vi "nanocal -- nuclear schottky fit V3.vi"() -> ()   [LabVIEW 2020]
uses:
  filename-pattern.ctl
  show-win- control.ctl
  cursor winow.ctl
  nanocal-goodness-weighting-strategy.ctl
  <vilib>/gmath/NumericalOptimization/stopping criteria.ctl
  3-lorentzian-parameters.ctl
  cursor window action.ctl
  3-lorentzian-heat-response action.ctl
  cursor action.ctl
  2Dwindow.ctl
  publisher action.ctl
  mathematica string map action.ctl
  <vilib>/gmath/NumericalOptimization/objective function data.ctl
  3-lorentzian-parameters -- action.ctl
  filename-action.ctl
  <vilib>/Utility/miscctls.llb/LVMapReplaceAction.ctl
  file -- read-write control.ctl
  array -- freq-voltage transformations action.ctl
  KM_file -- read-write control.ctl
  replace cursor action stack.vi
  Q -- range multiplier -- real -- V2.vi
  Q - not nan and gtr than zero - Real.vi
  Q - not nan -- real.vi
  Q -- check range -- i -- real.vi
  array - smart min max.vi
  3-lorentzian-heat-response -- V4.vi/142dd4c5-f9ed-c64b-bc14-a88e3e2c450a.vi
  3-lorentzian-heat-response -- analytic derivatives V3.vi
  array -- integrate scalar product.vi
  3-lorentzian-heat-response -- analytic derivatives -- grad and curvature -- V4.vi
  array -- freq-voltage transformations.vi/05c44075-957c-bc42-b6fa-2799d0bc0485.vi
  tale of three indices.vi
  filter -- window span logic.vi
  linear interp iiii- complex - z-omega - divide.vi
  linear interpolation iiii- complex.vi
  containing bix.vi
  3-lorentzian-heat-response.vi/142dd4c5-f9ed-c64b-bc14-a88e3e2c450a.vi
  <vilib>/Array/Sort 2D Array - Pop Stack.vi
  <vilib>/Array/Sort 2D Array - Push Stack.vi
  array -- freq-voltage transformations.vi/05c44075-957c-bc42-b6fa-2799d0bc0485.vi/5dd0d2be-718e-c148-b8fa-e083cdba2843.vi
  array -- freq-voltage transformations.vi/05c44075-957c-bc42-b6fa-2799d0bc0485.vi/095795a0-771d-c341-9fed-d90d2e44c51c.vi
  command stack.vi
  tale of three indices -- check state.vi
  Q -- check range -- i -- integer.vi
  linear interp iiii- complex - z-omega.vi
  line -- complex.vi
  Q - not nan -- integer.vi
  <vilib>/Analysis/baseanly.llb/A x B.vi
  <vilib>/Analysis/baseanly.llb/Complex A x B.vi
  array -- 3-finitediff.vi
  <vilib>/Analysis/polynomials.llb/Multiply Polynomials.vi
  <vilib>/Analysis/polynomials.llb/Multiply Polynomials (DBL).vi
  <vilib>/Analysis/polynomials.llb/Polynomial Roots.vi
  <vilib>/Analysis/polynomials.llb/Polynomial Roots (DBL).vi
  <vilib>/gmath/NumericalOptimization/Quasi Newton.vi
  <vilib>/Analysis/Matrix/Numeric/Conversions/Array To Matrix.vi
  <vilib>/Analysis/Matrix/Numeric/Conversions/Array To Matrix - RA2.vi
  <vilib>/Analysis/baseanly.llb/Inverse Matrix.vi
  <vilib>/Analysis/baseanly.llb/Real Inverse Matrix.vi
  <vilib>/Comparison/Less/Less Functor/Less Functor.lvclass
  <vilib>/gmath/NI_Gmath.lvlib
panel:
  in  "Map OUT":map{T1, dbl}(c390)
  in  "strings stuff tab":T2(tab)
  in  "string IN":string="  48 ->   <| \"ζ\"->  0.218787747977  , \"τ1\"-> 0.031456659327  , \"τS\"-> 0.269139973017  , \"τN\"-> 0.256714789857  , \"τC\"-> 0.001257909269  , \"κ0\"-> 0.000000000759  , \"mm1\"-> 0.000225096911  , \"mm2\"-> 0.015739660310  , \"mm3\"-> 0.657655153581  , \"T\"->  0.148000000000  , \"B\"-> 12.000000000000  , \"θ\"-> 0.000000000000  |>   , \r49 ->   <| \"ζ\"->  0.166979764431  , \"τ1\"-> 0.018942043621  , \"τS\"-> 0.110758885907  , \"τN\"-> 0.187535940807  , \"τC\"-> 0.001145519942  , \"κ0\"-> 0.000000001049  , \"mm1\"-> 0.000162653882  , \"mm2\"-> 0.006830646180  , \"mm3\"-> 0.361198290111  , \"T\"->  0.179000000000  , \"B\"-> 12.000000000000  , \"θ\"-> 0.000000000000  |>   , \r50 ->   <| \"ζ\"->  0.129670961314  , \"τ1\"-> 0.021089937696  , \"τS\"-> 0.112692124493  , \"τN\"-> 0.107228011320  , \"τC\"-> 0.001403544000  , \"κ0\"-> 0.000000001212  , \"mm1\"-> 0.000159537518  , \"mm2\"-> 0.010413685343  , \"mm3\"-> 0.260357650071  , \"T\"->  0.197000000000  , \"B\"-> 12.000000000000  , \"θ\"-> 0.000000000000  |>   , \r51 ->   <| \"ζ\"->  0.079034359832  , \"τ1\"-> 0.025346839295  , \"τS\"-> 0.089984085428  , \"τN\"-> 0.031717364329  , \"τC\"-> 0.001567096624  , \"κ0\"-> 0.000000001542  , \"mm1\"-> 0.000113086552  , \"mm2\"-> 0.017802249564  , \"mm3\"-> 0.140318645732  , \"T\"->  0.250000000000  , \"B\"-> 12.000000000000  , \"θ\"-> 0.000000000000  |>   , \r52 ->   <| \"ζ\"->  0.054397810218  , \"τ1\"-> 0.023191672440  , \"τS\"-> 0.068776102177  , \"τN\"-> 0.016667714610  , \"τC\"-> 0.001951070520  , \"κ0\"-> 0.000000001955  , \"mm1\"-> 0.000098147963  , \"mm2\"-> 0.017702409099  , \"mm3\"-> 0.097433959215  , \"T\"->  0.300000000000  , \"B\"-> 12.000000000000  , \"θ\"-> 0.000000000000  |>   , \r53 ->   <| \"ζ\"->  0.039475039748  , \"τ1\"-> 0.021602230815  , \"τS\"-> 0.055852925082  , \"τN\"-> 0.008163813050  , \"τC\"-> 0.002520091738  , \"κ0\"-> 0.000000002417  , \"mm1\"-> 0.000091858515  , \"mm2\"-> 0.018006002388  , \"mm3\"-> 0.072568263064  , \"T\"->  0.360000000000  , \"B\"-> 12.000000000000  , \"θ\"-> 0.000000000000  |>   , \r54 ->   <| \"ζ\"->  0.031945976845  , \"τ1\"-> 0.019000922826  , \"τS\"-> 0.045624146388  , \"τN\"-> 0.005314716063  , \"τC\"-> 0.002488383471  , \"κ0\"-> 0.000000002954  , \"mm1\"-> 0.000073272643  , \"mm2\"-> 0.016306894362  , \"mm3\"-> 0.057675293464  , \"T\"->  0.430000000000  , \"B\"-> 12.000000000000  , \"θ\"-> 0.000000000000  |>   , \r55 ->   <| \"ζ\"->  0.023031239946  , \"τ1\"-> 0.018268814012  , \"τS\"-> 0.037269400776  , \"τN\"-> 0.002696792890  , \"τC\"-> 0.003257395394  , \"κ0\"-> 0.000000003720  , \"mm1\"-> 0.000067670174  , \"mm2\"-> 0.016445281937  , \"mm3\"-> 0.045899921957  , \"T\"->  0.512000000000  , \"B\"-> 12.000000000000  , \"θ\"-> 0.000000000000  |>   , \r56 ->   <| \"ζ\"->  0.019920170845  , \"τ1\"-> 0.016368892412  , \"τS\"-> 0.030579536580  , \"τN\"-> 0.001736017565  , \"τC\"-> 0.004971418152  , \"κ0\"-> 0.000000004410  , \"mm1\"-> 0.000083939556  , \"mm2\"-> 0.015095997595  , \"mm3\"-> 0.039119658918  , \"T\"->  0.610000000000  , \"B\"-> 12.000000000000  , \"θ\"-> 0.000000000000  |>   , \r57 ->   <| \"ζ\"->  0.017558473054  , \"τ1\"-> 0.014545104284  , \"τS\"-> 0.022979681288  , \"τN\"-> 0.000840829385  , \"τC\"-> 0.005228030240  , \"κ0\"-> 0.000000006068  , \"mm1\"-> 0.000073916527  , \"mm2\"-> 0.013750428362  , \"mm3\"-> 0.030187552103  , \"T\"->  0.810000000000  , \"B\"-> 12.000000000000  , \"θ\"-> 0.000000000000  |>   , \r58 ->   <| \"ζ\"->  0.011916480594  , \"τ1\"-> 0.012551282481  , \"τS\"-> 0.018233218660  , \"τN\"-> 0.000345702746  , \"τC\"-> 0.004699451527  , \"κ0\"-> 0.000000008451  , \"mm1\"-> 0.000044190864  , \"mm2\"-> 0.012162820727  , \"mm3\"-> 0.023844039179  , \"T\"->  1.120000000000  , \"B\"-> 12.000000000000  , \"θ\"-> 0.000000000000  |>   , \r59 ->   <| \"ζ\"->  0.012831327568  , \"τ1\"-> 0.013315909415  , \"τS\"-> 0.012590836847  , \"τN\"-> 0.000065003013  , \"τC\"-> 0.005276356243  , \"κ0\"-> 0.000000013610  , \"mm1\"-> 0.000047406274  , \"mm2\"-> 0.013137605540  , \"mm3\"-> 0.018225484932  , \"T\"->  1.800000000000  , \"B\"-> 12.000000000000  , \"θ\"-> 0.000000000000  |>   , \r60 ->   <| \"ζ\"->  0.019774146838  , \"τ1\"-> 0.013257273421  , \"τS\"-> 0.007064131508  , \"τN\"-> 0.000028000819  , \"τC\"-> 0.006942241845  , \"κ0\"-> 0.000000023477  , \"mm1\"-> 0.000068886863  , \"mm2\"-> 0.012935419574  , \"mm3\"-> 0.014427582022  , \"T\"->  3.000000000000  , \"B\"-> 12.000000000000  , \"θ\"-> 0.000000000000  |>   , \r61 ->   <| \"ζ\"->  0.029251354442  , \"τ1\"-> 0.014634751206  , \"τS\"-> 0.003873958746  , \"τN\"-> 0.000007000487  , \"τC\"-> 0.006827504775  , \"κ0\"-> 0.000000056438  , \"mm1\"-> 0.000072018576  , \"mm2\"-> 0.010723236476  , \"mm3\"-> 0.014661483476  , \"T\"->  5.500000000000  , \"B\"-> 12.000000000000  , \"θ\"-> 0.000000000000  |>   , \r70 ->   <| \"ζ\"->  0.160194284670  , \"τ1\"-> 0.072790516188  , \"τS\"-> 0.045092589839  , \"τN\"-> 0.161618119718  , \"τC\"-> 0.001523160685  , \"κ0\"-> 0.000000001042  , \"mm1\"-> 0.000205091024  , \"mm2\"-> 0.012975392154  , \"mm3\"-> 0.300957777503  , \"T\"->  0.179000000000  , \"B\"-> 12.000000000000  , \"θ\"-> 90.000000000000  |>   , \r71 ->   <| \"ζ\"->  0.317192968490  , \"τ1\"-> 0.095324848000  , \"τS\"-> 0.087097785701  , \"τN\"-> 0.936221653169  , \"τC\"-> 0.001480807262  , \"κ0\"-> 0.000000000534  , \"mm1\"-> 0.000352978450  , \"mm2\"-> 0.007690057134  , \"mm3\"-> 1.436671789077  , \"T\"->  0.120000000000  , \"B\"-> 12.000000000000  , \"θ\"-> 90.000000000000  |>   , \r72 ->   <| \"ζ\"->  0.214326066797  , \"τ1\"-> 0.094995759328  , \"τS\"-> 0.077012716798  , \"τN\"-> 0.365142947332  , \"τC\"-> 0.001579379527  , \"κ0\"-> 0.000000000781  , \"mm1\"-> 0.000274869552  , \"mm2\"-> 0.014562991419  , \"mm3\"-> 0.618658426419  , \"T\"->  0.148000000000  , \"B\"-> 12.000000000000  , \"θ\"-> 90.000000000000  |>   , \r73 ->   <| \"ζ\"->  0.136975374218  , \"τ1\"-> 0.070969356603  , \"τS\"-> 0.041937456488  , \"τN\"-> 0.122985136767  , \"τC\"-> 0.001568280930  , \"κ0\"-> 0.000000001212  , \"mm1\"-> 0.000183564552  , \"mm2\"-> 0.014176261244  , \"mm3\"-> 0.245690738920  , \"T\"->  0.197000000000  , \"B\"-> 12.000000000000  , \"θ\"-> 90.000000000000  |>   , \r74 ->   <| \"ζ\"->  0.081038743925  , \"τ1\"-> 0.054864856987  , \"τS\"-> 0.033961002119  , \"τN\"-> 0.048653010594  , \"τC\"-> 0.001781381797  , \"κ0\"-> 0.000000001539  , \"mm1\"-> 0.000127765061  , \"mm2\"-> 0.016246990705  , \"mm3\"-> 0.129580431552  , \"T\"->  0.249000000000  , \"B\"-> 12.000000000000  , \"θ\"-> 90.000000000000  |>   , \r75 ->   <| \"ζ\"->  0.056185573597  , \"τ1\"-> 0.045207611912  , \"τS\"-> 0.029603026010  , \"τN\"-> 0.023507324547  , \"τC\"-> 0.002233080371  , \"κ0\"-> 0.000000001957  , \"mm1\"-> 0.000111229220  , \"mm2\"-> 0.017586614089  , \"mm3\"-> 0.085837235040  , \"T\"->  0.300000000000  , \"B\"-> 12.000000000000  , \"θ\"-> 90.000000000000  |>   , \r76 ->   <| \"ζ\"->  0.041794370964  , \"τ1\"-> 0.038862739492  , \"τS\"-> 0.026705422753  , \"τN\"-> 0.013514328703  , \"τC\"-> 0.002820386983  , \"κ0\"-> 0.000000002373  , \"mm1\"-> 0.000103067276  , \"mm2\"-> 0.018175730335  , \"mm3\"-> 0.065305039533  , \"T\"->  0.360000000000  , \"B\"-> 12.000000000000  , \"θ\"-> 90.000000000000  |>   , \r77 ->   <| \"ζ\"->  0.033296236595  , \"τ1\"-> 0.031336126456  , \"τS\"-> 0.024496257026  , \"τN\"-> 0.007027117109  , \"τC\"-> 0.002825302830  , \"κ0\"-> 0.000000002954  , \"mm1\"-> 0.000082132803  , \"mm2\"-> 0.018113321458  , \"mm3\"-> 0.048538958884  , \"T\"->  0.430000000000  , \"B\"-> 12.000000000000  , \"θ\"-> 90.000000000000  |>   , \r78 ->   <| \"ζ\"->  0.027144402160  , \"τ1\"-> 0.026090960664  , \"τS\"-> 0.022078937790  , \"τN\"-> 0.003827547658  , \"τC\"-> 0.003825438719  , \"κ0\"-> 0.000000003686  , \"mm1\"-> 0.000086780474  , \"mm2\"-> 0.017873160725  , \"mm3\"-> 0.038566159691  , \"T\"->  0.512000000000  , \"B\"-> 12.000000000000  , \"θ\"-> 90.000000000000  |>   , \r79 ->   <| \"ζ\"->  0.020263859818  , \"τ1\"-> 0.022629231163  , \"τS\"-> 0.021062454034  , \"τN\"-> 0.002238399470  , \"τC\"-> 0.004128602745  , \"κ0\"-> 0.000000004397  , \"mm1\"-> 0.000068966735  , \"mm2\"-> 0.017587727761  , \"mm3\"-> 0.032874158145  , \"T\"->  0.610000000000  , \"B\"-> 12.000000000000  , \"θ\"-> 90.000000000000  |>   , \r80 ->   <| \"ζ\"->  0.014774082145  , \"τ1\"-> 0.015773102766  , \"τS\"-> 0.018723894921  , \"τN\"-> 0.000790199963  , \"τC\"-> 0.005097561693  , \"κ0\"-> 0.000000006095  , \"mm1\"-> 0.000058657119  , \"mm2\"-> 0.014545814994  , \"mm3\"-> 0.026068590072  , \"T\"->  0.810000000000  , \"B\"-> 12.000000000000  , \"θ\"-> 90.000000000000  |>   , \r81 ->   <| \"ζ\"->  0.014230278097  , \"τ1\"-> 0.016181489886  , \"τS\"-> 0.016832346578  , \"τN\"-> 0.000327070958  , \"τC\"-> 0.005559720416  , \"κ0\"-> 0.000000008431  , \"mm1\"-> 0.000058995908  , \"mm2\"-> 0.015461166696  , \"mm3\"-> 0.023624648518  , \"T\"->  1.100000000000  , \"B\"-> 12.000000000000  , \"θ\"-> 90.000000000000  |>   , \r82 ->   <| \"ζ\"->  0.014703834330  , \"τ1\"-> 0.019025451961  , \"τS\"-> 0.011790469569  , \"τN\"-> 0.000107003492  , \"τC\"-> 0.007625608278  , \"κ0\"-> 0.000000014259  , \"mm1\"-> 0.000067719319  , \"mm2\"-> 0.017860728495  , \"mm3\"-> 0.020795023959  , \"T\"->  1.800000000000  , \"B\"-> 12.000000000000  , \"θ\"-> 90.000000000000  |>   , \r83 ->   <| \"ζ\"->  0.021950059397  , \"τ1\"-> 0.019029879523  , \"τS\"-> 0.006582834729  , \"τN\"-> 0.000028012011  , \"τC\"-> 0.009051896214  , \"κ0\"-> 0.000000024750  , \"mm1\"-> 0.000083329251  , \"mm2\"-> 0.015568079914  , \"mm3\"-> 0.019186321790  , \"T\"->  3.000000000000  , \"B\"-> 12.000000000000  , \"θ\"-> 90.000000000000  |>   , \r84 ->   <| \"ζ\"->  0.027897403691  , \"τ1\"-> 0.014639690770  , \"τS\"-> 0.004105291179  , \"τN\"-> 0.000006999171  , \"τC\"-> 0.007414449545  , \"κ0\"-> 0.000000059701  , \"mm1\"-> 0.000073450671  , \"mm2\"-> 0.011534391407  , \"mm3\"-> 0.014673310811  , \"T\"->  5.700000000000  , \"B\"-> 12.000000000000  , \"θ\"-> 90.000000000000  |>   , \r"
  in  "math -->   τ's !":bool
  in  "τ's --> math!":bool
  out "string OUT":string="  48 ->   <| \"ζ\"->  0.218787747977  , \"τ1\"-> 0.031456659327  , \"τS\"-> 0.269139973017  , \"τN\"-> 0.256714789857  , \"τC\"-> 0.001257909269  , \"κ0\"-> 0.000000000759  , \"mm1\"-> 0.000225096911  , \"mm2\"-> 0.015739660310  , \"mm3\"-> 0.657655153581  , \"T\"->  0.148000000000  , \"B\"-> 12.000000000000  , \"θ\"-> 0.000000000000  |>   , \r49 ->   <| \"ζ\"->  0.166979764431  , \"τ1\"-> 0.018942043621  , \"τS\"-> 0.110758885907  , \"τN\"-> 0.187535940807  , \"τC\"-> 0.001145519942  , \"κ0\"-> 0.000000001049  , \"mm1\"-> 0.000162653882  , \"mm2\"-> 0.006830646180  , \"mm3\"-> 0.361198290111  , \"T\"->  0.179000000000  , \"B\"-> 12.000000000000  , \"θ\"-> 0.000000000000  |>   , \r50 ->   <| \"ζ\"->  0.129670961314  , \"τ1\"-> 0.021089937696  , \"τS\"-> 0.112692124493  , \"τN\"-> 0.107228011320  , \"τC\"-> 0.001403544000  , \"κ0\"-> 0.000000001212  , \"mm1\"-> 0.000159537518  , \"mm2\"-> 0.010413685343  , \"mm3\"-> 0.260357650071  , \"T\"->  0.197000000000  , \"B\"-> 12.000000000000  , \"θ\"-> 0.000000000000  |>   , \r51 ->   <| \"ζ\"->  0.079034359832  , \"τ1\"-> 0.025346839295  , \"τS\"-> 0.089984085428  , \"τN\"-> 0.031717364329  , \"τC\"-> 0.001567096624  , \"κ0\"-> 0.000000001542  , \"mm1\"-> 0.000113086552  , \"mm2\"-> 0.017802249564  , \"mm3\"-> 0.140318645732  , \"T\"->  0.250000000000  , \"B\"-> 12.000000000000  , \"θ\"-> 0.000000000000  |>   , \r52 ->   <| \"ζ\"->  0.054397810218  , \"τ1\"-> 0.023191672440  , \"τS\"-> 0.068776102177  , \"τN\"-> 0.016667714610  , \"τC\"-> 0.001951070520  , \"κ0\"-> 0.000000001955  , \"mm1\"-> 0.000098147963  , \"mm2\"-> 0.017702409099  , \"mm3\"-> 0.097433959215  , \"T\"->  0.300000000000  , \"B\"-> 12.000000000000  , \"θ\"-> 0.000000000000  |>   , \r53 ->   <| \"ζ\"->  0.039475039748  , \"τ1\"-> 0.021602230815  , \"τS\"-> 0.055852925082  , \"τN\"-> 0.008163813050  , \"τC\"-> 0.002520091738  , \"κ0\"-> 0.000000002417  , \"mm1\"-> 0.000091858515  , \"mm2\"-> 0.018006002388  , \"mm3\"-> 0.072568263064  , \"T\"->  0.360000000000  , \"B\"-> 12.000000000000  , \"θ\"-> 0.000000000000  |>   , \r54 ->   <| \"ζ\"->  0.031945976845  , \"τ1\"-> 0.019000922826  , \"τS\"-> 0.045624146388  , \"τN\"-> 0.005314716063  , \"τC\"-> 0.002488383471  , \"κ0\"-> 0.000000002954  , \"mm1\"-> 0.000073272643  , \"mm2\"-> 0.016306894362  , \"mm3\"-> 0.057675293464  , \"T\"->  0.430000000000  , \"B\"-> 12.000000000000  , \"θ\"-> 0.000000000000  |>   , \r55 ->   <| \"ζ\"->  0.023031239946  , \"τ1\"-> 0.018268814012  , \"τS\"-> 0.037269400776  , \"τN\"-> 0.002696792890  , \"τC\"-> 0.003257395394  , \"κ0\"-> 0.000000003720  , \"mm1\"-> 0.000067670174  , \"mm2\"-> 0.016445281937  , \"mm3\"-> 0.045899921957  , \"T\"->  0.512000000000  , \"B\"-> 12.000000000000  , \"θ\"-> 0.000000000000  |>   , \r56 ->   <| \"ζ\"->  0.019920170845  , \"τ1\"-> 0.016368892412  , \"τS\"-> 0.030579536580  , \"τN\"-> 0.001736017565  , \"τC\"-> 0.004971418152  , \"κ0\"-> 0.000000004410  , \"mm1\"-> 0.000083939556  , \"mm2\"-> 0.015095997595  , \"mm3\"-> 0.039119658918  , \"T\"->  0.610000000000  , \"B\"-> 12.000000000000  , \"θ\"-> 0.000000000000  |>   , \r57 ->   <| \"ζ\"->  0.017558473054  , \"τ1\"-> 0.014545104284  , \"τS\"-> 0.022979681288  , \"τN\"-> 0.000840829385  , \"τC\"-> 0.005228030240  , \"κ0\"-> 0.000000006068  , \"mm1\"-> 0.000073916527  , \"mm2\"-> 0.013750428362  , \"mm3\"-> 0.030187552103  , \"T\"->  0.810000000000  , \"B\"-> 12.000000000000  , \"θ\"-> 0.000000000000  |>   , \r58 ->   <| \"ζ\"->  0.011916480594  , \"τ1\"-> 0.012551282481  , \"τS\"-> 0.018233218660  , \"τN\"-> 0.000345702746  , \"τC\"-> 0.004699451527  , \"κ0\"-> 0.000000008451  , \"mm1\"-> 0.000044190864  , \"mm2\"-> 0.012162820727  , \"mm3\"-> 0.023844039179  , \"T\"->  1.120000000000  , \"B\"-> 12.000000000000  , \"θ\"-> 0.000000000000  |>   , \r59 ->   <| \"ζ\"->  0.012831327568  , \"τ1\"-> 0.013315909415  , \"τS\"-> 0.012590836847  , \"τN\"-> 0.000065003013  , \"τC\"-> 0.005276356243  , \"κ0\"-> 0.000000013610  , \"mm1\"-> 0.000047406274  , \"mm2\"-> 0.013137605540  , \"mm3\"-> 0.018225484932  , \"T\"->  1.800000000000  , \"B\"-> 12.000000000000  , \"θ\"-> 0.000000000000  |>   , \r60 ->   <| \"ζ\"->  0.019774146838  , \"τ1\"-> 0.013257273421  , \"τS\"-> 0.007064131508  , \"τN\"-> 0.000028000819  , \"τC\"-> 0.006942241845  , \"κ0\"-> 0.000000023477  , \"mm1\"-> 0.000068886863  , \"mm2\"-> 0.012935419574  , \"mm3\"-> 0.014427582022  , \"T\"->  3.000000000000  , \"B\"-> 12.000000000000  , \"θ\"-> 0.000000000000  |>   , \r61 ->   <| \"ζ\"->  0.029251354442  , \"τ1\"-> 0.014634751206  , \"τS\"-> 0.003873958746  , \"τN\"-> 0.000007000487  , \"τC\"-> 0.006827504775  , \"κ0\"-> 0.000000056438  , \"mm1\"-> 0.000072018576  , \"mm2\"-> 0.010723236476  , \"mm3\"-> 0.014661483476  , \"T\"->  5.500000000000  , \"B\"-> 12.000000000000  , \"θ\"-> 0.000000000000  |>   , \r70 ->   <| \"ζ\"->  0.160194284670  , \"τ1\"-> 0.072790516188  , \"τS\"-> 0.045092589839  , \"τN\"-> 0.161618119718  , \"τC\"-> 0.001523160685  , \"κ0\"-> 0.000000001042  , \"mm1\"-> 0.000205091024  , \"mm2\"-> 0.012975392154  , \"mm3\"-> 0.300957777503  , \"T\"->  0.179000000000  , \"B\"-> 12.000000000000  , \"θ\"-> 90.000000000000  |>   , \r71 ->   <| \"ζ\"->  0.317192968490  , \"τ1\"-> 0.095324848000  , \"τS\"-> 0.087097785701  , \"τN\"-> 0.936221653169  , \"τC\"-> 0.001480807262  , \"κ0\"-> 0.000000000534  , \"mm1\"-> 0.000352978450  , \"mm2\"-> 0.007690057134  , \"mm3\"-> 1.436671789077  , \"T\"->  0.120000000000  , \"B\"-> 12.000000000000  , \"θ\"-> 90.000000000000  |>   , \r72 ->   <| \"ζ\"->  0.214326066797  , \"τ1\"-> 0.094995759328  , \"τS\"-> 0.077012716798  , \"τN\"-> 0.365142947332  , \"τC\"-> 0.001579379527  , \"κ0\"-> 0.000000000781  , \"mm1\"-> 0.000274869552  , \"mm2\"-> 0.014562991419  , \"mm3\"-> 0.618658426419  , \"T\"->  0.148000000000  , \"B\"-> 12.000000000000  , \"θ\"-> 90.000000000000  |>   , \r73 ->   <| \"ζ\"->  0.136975374218  , \"τ1\"-> 0.070969356603  , \"τS\"-> 0.041937456488  , \"τN\"-> 0.122985136767  , \"τC\"-> 0.001568280930  , \"κ0\"-> 0.000000001212  , \"mm1\"-> 0.000183564552  , \"mm2\"-> 0.014176261244  , \"mm3\"-> 0.245690738920  , \"T\"->  0.197000000000  , \"B\"-> 12.000000000000  , \"θ\"-> 90.000000000000  |>   , \r74 ->   <| \"ζ\"->  0.081038743925  , \"τ1\"-> 0.054864856987  , \"τS\"-> 0.033961002119  , \"τN\"-> 0.048653010594  , \"τC\"-> 0.001781381797  , \"κ0\"-> 0.000000001539  , \"mm1\"-> 0.000127765061  , \"mm2\"-> 0.016246990705  , \"mm3\"-> 0.129580431552  , \"T\"->  0.249000000000  , \"B\"-> 12.000000000000  , \"θ\"-> 90.000000000000  |>   , \r75 ->   <| \"ζ\"->  0.056185573597  , \"τ1\"-> 0.045207611912  , \"τS\"-> 0.029603026010  , \"τN\"-> 0.023507324547  , \"τC\"-> 0.002233080371  , \"κ0\"-> 0.000000001957  , \"mm1\"-> 0.000111229220  , \"mm2\"-> 0.017586614089  , \"mm3\"-> 0.085837235040  , \"T\"->  0.300000000000  , \"B\"-> 12.000000000000  , \"θ\"-> 90.000000000000  |>   , \r76 ->   <| \"ζ\"->  0.041794370964  , \"τ1\"-> 0.038862739492  , \"τS\"-> 0.026705422753  , \"τN\"-> 0.013514328703  , \"τC\"-> 0.002820386983  , \"κ0\"-> 0.000000002373  , \"mm1\"-> 0.000103067276  , \"mm2\"-> 0.018175730335  , \"mm3\"-> 0.065305039533  , \"T\"->  0.360000000000  , \"B\"-> 12.000000000000  , \"θ\"-> 90.000000000000  |>   , \r77 ->   <| \"ζ\"->  0.033296236595  , \"τ1\"-> 0.031336126456  , \"τS\"-> 0.024496257026  , \"τN\"-> 0.007027117109  , \"τC\"-> 0.002825302830  , \"κ0\"-> 0.000000002954  , \"mm1\"-> 0.000082132803  , \"mm2\"-> 0.018113321458  , \"mm3\"-> 0.048538958884  , \"T\"->  0.430000000000  , \"B\"-> 12.000000000000  , \"θ\"-> 90.000000000000  |>   , \r78 ->   <| \"ζ\"->  0.027144402160  , \"τ1\"-> 0.026090960664  , \"τS\"-> 0.022078937790  , \"τN\"-> 0.003827547658  , \"τC\"-> 0.003825438719  , \"κ0\"-> 0.000000003686  , \"mm1\"-> 0.000086780474  , \"mm2\"-> 0.017873160725  , \"mm3\"-> 0.038566159691  , \"T\"->  0.512000000000  , \"B\"-> 12.000000000000  , \"θ\"-> 90.000000000000  |>   , \r79 ->   <| \"ζ\"->  0.020263859818  , \"τ1\"-> 0.022629231163  , \"τS\"-> 0.021062454034  , \"τN\"-> 0.002238399470  , \"τC\"-> 0.004128602745  , \"κ0\"-> 0.000000004397  , \"mm1\"-> 0.000068966735  , \"mm2\"-> 0.017587727761  , \"mm3\"-> 0.032874158145  , \"T\"->  0.610000000000  , \"B\"-> 12.000000000000  , \"θ\"-> 90.000000000000  |>   , \r80 ->   <| \"ζ\"->  0.014774082145  , \"τ1\"-> 0.015773102766  , \"τS\"-> 0.018723894921  , \"τN\"-> 0.000790199963  , \"τC\"-> 0.005097561693  , \"κ0\"-> 0.000000006095  , \"mm1\"-> 0.000058657119  , \"mm2\"-> 0.014545814994  , \"mm3\"-> 0.026068590072  , \"T\"->  0.810000000000  , \"B\"-> 12.000000000000  , \"θ\"-> 90.000000000000  |>   , \r81 ->   <| \"ζ\"->  0.014230278097  , \"τ1\"-> 0.016181489886  , \"τS\"-> 0.016832346578  , \"τN\"-> 0.000327070958  , \"τC\"-> 0.005559720416  , \"κ0\"-> 0.000000008431  , \"mm1\"-> 0.000058995908  , \"mm2\"-> 0.015461166696  , \"mm3\"-> 0.023624648518  , \"T\"->  1.100000000000  , \"B\"-> 12.000000000000  , \"θ\"-> 90.000000000000  |>   , \r82 ->   <| \"ζ\"->  0.014703834330  , \"τ1\"-> 0.019025451961  , \"τS\"-> 0.011790469569  , \"τN\"-> 0.000107003492  , \"τC\"-> 0.007625608278  , \"κ0\"-> 0.000000014259  , \"mm1\"-> 0.000067719319  , \"mm2\"-> 0.017860728495  , \"mm3\"-> 0.020795023959  , \"T\"->  1.800000000000  , \"B\"-> 12.000000000000  , \"θ\"-> 90.000000000000  |>   , \r83 ->   <| \"ζ\"->  0.021950059397  , \"τ1\"-> 0.019029879523  , \"τS\"-> 0.006582834729  , \"τN\"-> 0.000028012011  , \"τC\"-> 0.009051896214  , \"κ0\"-> 0.000000024750  , \"mm1\"-> 0.000083329251  , \"mm2\"-> 0.015568079914  , \"mm3\"-> 0.019186321790  , \"T\"->  3.000000000000  , \"B\"-> 12.000000000000  , \"θ\"-> 90.000000000000  |>   , \r84 ->   <| \"ζ\"->  0.027897403691  , \"τ1\"-> 0.014639690770  , \"τS\"-> 0.004105291179  , \"τN\"-> 0.000006999171  , \"τC\"-> 0.007414449545  , \"κ0\"-> 0.000000059701  , \"mm1\"-> 0.000073450671  , \"mm2\"-> 0.011534391407  , \"mm3\"-> 0.014673310811  , \"T\"->  5.700000000000  , \"B\"-> 12.000000000000  , \"θ\"-> 90.000000000000  |>   , \r"
  in  "math --> string!":bool
  in  "string --> math!":bool
  in  "file pattern":string="CeCoIn5_*_labview_.dat"
  in  "folder":path=path "/opt/new/Dropbox/shared_AkashAndreas/paper-CeCoIn5/labviewreadydata"
  in  "filenames":u16(ring)=11 caption="files" items=["CeCoIn5_2nd_071_12T_0.120K_90deg_fdep_labview_.dat", "CeCoIn5_2nd_048_12T_0.148K_0deg_freqDep_labview_.dat", "CeCoIn5_2nd_072_12T_0.148K_90deg_fdep_labview_.dat", "CeCoIn5_2nd_049_12T_0.179K_0deg_freqDep_labview_.dat", "CeCoIn5_2nd_070_12T_0.179K_90deg_fdep_labview_.dat", "CeCoIn5_2nd_050_12T_0.197K_0deg_freqDep_labview_.dat", "CeCoIn5_2nd_073_12T_0.197K_90deg_fdep_labview_.dat", "CeCoIn5_2nd_074_12T_0.249K_90deg_fdep_labview_.dat", "CeCoIn5_2nd_051_12T_0.25K_0deg_freqDep_labview_.dat", "CeCoIn5_2nd_052_12T_0.3K_0deg_freqDep_labview_.dat", "CeCoIn5_2nd_075_12T_0.300K_90deg_fdep_labview_.dat", "CeCoIn5_2nd_053_12T_0.360K_0deg_freqDep_labview_.dat", "CeCoIn5_2nd_076_12T_0.360K_90deg_fdep_labview_.dat", "CeCoIn5_2nd_054_12T_0.430K_0deg_freqDep_labview_.dat", "CeCoIn5_2nd_077_12T_0.430K_90deg_fdep_labview_.dat", "CeCoIn5_2nd_055_12T_0.512K_0deg_freqDep_labview_.dat", "CeCoIn5_2nd_078_12T_0.512K_90deg_fdep_labview_.dat", "CeCoIn5_2nd_056_12T_0.61K_0deg_freqDep_labview_.dat", "CeCoIn5_2nd_079_12T_0.610K_90deg_fdep_labview_.dat", "CeCoIn5_2nd_057_12T_0.81K_0deg_freqDep_labview_.dat", "CeCoIn5_2nd_080_12T_0.810K_90deg_fdep_labview_.dat", "CeCoIn5_2nd_081_12T_1.1K_90deg_fdep_labview_.dat", "CeCoIn5_2nd_058_12T_1.12K_0deg_freqDep_labview_.dat", "CeCoIn5_2nd_059_12T_1.8K_0deg_freqDep_labview_.dat", "CeCoIn5_2nd_082_12T_1.8K_90deg_fdep_labview_.dat", "CeCoIn5_2nd_060_12T_3.0K_0deg_freqDep_labview_.dat", "CeCoIn5_2nd_083_12T_3.0K_90deg_fdep_labview_.dat", "CeCoIn5_2nd_061_12T_5.5K_0deg_freqDep_labview_.dat", "CeCoIn5_2nd_084_12T_5.7K_90deg_fdep_labview_.dat"]
  out "notes":string="------------\n\n/opt/new/Dropbox/desktop_data/Indium-nanocal-cell12-June2021/labview-ready-files\nIndium_June2021_*_ark.dat\n\n---------------------\n/opt/new/Dropbox/shared_AkashAndreas/paper-CeCoIn5/labviewreadydata\nCeCoIn5_*_labview_.dat\n--------------------------------\n\n\n\n  48 ->   <| \"ζ\"-> 0.225182112153  , \"τ1\"-> 0.030427185371  , \"τS\"-> 0.215756406989  , \"τN\"-> 0.297516075068  , \"τC\"-> 0.001159880124  , \"κ0\"-> 0.000000000757  , \"T\"-> 0.148000000000  , \"mm1\"-> 0.000000000000  , \"mm2\"-> 0.000000000000  , \"mm3\"-> 0.000000000000  , \"θ\"-> 0.000000000000  |>   , \r49 ->   <| \"ζ\"-> 0.172076901868  , \"τ1\"-> 0.029034369734  , \"τS\"-> 0.155813864567  , \"τN\"-> 0.144653734876  , \"τC\"-> 0.001114471886  , \"κ0\"-> 0.000000001041  , \"T\"-> 0.179000000000  , \"mm1\"-> 0.000000000000  , \"mm2\"-> 0.000000000000  , \"mm3\"-> 0.000000000000  , \"θ\"-> 0.000000000000  |>   , \r50 ->   <| \"ζ\"-> 0.148077728243  , \"τ1\"-> 0.028544607399  , \"τS\"-> 0.124620640187  , \"τN\"-> 0.093757074751  , \"τC\"-> 0.001082877171  , \"κ0\"-> 0.000000001180  , \"T\"-> 0.197000000000  , \"mm1\"-> 0.000000000000  , \"mm2\"-> 0.000000000000  , \"mm3\"-> 0.000000000000  , \"θ\"-> 0.000000000000  |>   , \r51 ->   <| \"ζ\"-> 0.081193222097  , \"τ1\"-> 0.024715806431  , \"τS\"-> 0.089455978355  , \"τN\"-> 0.032053841538  , \"τC\"-> 0.001544599185  , \"κ0\"-> 0.000000001536  , \"T\"-> 0.250000000000  , \"mm1\"-> 0.000000000000  , \"mm2\"-> 0.000000000000  , \"mm3\"-> 0.000000000000  , \"θ\"-> 0.000000000000  |>   , \r52 ->   <| \"ζ\"-> 0.048082496373  , \"τ1\"-> 0.022642786515  , \"τS\"-> 0.068869549235  , \"τN\"-> 0.016486235683  , \"τC\"-> 0.002476229885  , \"κ0\"-> 0.000000001973  , \"T\"-> 0.300000000000  , \"mm1\"-> 0.000000000000  , \"mm2\"-> 0.000000000000  , \"mm3\"-> 0.000000000000  , \"θ\"-> 0.000000000000  |>   , \r53 ->   <| \"ζ\"-> 0.038407326202  , \"τ1\"-> 0.020371560008  , \"τS\"-> 0.055508745241  , \"τN\"-> 0.008451508810  , \"τC\"-> 0.002530832197  , \"κ0\"-> 0.000000002423  , \"T\"-> 0.360000000000  , \"mm1\"-> 0.000000000000  , \"mm2\"-> 0.000000000000  , \"mm3\"-> 0.000000000000  , \"θ\"-> 0.000000000000  |>   , \r54 ->   <| \"ζ\"-> 0.025817013343  , \"τ1\"-> 0.018385471103  , \"τS\"-> 0.045747558757  , \"τN\"-> 0.005165003032  , \"τC\"-> 0.002680275541  , \"κ0\"-> 0.000000002982  , \"T\"-> 0.430000000000  , \"mm1\"-> 0.000000000000  , \"mm2\"-> 0.000000000000  , \"mm3\"-> 0.000000000000  , \"θ\"-> 0.000000000000  |>   , \r55 ->   <| \"ζ\"-> 0.019908376980  , \"τ1\"-> 0.016902177597  , \"τS\"-> 0.037431350421  , \"τN\"-> 0.003115611581  , \"τC\"-> 0.002813000351  , \"κ0\"-> 0.000000003723  , \"T\"-> 0.512000000000  , \"mm1\"-> 0.000000000000  , \"mm2\"-> 0.000000000000  , \"mm3\"-> 0.000000000000  , \"θ\"-> 0.000000000000  |>   , \r56 ->   <| \"ζ\"-> 0.018376000000  , \"τ1\"-> 0.014989979497  , \"τS\"-> 0.031364970092  , \"τN\"-> 0.001876083588  , \"τC\"-> 0.004034409107  , \"κ0\"-> 0.000000004410  , \"T\"-> 0.610000000000  , \"mm1\"-> 0.000000000000  , \"mm2\"-> 0.000000000000  , \"mm3\"-> 0.000000000000  , \"θ\"-> 0.000000000000  |>   , \r57 ->   <| \"ζ\"-> 0.015651665128  , \"τ1\"-> 0.013298894889  , \"τS\"-> 0.022882494925  , \"τN\"-> 0.000826522678  , \"τC\"-> 0.005306542804  , \"κ0\"-> 0.000000006075  , \"T\"-> 0.810000000000  , \"mm1\"-> 0.000000000000  , \"mm2\"-> 0.000000000000  , \"mm3\"-> 0.000000000000  , \"θ\"-> 0.000000000000  |>   , \r58 ->   <| \"ζ\"-> 0.011916480594  , \"τ1\"-> 0.012551282481  , \"τS\"-> 0.018233218660  , \"τN\"-> 0.000345702746  , \"τC\"-> 0.004699451527  , \"κ0\"-> 0.000000008451  , \"T\"-> 1.120000000000  , \"mm1\"-> 0.000000000000  , \"mm2\"-> 0.000000000000  , \"mm3\"-> 0.000000000000  , \"θ\"-> 0.000000000000  |>   , \r59 ->   <| \"ζ\"-> 0.012831327568  , \"τ1\"-> 0.013315909415  , \"τS\"-> 0.012590836847  , \"τN\"-> 0.000065003013  , \"τC\"-> 0.005276356243  , \"κ0\"-> 0.000000013610  , \"T\"-> 1.800000000000  , \"mm1\"-> 0.000000000000  , \"mm2\"-> 0.000000000000  , \"mm3\"-> 0.000000000000  , \"θ\"-> 0.000000000000  |>   , \r60 ->   <| \"ζ\"-> 0.019774146838  , \"τ1\"-> 0.013257273421  , \"τS\"-> 0.007064131508  , \"τN\"-> 0.000028000819  , \"τC\"-> 0.006942241845  , \"κ0\"-> 0.000000023477  , \"T\"-> 3.000000000000  , \"mm1\"-> 0.000000000000  , \"mm2\"-> 0.000000000000  , \"mm3\"-> 0.000000000000  , \"θ\"-> 0.000000000000  |>   , \r61 ->   <| \"ζ\"-> 0.029251354442  , \"τ1\"-> 0.014634751206  , \"τS\"-> 0.003873958746  , \"τN\"-> 0.000007000487  , \"τC\"-> 0.006827504775  , \"κ0\"-> 0.000000056438  , \"T\"-> 5.500000000000  , \"mm1\"-> 0.000000000000  , \"mm2\"-> 0.000000000000  , \"mm3\"-> 0.000000000000  , \"θ\"-> 0.000000000000  |>   , \r70 ->   <| \"ζ\"-> 0.160286026344  , \"τ1\"-> 0.073452047785  , \"τS\"-> 0.044872374187  , \"τN\"-> 0.162076895387  , \"τC\"-> 0.001481759328  , \"κ0\"-> 0.000000001039  , \"T\"-> 0.179000000000  , \"mm1\"-> 0.000000000000  , \"mm2\"-> 0.000000000000  , \"mm3\"-> 0.000000000000  , \"θ\"-> 90.000000000000  |>   , \r71 ->   <| \"ζ\"-> 0.317192968490  , \"τ1\"-> 0.095324848000  , \"τS\"-> 0.087097785701  , \"τN\"-> 0.936221653169  , \"τC\"-> 0.001480807262  , \"κ0\"-> 0.000000000534  , \"T\"-> 0.120000000000  , \"mm1\"-> 0.000000000000  , \"mm2\"-> 0.000000000000  , \"mm3\"-> 0.000000000000  , \"θ\"-> 90.000000000000  |>   , \r72 ->   <| \"ζ\"-> 0.222764630124  , \"τ1\"-> 0.096058032825  , \"τS\"-> 0.066495942806  , \"τN\"-> 0.366151877245  , \"τC\"-> 0.001319275999  , \"κ0\"-> 0.000000000769  , \"T\"-> 0.148000000000  , \"mm1\"-> 0.000000000000  , \"mm2\"-> 0.000000000000  , \"mm3\"-> 0.000000000000  , \"θ\"-> 90.000000000000  |>   , \r73 ->   <| \"ζ\"-> 0.136082903087  , \"τ1\"-> 0.070214285183  , \"τS\"-> 0.041562366618  , \"τN\"-> 0.122478563978  , \"τC\"-> 0.001561716081  , \"κ0\"-> 0.000000001214  , \"T\"-> 0.197000000000  , \"mm1\"-> 0.000000000000  , \"mm2\"-> 0.000000000000  , \"mm3\"-> 0.000000000000  , \"θ\"-> 90.000000000000  |>   , \r74 ->   <| \"ζ\"-> 0.079924133870  , \"τ1\"-> 0.053892600038  , \"τS\"-> 0.033721986821  , \"τN\"-> 0.048194390820  , \"τC\"-> 0.001786420268  , \"κ0\"-> 0.000000001543  , \"T\"-> 0.249000000000  , \"mm1\"-> 0.000000000000  , \"mm2\"-> 0.000000000000  , \"mm3\"-> 0.000000000000  , \"θ\"-> 90.000000000000  |>   , \r75 ->   <| \"ζ\"-> 0.055680730504  , \"τ1\"-> 0.044845519236  , \"τS\"-> 0.029550773155  , \"τN\"-> 0.023428217313  , \"τC\"-> 0.002197475136  , \"κ0\"-> 0.000000001960  , \"T\"-> 0.300000000000  , \"mm1\"-> 0.000000000000  , \"mm2\"-> 0.000000000000  , \"mm3\"-> 0.000000000000  , \"θ\"-> 90.000000000000  |>   , \r76 ->   <| \"ζ\"-> 0.040648812263  , \"τ1\"-> 0.038083560479  , \"τS\"-> 0.026574795079  , \"τN\"-> 0.013361826633  , \"τC\"-> 0.002899405432  , \"κ0\"-> 0.000000002383  , \"T\"-> 0.360000000000  , \"mm1\"-> 0.000000000000  , \"mm2\"-> 0.000000000000  , \"mm3\"-> 0.000000000000  , \"θ\"-> 90.000000000000  |>   , \r77 ->   <| \"ζ\"-> 0.031873906103  , \"τ1\"-> 0.030223838950  , \"τS\"-> 0.024286132427  , \"τN\"-> 0.006926780152  , \"τC\"-> 0.002978043437  , \"κ0\"-> 0.000000002967  , \"T\"-> 0.430000000000  , \"mm1\"-> 0.000000000000  , \"mm2\"-> 0.000000000000  , \"mm3\"-> 0.000000000000  , \"θ\"-> 90.000000000000  |>   , \r78 ->   <| \"ζ\"-> 0.025948172116  , \"τ1\"-> 0.025051552712  , \"τS\"-> 0.022571188655  , \"τN\"-> 0.003812228812  , \"τC\"-> 0.003259730052  , \"κ0\"-> 0.000000003686  , \"T\"-> 0.512000000000  , \"mm1\"-> 0.000000000000  , \"mm2\"-> 0.000000000000  , \"mm3\"-> 0.000000000000  , \"θ\"-> 90.000000000000  |>   , \r79 ->   <| \"ζ\"-> 0.020946044060  , \"τ1\"-> 0.024756174566  , \"τS\"-> 0.021099556284  , \"τN\"-> 0.002276701384  , \"τC\"-> 0.004159440288  , \"κ0\"-> 0.000000004389  , \"T\"-> 0.610000000000  , \"mm1\"-> 0.000000000000  , \"mm2\"-> 0.000000000000  , \"mm3\"-> 0.000000000000  , \"θ\"-> 90.000000000000  |>   , \r80 ->   <| \"ζ\"-> 0.014774082145  , \"τ1\"-> 0.015773102766  , \"τS\"-> 0.018723894921  , \"τN\"-> 0.000790199963  , \"τC\"-> 0.005097561693  , \"κ0\"-> 0.000000006095  , \"T\"-> 0.810000000000  , \"mm1\"-> 0.000000000000  , \"mm2\"-> 0.000000000000  , \"mm3\"-> 0.000000000000  , \"θ\"-> 90.000000000000  |>   , \r81 ->   <| \"ζ\"-> 0.013971175207  , \"τ1\"-> 0.015831825440  , \"τS\"-> 0.017293056061  , \"τN\"-> 0.000406001835  , \"τC\"-> 0.005061653181  , \"κ0\"-> 0.000000008423  , \"T\"-> 1.100000000000  , \"mm1\"-> 0.000000000000  , \"mm2\"-> 0.000000000000  , \"mm3\"-> 0.000000000000  , \"θ\"-> 90.000000000000  |>   , \r82 ->   <| \"ζ\"-> 0.014703834330  , \"τ1\"-> 0.019025451961  , \"τS\"-> 0.011790469569  , \"τN\"-> 0.000107003492  , \"τC\"-> 0.007625608278  , \"κ0\"-> 0.000000014259  , \"T\"-> 1.800000000000  , \"mm1\"-> 0.000000000000  , \"mm2\"-> 0.000000000000  , \"mm3\"-> 0.000000000000  , \"θ\"-> 90.000000000000  |>   , \r83 ->   <| \"ζ\"-> 0.021950059397  , \"τ1\"-> 0.019029879523  , \"τS\"-> 0.006582834729  , \"τN\"-> 0.000028012011  , \"τC\"-> 0.009051896214  , \"κ0\"-> 0.000000024750  , \"T\"-> 3.000000000000  , \"mm1\"-> 0.000000000000  , \"mm2\"-> 0.000000000000  , \"mm3\"-> 0.000000000000  , \"θ\"-> 90.000000000000  |>   , \r84 ->   <| \"ζ\"-> 0.027897403691  , \"τ1\"-> 0.014639690770  , \"τS\"-> 0.004105291179  , \"τN\"-> 0.000006999171  , \"τC\"-> 0.007414449545  , \"κ0\"-> 0.000000059701  , \"T\"-> 5.700000000000  , \"mm1\"-> 0.000073450671  , \"mm2\"-> 0.014673310812  , \"mm3\"-> 0.011534391407  , \"θ\"-> 90.000000000000  |>   , \r"
  out "filenames":map{i32, string}(c390)={48="CeCoIn5_2nd_048_12T_0.148K_0deg_freqDep_labview_.dat", 49="CeCoIn5_2nd_049_12T_0.179K_0deg_freqDep_labview_.dat", 50="CeCoIn5_2nd_050_12T_0.197K_0deg_freqDep_labview_.dat", 51="CeCoIn5_2nd_051_12T_0.25K_0deg_freqDep_labview_.dat", 52="CeCoIn5_2nd_052_12T_0.3K_0deg_freqDep_labview_.dat", 53="CeCoIn5_2nd_053_12T_0.360K_0deg_freqDep_labview_.dat", 54="CeCoIn5_2nd_054_12T_0.430K_0deg_freqDep_labview_.dat", 55="CeCoIn5_2nd_055_12T_0.512K_0deg_freqDep_labview_.dat", 56="CeCoIn5_2nd_056_12T_0.61K_0deg_freqDep_labview_.dat", 57="CeCoIn5_2nd_057_12T_0.81K_0deg_freqDep_labview_.dat", 58="CeCoIn5_2nd_058_12T_1.12K_0deg_freqDep_labview_.dat", 59="CeCoIn5_2nd_059_12T_1.8K_0deg_freqDep_labview_.dat", 60="CeCoIn5_2nd_060_12T_3.0K_0deg_freqDep_labview_.dat", 61="CeCoIn5_2nd_061_12T_5.5K_0deg_freqDep_labview_.dat", 70="CeCoIn5_2nd_070_12T_0.179K_90deg_fdep_labview_.dat", 71="CeCoIn5_2nd_071_12T_0.120K_90deg_fdep_labview_.dat", 72="CeCoIn5_2nd_072_12T_0.148K_90deg_fdep_labview_.dat", 73="CeCoIn5_2nd_073_12T_0.197K_90deg_fdep_labview_.dat", 74="CeCoIn5_2nd_074_12T_0.249K_90deg_fdep_labview_.dat", 75="CeCoIn5_2nd_075_12T_0.300K_90deg_fdep_labview_.dat", 76="CeCoIn5_2nd_076_12T_0.360K_90deg_fdep_labview_.dat", 77="CeCoIn5_2nd_077_12T_0.430K_90deg_fdep_labview_.dat", 78="CeCoIn5_2nd_078_12T_0.512K_90deg_fdep_labview_.dat", 79="CeCoIn5_2nd_079_12T_0.610K_90deg_fdep_labview_.dat", 80="CeCoIn5_2nd_080_12T_0.810K_90deg_fdep_labview_.dat", 81="CeCoIn5_2nd_081_12T_1.1K_90deg_fdep_labview_.dat", 82="CeCoIn5_2nd_082_12T_1.8K_90deg_fdep_labview_.dat", 83="CeCoIn5_2nd_083_12T_3.0K_90deg_fdep_labview_.dat", 84="CeCoIn5_2nd_084_12T_5.7K_90deg_fdep_labview_.dat"}
  out "Set of B's":set{dbl}(c389)={12.0}
  out "Set of θ's":set{dbl}(c389)={0.0, 90.0}
  out "Set of T's":set{dbl}(c389)={0.12, 0.148, 0.179, 0.197, 0.249, 0.25, 0.3, 0.36, 0.43, 0.512, 0.61, 0.81, 1.1, 1.12, 1.8, 3.0, 5.5, 5.7}
  out "B lookup":map{i32, dbl}(c390)={0=12.0}
  out "filesnames lookup":map{i32, i32}(c390)={0=71, 1=48, 2=72, 3=49, 4=70, 5=50, 6=73, 7=74, 8=51, 9=52, 10=75, 11=53, 12=76, 13=54, 14=77, 15=55, 16=78, 17=56, 18=79, 19=57, 20=80, 21=81, 22=58, 23=59, 24=82, 25=60, 26=83, 27=61, 28=84}
  out "θ lookup":map{i32, dbl}(c390)={0=0.0, 1=90.0}
  out "T lookup":map{i32, dbl}(c390)={0=0.12, 1=0.148, 2=0.179, 3=0.197, 4=0.249, 5=0.25, 6=0.3, 7=0.36, 8=0.43, 9=0.512, 10=0.61, 11=0.81, 12=1.1, 13=1.12, 14=1.8, 15=3.0, 16=5.5, 17=5.7}
  out "backup mathematica string OUT backup":string="  48 ->   <| \"ζ\"-> 0.225182112153  , \"τ1\"-> 0.030427185371  , \"τS\"-> 0.215756406989  , \"τN\"-> 0.297516075068  , \"τC\"-> 0.001159880124  , \"κ0\"-> 0.000000000757  , \"T\"-> 0.148000000000  , \"mm1\"-> 0.000000000000  , \"mm2\"-> 0.000000000000  , \"mm3\"-> 0.000000000000  , \"θ\"-> 0.000000000000  |>   , \r49 ->   <| \"ζ\"-> 0.172076901868  , \"τ1\"-> 0.029034369734  , \"τS\"-> 0.155813864567  , \"τN\"-> 0.144653734876  , \"τC\"-> 0.001114471886  , \"κ0\"-> 0.000000001041  , \"T\"-> 0.179000000000  , \"mm1\"-> 0.000000000000  , \"mm2\"-> 0.000000000000  , \"mm3\"-> 0.000000000000  , \"θ\"-> 0.000000000000  |>   , \r50 ->   <| \"ζ\"-> 0.148077728243  , \"τ1\"-> 0.028544607399  , \"τS\"-> 0.124620640187  , \"τN\"-> 0.093757074751  , \"τC\"-> 0.001082877171  , \"κ0\"-> 0.000000001180  , \"T\"-> 0.197000000000  , \"mm1\"-> 0.000000000000  , \"mm2\"-> 0.000000000000  , \"mm3\"-> 0.000000000000  , \"θ\"-> 0.000000000000  |>   , \r51 ->   <| \"ζ\"-> 0.081193222097  , \"τ1\"-> 0.024715806431  , \"τS\"-> 0.089455978355  , \"τN\"-> 0.032053841538  , \"τC\"-> 0.001544599185  , \"κ0\"-> 0.000000001536  , \"T\"-> 0.250000000000  , \"mm1\"-> 0.000000000000  , \"mm2\"-> 0.000000000000  , \"mm3\"-> 0.000000000000  , \"θ\"-> 0.000000000000  |>   , \r52 ->   <| \"ζ\"-> 0.048082496373  , \"τ1\"-> 0.022642786515  , \"τS\"-> 0.068869549235  , \"τN\"-> 0.016486235683  , \"τC\"-> 0.002476229885  , \"κ0\"-> 0.000000001973  , \"T\"-> 0.300000000000  , \"mm1\"-> 0.000000000000  , \"mm2\"-> 0.000000000000  , \"mm3\"-> 0.000000000000  , \"θ\"-> 0.000000000000  |>   , \r53 ->   <| \"ζ\"-> 0.038407326202  , \"τ1\"-> 0.020371560008  , \"τS\"-> 0.055508745241  , \"τN\"-> 0.008451508810  , \"τC\"-> 0.002530832197  , \"κ0\"-> 0.000000002423  , \"T\"-> 0.360000000000  , \"mm1\"-> 0.000000000000  , \"mm2\"-> 0.000000000000  , \"mm3\"-> 0.000000000000  , \"θ\"-> 0.000000000000  |>   , \r54 ->   <| \"ζ\"-> 0.025817013343  , \"τ1\"-> 0.018385471103  , \"τS\"-> 0.045747558757  , \"τN\"-> 0.005165003032  , \"τC\"-> 0.002680275541  , \"κ0\"-> 0.000000002982  , \"T\"-> 0.430000000000  , \"mm1\"-> 0.000000000000  , \"mm2\"-> 0.000000000000  , \"mm3\"-> 0.000000000000  , \"θ\"-> 0.000000000000  |>   , \r55 ->   <| \"ζ\"-> 0.019908376980  , \"τ1\"-> 0.016902177597  , \"τS\"-> 0.037431350421  , \"τN\"-> 0.003115611581  , \"τC\"-> 0.002813000351  , \"κ0\"-> 0.000000003723  , \"T\"-> 0.512000000000  , \"mm1\"-> 0.000000000000  , \"mm2\"-> 0.000000000000  , \"mm3\"-> 0.000000000000  , \"θ\"-> 0.000000000000  |>   , \r56 ->   <| \"ζ\"-> 0.018376000000  , \"τ1\"-> 0.014989979497  , \"τS\"-> 0.031364970092  , \"τN\"-> 0.001876083588  , \"τC\"-> 0.004034409107  , \"κ0\"-> 0.000000004410  , \"T\"-> 0.610000000000  , \"mm1\"-> 0.000000000000  , \"mm2\"-> 0.000000000000  , \"mm3\"-> 0.000000000000  , \"θ\"-> 0.000000000000  |>   , \r57 ->   <| \"ζ\"-> 0.015651665128  , \"τ1\"-> 0.013298894889  , \"τS\"-> 0.022882494925  , \"τN\"-> 0.000826522678  , \"τC\"-> 0.005306542804  , \"κ0\"-> 0.000000006075  , \"T\"-> 0.810000000000  , \"mm1\"-> 0.000000000000  , \"mm2\"-> 0.000000000000  , \"mm3\"-> 0.000000000000  , \"θ\"-> 0.000000000000  |>   , \r58 ->   <| \"ζ\"-> 0.011916480594  , \"τ1\"-> 0.012551282481  , \"τS\"-> 0.018233218660  , \"τN\"-> 0.000345702746  , \"τC\"-> 0.004699451527  , \"κ0\"-> 0.000000008451  , \"T\"-> 1.120000000000  , \"mm1\"-> 0.000000000000  , \"mm2\"-> 0.000000000000  , \"mm3\"-> 0.000000000000  , \"θ\"-> 0.000000000000  |>   , \r59 ->   <| \"ζ\"-> 0.012831327568  , \"τ1\"-> 0.013315909415  , \"τS\"-> 0.012590836847  , \"τN\"-> 0.000065003013  , \"τC\"-> 0.005276356243  , \"κ0\"-> 0.000000013610  , \"T\"-> 1.800000000000  , \"mm1\"-> 0.000000000000  , \"mm2\"-> 0.000000000000  , \"mm3\"-> 0.000000000000  , \"θ\"-> 0.000000000000  |>   , \r60 ->   <| \"ζ\"-> 0.019774146838  , \"τ1\"-> 0.013257273421  , \"τS\"-> 0.007064131508  , \"τN\"-> 0.000028000819  , \"τC\"-> 0.006942241845  , \"κ0\"-> 0.000000023477  , \"T\"-> 3.000000000000  , \"mm1\"-> 0.000000000000  , \"mm2\"-> 0.000000000000  , \"mm3\"-> 0.000000000000  , \"θ\"-> 0.000000000000  |>   , \r61 ->   <| \"ζ\"-> 0.029251354442  , \"τ1\"-> 0.014634751206  , \"τS\"-> 0.003873958746  , \"τN\"-> 0.000007000487  , \"τC\"-> 0.006827504775  , \"κ0\"-> 0.000000056438  , \"T\"-> 5.500000000000  , \"mm1\"-> 0.000000000000  , \"mm2\"-> 0.000000000000  , \"mm3\"-> 0.000000000000  , \"θ\"-> 0.000000000000  |>   , \r70 ->   <| \"ζ\"-> 0.160286026344  , \"τ1\"-> 0.073452047785  , \"τS\"-> 0.044872374187  , \"τN\"-> 0.162076895387  , \"τC\"-> 0.001481759328  , \"κ0\"-> 0.000000001039  , \"T\"-> 0.179000000000  , \"mm1\"-> 0.000000000000  , \"mm2\"-> 0.000000000000  , \"mm3\"-> 0.000000000000  , \"θ\"-> 90.000000000000  |>   , \r71 ->   <| \"ζ\"-> 0.317192968490  , \"τ1\"-> 0.095324848000  , \"τS\"-> 0.087097785701  , \"τN\"-> 0.936221653169  , \"τC\"-> 0.001480807262  , \"κ0\"-> 0.000000000534  , \"T\"-> 0.120000000000  , \"mm1\"-> 0.000000000000  , \"mm2\"-> 0.000000000000  , \"mm3\"-> 0.000000000000  , \"θ\"-> 90.000000000000  |>   , \r72 ->   <| \"ζ\"-> 0.222764630124  , \"τ1\"-> 0.096058032825  , \"τS\"-> 0.066495942806  , \"τN\"-> 0.366151877245  , \"τC\"-> 0.001319275999  , \"κ0\"-> 0.000000000769  , \"T\"-> 0.148000000000  , \"mm1\"-> 0.000000000000  , \"mm2\"-> 0.000000000000  , \"mm3\"-> 0.000000000000  , \"θ\"-> 90.000000000000  |>   , \r73 ->   <| \"ζ\"-> 0.136082903087  , \"τ1\"-> 0.070214285183  , \"τS\"-> 0.041562366618  , \"τN\"-> 0.122478563978  , \"τC\"-> 0.001561716081  , \"κ0\"-> 0.000000001214  , \"T\"-> 0.197000000000  , \"mm1\"-> 0.000000000000  , \"mm2\"-> 0.000000000000  , \"mm3\"-> 0.000000000000  , \"θ\"-> 90.000000000000  |>   , \r74 ->   <| \"ζ\"-> 0.079924133870  , \"τ1\"-> 0.053892600038  , \"τS\"-> 0.033721986821  , \"τN\"-> 0.048194390820  , \"τC\"-> 0.001786420268  , \"κ0\"-> 0.000000001543  , \"T\"-> 0.249000000000  , \"mm1\"-> 0.000000000000  , \"mm2\"-> 0.000000000000  , \"mm3\"-> 0.000000000000  , \"θ\"-> 90.000000000000  |>   , \r75 ->   <| \"ζ\"-> 0.055680730504  , \"τ1\"-> 0.044845519236  , \"τS\"-> 0.029550773155  , \"τN\"-> 0.023428217313  , \"τC\"-> 0.002197475136  , \"κ0\"-> 0.000000001960  , \"T\"-> 0.300000000000  , \"mm1\"-> 0.000000000000  , \"mm2\"-> 0.000000000000  , \"mm3\"-> 0.000000000000  , \"θ\"-> 90.000000000000  |>   , \r76 ->   <| \"ζ\"-> 0.040648812263  , \"τ1\"-> 0.038083560479  , \"τS\"-> 0.026574795079  , \"τN\"-> 0.013361826633  , \"τC\"-> 0.002899405432  , \"κ0\"-> 0.000000002383  , \"T\"-> 0.360000000000  , \"mm1\"-> 0.000000000000  , \"mm2\"-> 0.000000000000  , \"mm3\"-> 0.000000000000  , \"θ\"-> 90.000000000000  |>   , \r77 ->   <| \"ζ\"-> 0.031873906103  , \"τ1\"-> 0.030223838950  , \"τS\"-> 0.024286132427  , \"τN\"-> 0.006926780152  , \"τC\"-> 0.002978043437  , \"κ0\"-> 0.000000002967  , \"T\"-> 0.430000000000  , \"mm1\"-> 0.000000000000  , \"mm2\"-> 0.000000000000  , \"mm3\"-> 0.000000000000  , \"θ\"-> 90.000000000000  |>   , \r78 ->   <| \"ζ\"-> 0.025948172116  , \"τ1\"-> 0.025051552712  , \"τS\"-> 0.022571188655  , \"τN\"-> 0.003812228812  , \"τC\"-> 0.003259730052  , \"κ0\"-> 0.000000003686  , \"T\"-> 0.512000000000  , \"mm1\"-> 0.000000000000  , \"mm2\"-> 0.000000000000  , \"mm3\"-> 0.000000000000  , \"θ\"-> 90.000000000000  |>   , \r79 ->   <| \"ζ\"-> 0.020946044060  , \"τ1\"-> 0.024756174566  , \"τS\"-> 0.021099556284  , \"τN\"-> 0.002276701384  , \"τC\"-> 0.004159440288  , \"κ0\"-> 0.000000004389  , \"T\"-> 0.610000000000  , \"mm1\"-> 0.000000000000  , \"mm2\"-> 0.000000000000  , \"mm3\"-> 0.000000000000  , \"θ\"-> 90.000000000000  |>   , \r80 ->   <| \"ζ\"-> 0.014774082145  , \"τ1\"-> 0.015773102766  , \"τS\"-> 0.018723894921  , \"τN\"-> 0.000790199963  , \"τC\"-> 0.005097561693  , \"κ0\"-> 0.000000006095  , \"T\"-> 0.810000000000  , \"mm1\"-> 0.000000000000  , \"mm2\"-> 0.000000000000  , \"mm3\"-> 0.000000000000  , \"θ\"-> 90.000000000000  |>   , \r81 ->   <| \"ζ\"-> 0.013971175207  , \"τ1\"-> 0.015831825440  , \"τS\"-> 0.017293056061  , \"τN\"-> 0.000406001835  , \"τC\"-> 0.005061653181  , \"κ0\"-> 0.000000008423  , \"T\"-> 1.100000000000  , \"mm1\"-> 0.000000000000  , \"mm2\"-> 0.000000000000  , \"mm3\"-> 0.000000000000  , \"θ\"-> 90.000000000000  |>   , \r82 ->   <| \"ζ\"-> 0.014703834330  , \"τ1\"-> 0.019025451961  , \"τS\"-> 0.011790469569  , \"τN\"-> 0.000107003492  , \"τC\"-> 0.007625608278  , \"κ0\"-> 0.000000014259  , \"T\"-> 1.800000000000  , \"mm1\"-> 0.000000000000  , \"mm2\"-> 0.000000000000  , \"mm3\"-> 0.000000000000  , \"θ\"-> 90.000000000000  |>   , \r83 ->   <| \"ζ\"-> 0.021950059397  , \"τ1\"-> 0.019029879523  , \"τS\"-> 0.006582834729  , \"τN\"-> 0.000028012011  , \"τC\"-> 0.009051896214  , \"κ0\"-> 0.000000024750  , \"T\"-> 3.000000000000  , \"mm1\"-> 0.000000000000  , \"mm2\"-> 0.000000000000  , \"mm3\"-> 0.000000000000  , \"θ\"-> 90.000000000000  |>   , \r84 ->   <| \"ζ\"-> 0.027897403691  , \"τ1\"-> 0.014639690770  , \"τS\"-> 0.004105291179  , \"τN\"-> 0.000006999171  , \"τC\"-> 0.007414449545  , \"κ0\"-> 0.000000059701  , \"T\"-> 5.700000000000  , \"mm1\"-> 0.000073450671  , \"mm2\"-> 0.014673310812  , \"mm3\"-> 0.011534391407  , \"θ\"-> 90.000000000000  |>   , \r"
  in  "input":enum32{"Page 1", "Page 2"}(tab)
  in  "String":string=" <| \"ζ\"->  0.033416389090  , \"τ1\"-> 0.010165657588  , \"τS\"-> 0.048946310195  , \"τN\"-> 0.014465537704  , \"τC\"-> 0.002635749648  , \"κ0\"-> 0.000000002431  , \"mm1\"-> 0.000081122356  , \"mm2\"-> 0.007652084156  , \"mm3\"-> 0.070599043606  , \"T\"->  0.360000000000  , \"B\"-> 12.000000000000  , \"θ\"-> 0.000000000000  |> "
  in  "parse! :p":bool
  in  "Read from file":path=path "/opt/new/Dropbox/shared_AkashAndreas/paper-CeCoIn5/labviewreadydata/CeCoIn5_2nd_053_12T_0.360K_0deg_freqDep_labview_.dat"
  in  "load! :l":bool
  in  "string notes":string="\"T\"-> 0.225000,    \"ζ\"-> 0.006057  , \"τ1\"-> 0.011106  , \"τS\"-> 0.134857  , \"τN\"-> 0.000042  , \"τC\"-> 0.012982  , \"κ0\"-> 0.000000101776  , \"mm1\"-> 0.000071  , \"mm2\"-> 0.148631  , \"mm3\"-> 0.011103 "
  in  "backup string :b":string="\"T\"-> 0.225000,    \"ζ\"-> 0.006057  , \"τ1\"-> 0.011106  , \"τS\"-> 0.134857  , \"τN\"-> 0.000042  , \"τC\"-> 0.012982  , \"κ0\"-> 0.000000101776  , \"mm1\"-> 0.000071  , \"mm2\"-> 0.148631  , \"mm3\"-> 0.011103 "
  in  "plots":enum32{"Page 1", "Page 2"}(tab)
  out "Plot:  colors":cluster{"Freq out (Hz)":dbl[], dbl[]}[](graph)=[{"Freq out (Hz)"=[0.148, 0.179, 0.197, 0.25, 0.3, 0.36, 0.43, 0.512, 0.61, 0.81, 1.12, 1.8, 3.0, 5.5], [0.218787747977, 0.17097389920422382, 0.14761812098892468, 0.11274074360033087, 0.04559581897801322, 0.039475039748, 0.031945976845, 0.023031239946, 0.019920170845, 0.017558473054, 0.011916480594, 0.012831327568, 0.019774146838, 0.029251354442]}, {"Freq out (Hz)"=[0.148, 0.179, 0.197, 0.25, 0.3, 0.36, 0.43, 0.512, 0.61, 0.81, 1.12, 1.8, 3.0, 5.5], [0.031456659327, 0.020780406407531756, 0.017439087629000503, 0.013992698862444412, 0.011644710932388511, 0.021602230815, 0.019000922826, 0.018268814012, 0.016368892412, 0.014545104284, 0.012551282481, 0.013315909415, 0.013257273421, 0.014634751206]}, {"Freq out (Hz)"=[0.148, 0.179, 0.197, 0.25, 0.3, 0.36, 0.43, 0.512, 0.61, 0.81, 1.12, 1.8, 3.0, 5.5], [0.269139973017, 0.07892374572886786, 0.07345575091244771, 0.06366178328551222, 0.05923744701839523, 0.055852925082, 0.045624146388, 0.037269400776, 0.03057953658, 0.022979681288, 0.01823321866, 0.012590836847, 0.007064131508, 0.003873958746]}, {"Freq out (Hz)"=[0.148, 0.179, 0.197, 0.25, 0.3, 0.36, 0.43, 0.512, 0.61, 0.81, 1.12, 1.8, 3.0, 5.5], [0.256714789857, 0.21798091781830217, 0.13956179065392582, 0.05207630273431135, 0.024840698735647763, 0.00816381305, 0.005314716063, 0.00269679289, 0.001736017565, 0.000840829385, 0.000345702746, 6.5003013e-05, 2.8000819e-05, 7.000487e-06]}, {"Freq out (Hz)"=[0.148, 0.179, 0.197, 0.25, 0.3, 0.36, 0.43, 0.512, 0.61, 0.81, 1.12, 1.8, 3.0, 5.5], [0.001257909269, 0.0010028907738879789, 0.0009010361830654456, 0.0005326114848183616, 0.0024545078524793656, 0.002520091738, 0.002488383471, 0.003257395394, 0.004971418152, 0.00522803024, 0.004699451527, 0.005276356243, 0.006942241845, 0.006827504775]}]
  in  "parameter selectors":enum32{"Page 1"}(tab)
  in  "select B (T)":u16(ring) items=["12.000000"]
  in  "select θ (deg)":u16(ring) items=["0.000000", "90.000000"]
  in  "ignore T !":bool=TRUE
  in  "select T (T)":u16(ring) items=["0.120000", "0.148000", "0.179000", "0.197000", "0.249000", "0.250000", "0.300000", "0.360000", "0.430000", "0.512000", "0.610000", "0.810000", "1.100000", "1.120000", "1.800000", "3.000000", "5.500000", "5.700000"]
  in  "ignore B !":bool
  in  "ignore θ !":bool
  in  "X selector":T1=enum."T (K)"
  in  "parameters":enum32{"Page 1"}(tab)
  in  "ζ":dbl(slide)=0.03341638908995967 min=0.0 max=0.3 step=1e-06 scale=1e-05..1000.0 scale format="%#_3p"
  in  "T1":dbl(slide)=0.010165657588352316 min=0.0 max=0.3 step=1e-06 scale=0.0001..1000.0 scale format="%#_3p"
  in  "τS":dbl(slide)=0.04894631019507874 min=0.0 max=0.3 step=1e-06 scale=0.0001..10.0 scale format="%#_3p"
  in  "τN":dbl(slide)=0.014465537704024084 min=0.0 max=0.3 step=1e-06 scale=1e-06..1000.0 scale format="%#_3p"
  in  "τC":dbl(slide)=0.002635749648085244 min=0.0 max=0.3 step=1e-06 scale=0.0001..10.0 scale format="%#_3p"
  in  "κ0":dbl(slide)=2.4306364470344755e-09 min=0.0 max=0.3 step=1e-12 scale=1e-10..1e-06 scale format="%#_3p"
  in  "newton control":enum32{"Page 1", "Page 2"}(tab)
  in  "pause!":bool
  in  "newton control":enum32{"Page 1"}(tab)
  in  "# steps":dbl=250.0 format="%#_10f"
  in  "gradient factor":dbl(slide)=7.40925439579986e-05 scale=1e-06..1.0 scale format="%#_3p"
  out "logarithmic derivatives":dbl[](array[numeric])=[-0.4786399825424796, 0.5445905389195271, -0.5599486619851562, 2.3056625030751086, 0.04611264466244743, -0.03487920539952545]
  in  "weighting":T3=enum."|dz/dω|"
  out "goodness":dbl=8.801800703278548e-05 format="%#_10f"
  in  "go!":bool
  in  "what":cluster{"scaling":dbl, "what":T1}[](array[cluster])=[{"scaling"=1.0, "what"=enum."ζ"}, {"scaling"=1.0, "what"=enum."τ1"}, {"scaling"=1.0, "what"=enum."τS"}, {"scaling"=1.0, "what"=enum."τN"}, {"scaling"=10.0, "what"=enum."τC"}, {"scaling"=1.0, "what"=enum."κ0"}]
  out "θ (deg)":dbl format="%#_10f"
  out "T (K)":dbl=0.36 format="%#_10f"
  out "file index":i32=53
  out "B (T)":dbl=12.0
  in  "newton pause":bool=TRUE
  in  "sweeper panel":T4(tab)
  out "Plot: sweep window":cluster{"Freq out (Hz)":dbl[], dbl[]}[](graph)
  in  "scale gauge: Plot: complex plane":dbl(slide)=617512679.872548 min=0.0 max=0.3 step=1e-06 scale=1e-05..100000000000.0 scale format="%#_3p"
  in  "ω0 (rad/sec)":dbl(slide)=140.85980015121274 scale=0.001..50000.0 scale format="%#_3f"
  in  "offset control tab":enum32{"Page 1"}(tab)
  in  "off\nRe\nIm":cluster{"Numeric":dbl, "Numeric":dbl}(slide)={"Numeric"=-1851851.8518518507, "Numeric"=0.0} scale=-50000000.0..100000000.0 scale format="%#_1p"
  in  "cspan":dbl=0.003 format="%#_13g"
  in  "cursor window":T5={"left"=20184.313682072192, "right "=24669.14654231211, "center"=22426.730112192152, "window"=4484.832860239923, "cursors"=[0, 1, 2], "relative"=0, "absolute"=0, "fixed vertical offset"=0.0, "vertical offset"=0.0, "skew"=0.0, "default window frac"=0.1, "kind"=enum."symmetric", "skew.left"=0.5, "skew.right"=0.5, "Plot ref"=refnum, "wing order"=enum."forw"}
  in  "win":T6={"cen (Hz)"=23772.179970264126, "win (Hz)"=4484.832860239923, "left (Hz)"=21529.763540144166, "right (Hz)"=26014.596400384085}
  in  ":sweep is ON":bool
  in  "stopping criteria":T7={"function tolerance"=1e-06, "parameter tolerance"=1e-06, "max iterations"=100, "max function calls"=1000, "gradient tolerance"=1e-06, "max time (sec)"=-1.0}
  in  "uco! :u":bool
  in  "tr":enum16{"as is", "add - ω", "full rydh"}(ring)=enum."add - ω"
  out "cursor x selector":map{T1, dbl}(c390)={enum."T (K)"=0.36, enum."B (T)"=12.0, enum."θ (deg)"=0.0}
  out "Plot: phase":cluster{"Freq out (Hz)":dbl[], dbl[]}[](graph)
  in  "save data":enum32{"save/read"}(tab)
  in  "Save to file :s":bool
  in  "Freq sweep name template":T8={"prefix"="RuCl3-rod", "group"="f"}
  in  "Save folder":path=path "/opt/data"
  in  "freq sweep file name":string="f004_RuCl3-rod_060221.dat"
  in  "cursor index map":map{T1, i32}(c390)={enum."ζ"=0, enum."τ1"=1, enum."τS"=2, enum."τN"=3, enum."τC"=4, enum."κ0"=5, enum."m1"=6, enum."m2"=7, enum."m3"=8}
  out "temps&degs":map{i32, map{T1, dbl}}(c390)={48={enum."T (K)"=0.148, enum."B (T)"=12.0, enum."θ (deg)"=0.0}, 49={enum."T (K)"=0.179, enum."B (T)"=12.0, enum."θ (deg)"=0.0}, 50={enum."T (K)"=0.197, enum."B (T)"=12.0, enum."θ (deg)"=0.0}, 51={enum."T (K)"=0.25, enum."B (T)"=12.0, enum."θ (deg)"=0.0}, 52={enum."T (K)"=0.3, enum."B (T)"=12.0, enum."θ (deg)"=0.0}, 53={enum."T (K)"=0.36, enum."B (T)"=12.0, enum."θ (deg)"=0.0}, 54={enum."T (K)"=0.43, enum."B (T)"=12.0, enum."θ (deg)"=0.0}, 55={enum."T (K)"=0.512, enum."B (T)"=12.0, enum."θ (deg)"=0.0}, 56={enum."T (K)"=0.61, enum."B (T)"=12.0, enum."θ (deg)"=0.0}, 57={enum."T (K)"=0.81, enum."B (T)"=12.0, enum."θ (deg)"=0.0}, 58={enum."T (K)"=1.12, enum."B (T)"=12.0, enum."θ (deg)"=0.0}, 59={enum."T (K)"=1.8, enum."B (T)"=12.0, enum."θ (deg)"=0.0}, 60={enum."T (K)"=3.0, enum."B (T)"=12.0, enum."θ (deg)"=0.0}, 61={enum."T (K)"=5.5, enum."B (T)"=12.0, enum."θ (deg)"=0.0}, 70={enum."T (K)"=0.179, enum."B (T)"=12.0, enum."θ (deg)"=90.0}, 71={enum."T (K)"=0.12, enum."B (T)"=12.0, enum."θ (deg)"=90.0}, 72={enum."T (K)"=0.148, enum."B (T)"=12.0, enum."θ (deg)"=90.0}, 73={enum."T (K)"=0.197, enum."B (T)"=12.0, enum."θ (deg)"=90.0}, 74={enum."T (K)"=0.249, enum."B (T)"=12.0, enum."θ (deg)"=90.0}, 75={enum."T (K)"=0.3, enum."B (T)"=12.0, enum."θ (deg)"=90.0}, 76={enum."T (K)"=0.36, enum."B (T)"=12.0, enum."θ (deg)"=90.0}, 77={enum."T (K)"=0.43, enum."B (T)"=12.0, enum."θ (deg)"=90.0}, 78={enum."T (K)"=0.512, enum."B (T)"=12.0, enum."θ (deg)"=90.0}, 79={enum."T (K)"=0.61, enum."B (T)"=12.0, enum."θ (deg)"=90.0}, 80={enum."T (K)"=0.81, enum."B (T)"=12.0, enum."θ (deg)"=90.0}, 81={enum."T (K)"=1.1, enum."B (T)"=12.0, enum."θ (deg)"=90.0}, 82={enum."T (K)"=1.8, enum."B (T)"=12.0, enum."θ (deg)"=90.0}, 83={enum."T (K)"=3.0, enum."B (T)"=12.0, enum."θ (deg)"=90.0}, 84={enum."T (K)"=5.7, enum."B (T)"=12.0, enum."θ (deg)"=90.0}}
  out "mathematica thing":map{i32, map{T1, dbl}}(c390)={48={enum."ζ"=0.218787747977, enum."τ1"=0.031456659327, enum."τS"=0.269139973017, enum."τN"=0.256714789857, enum."τC"=0.001257909269, enum."κ0"=7.59e-10, enum."m1"=0.0, enum."m2"=0.0, enum."m3"=0.0, enum."T (K)"=0.148, enum."B (T)"=12.0, enum."θ (deg)"=0.0}, 49={enum."ζ"=0.17097389920422382, enum."τ1"=0.020780406407531756, enum."τS"=0.07892374572886786, enum."τN"=0.21798091781830217, enum."τC"=0.0010028907738879789, enum."κ0"=1.037573495113704e-09, enum."m1"=0.00014505896771698846, enum."m2"=0.005326274955191035, enum."m3"=0.3639795748242596, enum."T (K)"=0.179, enum."B (T)"=12.0, enum."θ (deg)"=0.0}, 50={enum."ζ"=0.14761812098892468, enum."τ1"=0.017439087629000503, enum."τS"=0.07345575091244771, enum."τN"=0.13956179065392582, enum."τC"=0.0009010361830654456, enum."κ0"=1.1823236559074934e-09, enum."m1"=0.00011481579473876581, enum."m2"=0.0057762461188156184, enum."m3"=0.25691185268859335, enum."T (K)"=0.197, enum."B (T)"=12.0, enum."θ (deg)"=0.0}, 51={enum."ζ"=0.11274074360033087, enum."τ1"=0.013992698862444412, enum."τS"=0.06366178328551222, enum."τN"=0.05207630273431135, enum."τC"=0.0005326114848183616, enum."κ0"=1.4852787827729598e-09, enum."m1"=5.359958459029188e-05, enum."m2"=0.0073424414045021435, enum."m3"=0.13591575325874794, enum."T (K)"=0.25, enum."B (T)"=12.0, enum."θ (deg)"=0.0}, 52={enum."ζ"=0.04559581897801322, enum."τ1"=0.011644710932388511, enum."τS"=0.05923744701839523, enum."τN"=0.024840698735647763, enum."τC"=0.0024545078524793656, enum."κ0"=1.978437402181448e-09, enum."m1"=0.0001031059636937415, enum."m2"=0.007970635185906098, enum."m3"=0.09393723530311938, enum."T (K)"=0.3, enum."B (T)"=12.0, enum."θ (deg)"=0.0}, 53={enum."ζ"=0.039475039748, enum."τ1"=0.021602230815, enum."τS"=0.055852925082, enum."τN"=0.00816381305, enum."τC"=0.002520091738, enum."κ0"=2.417e-09, enum."m1"=0.0, enum."m2"=0.0, enum."m3"=0.0, enum."T (K)"=0.36, enum."B (T)"=12.0, enum."θ (deg)"=0.0}, 54={enum."ζ"=0.031945976845, enum."τ1"=0.019000922826, enum."τS"=0.045624146388, enum."τN"=0.005314716063, enum."τC"=0.002488383471, enum."κ0"=2.954e-09, enum."m1"=0.0, enum."m2"=0.0, enum."m3"=0.0, enum."T (K)"=0.43, enum."B (T)"=12.0, enum."θ (deg)"=0.0}, 55={enum."ζ"=0.023031239946, enum."τ1"=0.018268814012, enum."τS"=0.037269400776, enum."τN"=0.00269679289, enum."τC"=0.003257395394, enum."κ0"=3.72e-09, enum."m1"=0.0, enum."m2"=0.0, enum."m3"=0.0, enum."T (K)"=0.512, enum."B (T)"=12.0, enum."θ (deg)"=0.0}, 56={enum."ζ"=0.019920170845, enum."τ1"=0.016368892412, enum."τS"=0.03057953658, enum."τN"=0.001736017565, enum."τC"=0.004971418152, enum."κ0"=4.41e-09, enum."m1"=0.0, enum."m2"=0.0, enum."m3"=0.0, enum."T (K)"=0.61, enum."B (T)"=12.0, enum."θ (deg)"=0.0}, 57={enum."ζ"=0.017558473054, enum."τ1"=0.014545104284, enum."τS"=0.022979681288, enum."τN"=0.000840829385, enum."τC"=0.00522803024, enum."κ0"=6.068e-09, enum."m1"=0.0, enum."m2"=0.0, enum."m3"=0.0, enum."T (K)"=0.81, enum."B (T)"=12.0, enum."θ (deg)"=0.0}, 58={enum."ζ"=0.011916480594, enum."τ1"=0.012551282481, enum."τS"=0.01823321866, enum."τN"=0.000345702746, enum."τC"=0.004699451527, enum."κ0"=8.451e-09, enum."m1"=0.0, enum."m2"=0.0, enum."m3"=0.0, enum."T (K)"=1.12, enum."B (T)"=12.0, enum."θ (deg)"=0.0}, 59={enum."ζ"=0.012831327568, enum."τ1"=0.013315909415, enum."τS"=0.012590836847, enum."τN"=6.5003013e-05, enum."τC"=0.005276356243, enum."κ0"=1.361e-08, enum."m1"=0.0, enum."m2"=0.0, enum."m3"=0.0, enum."T (K)"=1.8, enum."B (T)"=12.0, enum."θ (deg)"=0.0}, 60={enum."ζ"=0.019774146838, enum."τ1"=0.013257273421, enum."τS"=0.007064131508, enum."τN"=2.8000819e-05, enum."τC"=0.006942241845, enum."κ0"=2.3477e-08, enum."m1"=0.0, enum."m2"=0.0, enum."m3"=0.0, enum."T (K)"=3.0, enum."B (T)"=12.0, enum."θ (deg)"=0.0}, 61={enum."ζ"=0.029251354442, enum."τ1"=0.014634751206, enum."τS"=0.003873958746, enum."τN"=7.000487e-06, enum."τC"=0.006827504775, enum."κ0"=5.6438e-08, enum."m1"=0.0, enum."m2"=0.0, enum."m3"=0.0, enum."T (K)"=5.5, enum."B (T)"=12.0, enum."θ (deg)"=0.0}, 70={enum."ζ"=0.16687004024769275, enum."τ1"=0.07230206533653885, enum."τS"=0.041247201771786146, enum."τN"=0.16130228501353755, enum."τC"=0.0012104695826081564, enum."κ0"=1.0265454590974847e-09, enum."m1"=0.00016940679594146428, enum."m2"=0.011942507015549044, enum."m3"=0.29774954890499666, enum."T (K)"=0.179, enum."B (T)"=12.0, enum."θ (deg)"=90.0}, 71={enum."ζ"=0.31719296849, enum."τ1"=0.095324848, enum."τS"=0.087097785701, enum."τN"=0.936221653169, enum."τC"=0.001480807262, enum."κ0"=5.34e-10, enum."m1"=0.0, enum."m2"=0.0, enum."m3"=0.0, enum."T (K)"=0.12, enum."B (T)"=12.0, enum."θ (deg)"=90.0}, 72={enum."ζ"=0.21779292555204557, enum."τ1"=0.09577148981745257, enum."τS"=0.07303905538394233, enum."τN"=0.36551960376559023, enum."τC"=0.0014682873216596848, enum."κ0"=7.760669180430888e-10, enum."m1"=0.00025902196149852626, enum."m2"=0.013995321620223699, enum."m3"=0.6170590661092816, enum."T (K)"=0.148, enum."B (T)"=12.0, enum."θ (deg)"=90.0}, 73={enum."ζ"=0.136975374218, enum."τ1"=0.070969356603, enum."τS"=0.041937456488, enum."τN"=0.122985136767, enum."τC"=0.00156828093, enum."κ0"=1.212e-09, enum."m1"=0.0, enum."m2"=0.0, enum."m3"=0.0, enum."T (K)"=0.197, enum."B (T)"=12.0, enum."θ (deg)"=90.0}, 74={enum."ζ"=0.081038743925, enum."τ1"=0.054864856987, enum."τS"=0.033961002119, enum."τN"=0.048653010594, enum."τC"=0.001781381797, enum."κ0"=1.539e-09, enum."m1"=0.0, enum."m2"=0.0, enum."m3"=0.0, enum."T (K)"=0.249, enum."B (T)"=12.0, enum."θ (deg)"=90.0}, 75={enum."ζ"=0.056185573597, enum."τ1"=0.045207611912, enum."τS"=0.02960302601, enum."τN"=0.023507324547, enum."τC"=0.002233080371, enum."κ0"=1.957e-09, enum."m1"=0.0, enum."m2"=0.0, enum."m3"=0.0, enum."T (K)"=0.3, enum."B (T)"=12.0, enum."θ (deg)"=90.0}, 76={enum."ζ"=0.041794370964, enum."τ1"=0.038862739492, enum."τS"=0.026705422753, enum."τN"=0.013514328703, enum."τC"=0.002820386983, enum."κ0"=2.373e-09, enum."m1"=0.0, enum."m2"=0.0, enum."m3"=0.0, enum."T (K)"=0.36, enum."B (T)"=12.0, enum."θ (deg)"=90.0}, 77={enum."ζ"=0.033296236595, enum."τ1"=0.031336126456, enum."τS"=0.024496257026, enum."τN"=0.007027117109, enum."τC"=0.00282530283, enum."κ0"=2.954e-09, enum."m1"=0.0, enum."m2"=0.0, enum."m3"=0.0, enum."T (K)"=0.43, enum."B (T)"=12.0, enum."θ (deg)"=90.0}, 78={enum."ζ"=0.02714440216, enum."τ1"=0.026090960664, enum."τS"=0.02207893779, enum."τN"=0.003827547658, enum."τC"=0.003825438719, enum."κ0"=3.686e-09, enum."m1"=0.0, enum."m2"=0.0, enum."m3"=0.0, enum."T (K)"=0.512, enum."B (T)"=12.0, enum."θ (deg)"=90.0}, 79={enum."ζ"=0.020263859818, enum."τ1"=0.022629231163, enum."τS"=0.021062454034, enum."τN"=0.00223839947, enum."τC"=0.004128602745, enum."κ0"=4.397e-09, enum."m1"=0.0, enum."m2"=0.0, enum."m3"=0.0, enum."T (K)"=0.61, enum."B (T)"=12.0, enum."θ (deg)"=90.0}, 80={enum."ζ"=0.014774082145, enum."τ1"=0.015773102766, enum."τS"=0.018723894921, enum."τN"=0.000790199963, enum."τC"=0.005097561693, enum."κ0"=6.095e-09, enum."m1"=0.0, enum."m2"=0.0, enum."m3"=0.0, enum."T (K)"=0.81, enum."B (T)"=12.0, enum."θ (deg)"=90.0}, 81={enum."ζ"=0.014230278097, enum."τ1"=0.016181489886, enum."τS"=0.016832346578, enum."τN"=0.000327070958, enum."τC"=0.005559720416, enum."κ0"=8.431e-09, enum."m1"=0.0, enum."m2"=0.0, enum."m3"=0.0, enum."T (K)"=1.1, enum."B (T)"=12.0, enum."θ (deg)"=90.0}, 82={enum."ζ"=0.01470383433, enum."τ1"=0.019025451961, enum."τS"=0.011790469569, enum."τN"=0.000107003492, enum."τC"=0.007625608278, enum."κ0"=1.4259e-08, enum."m1"=0.0, enum."m2"=0.0, enum."m3"=0.0, enum."T (K)"=1.8, enum."B (T)"=12.0, enum."θ (deg)"=90.0}, 83={enum."ζ"=0.021950059397, enum."τ1"=0.019029879523, enum."τS"=0.006582834729, enum."τN"=2.8012011e-05, enum."τC"=0.009051896214, enum."κ0"=2.475e-08, enum."m1"=0.0, enum."m2"=0.0, enum."m3"=0.0, enum."T (K)"=3.0, enum."B (T)"=12.0, enum."θ (deg)"=90.0}, 84={enum."ζ"=0.027897403691, enum."τ1"=0.01463969077, enum."τS"=0.004105291179, enum."τN"=6.999171e-06, enum."τC"=0.007414449545, enum."κ0"=5.9701e-08, enum."m1"=0.0, enum."m2"=0.0, enum."m3"=0.0, enum."T (K)"=5.7, enum."B (T)"=12.0, enum."θ (deg)"=90.0}}
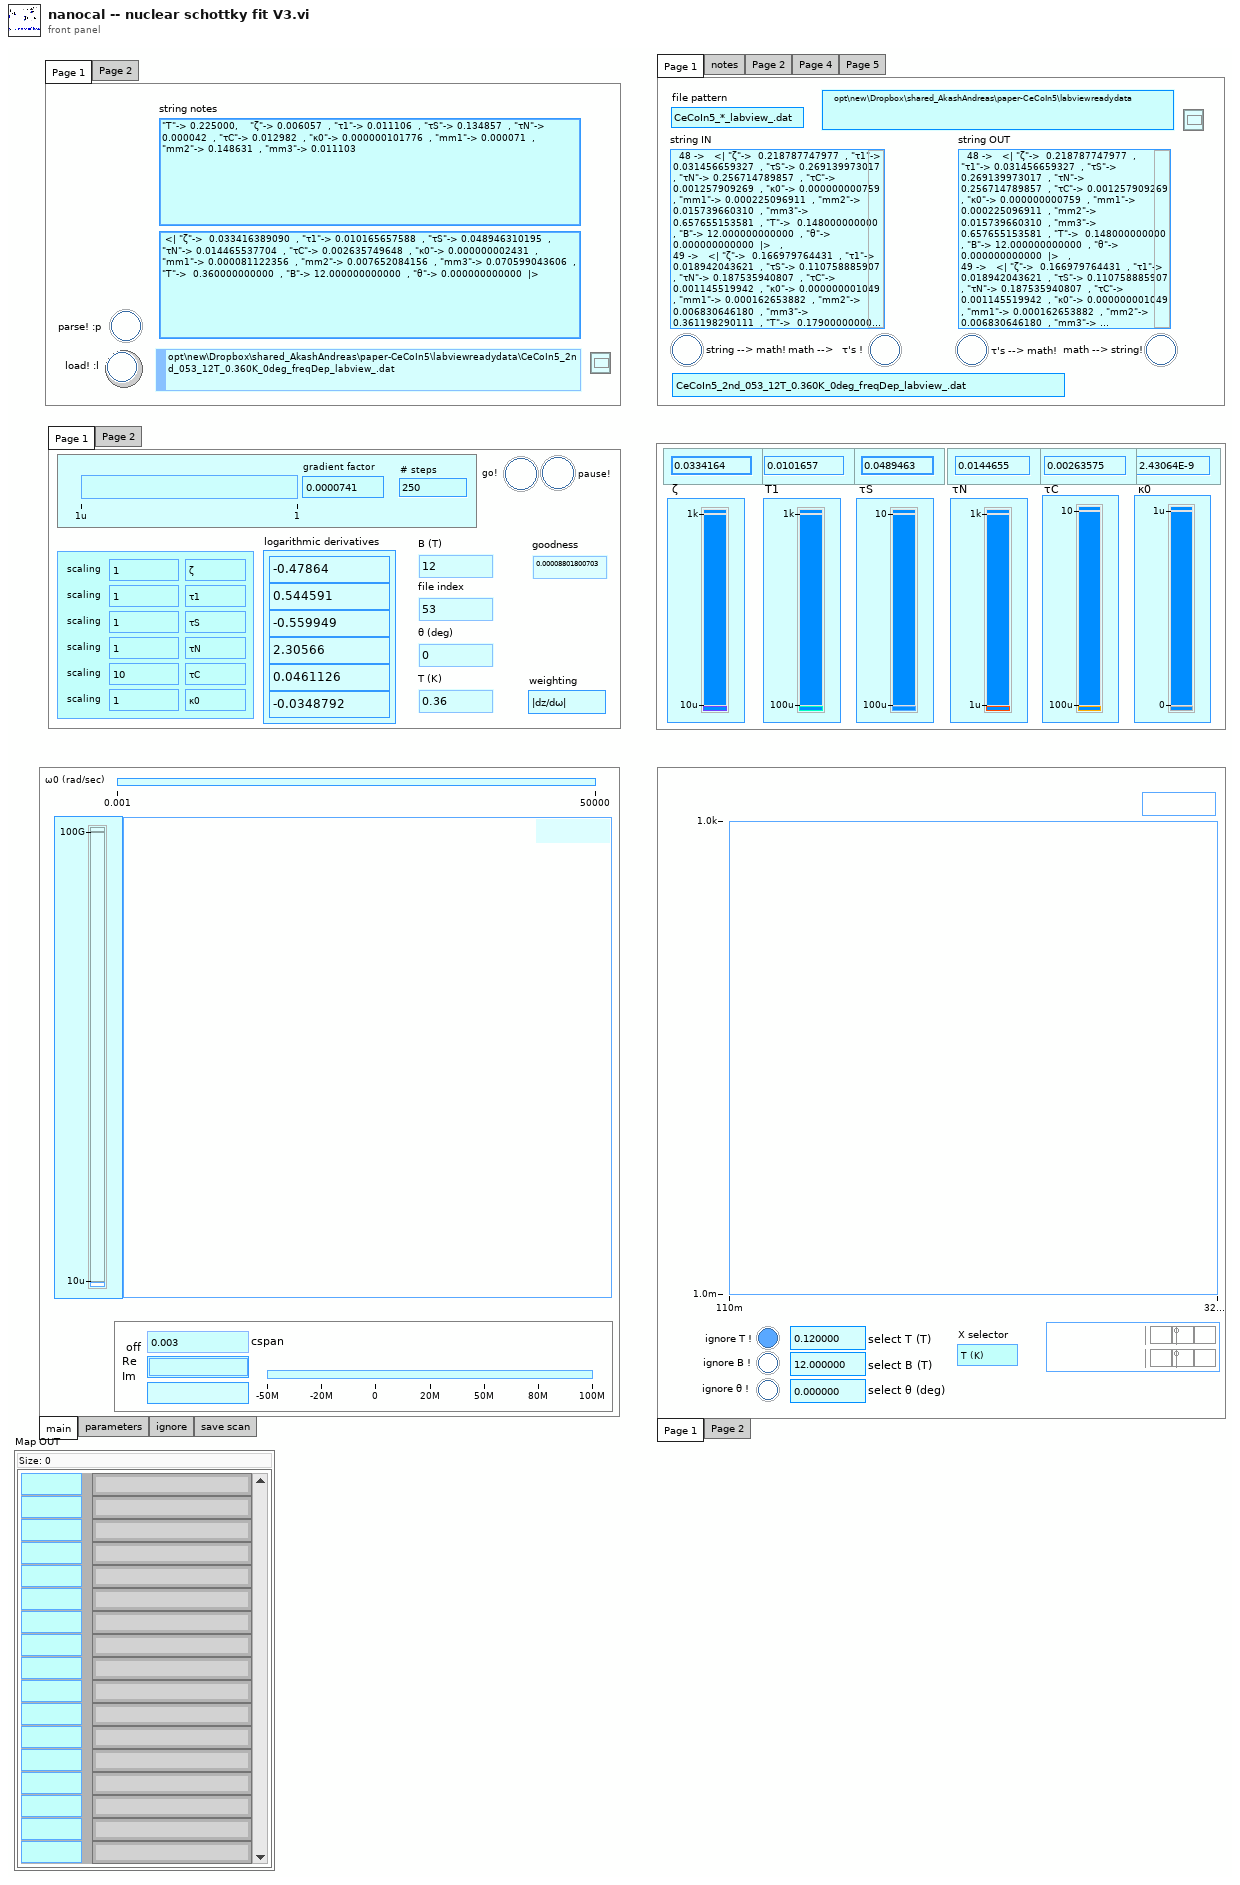
[diagram p1: front panel]
types:
  T1 = typedef "3-lorentzian-parameters.ctl" = enum16{"ζ", "τ1", "τS", "τN", "τC", "κ0", "m1", "m2", "m3", "T (K)", "B (T)", "θ (deg)"}
  T2 = enum32{"Page 1", "notes", "Page 2", "Page 4", "Page 5"}
  T3 = typedef "nanocal-goodness-weighting-strategy.ctl" = enum16{"as is", "|dz/dω|", "ω", "phase"}
  T4 = enum32{"main", "parameters", "ignore", "save scan"}
  T5 = typedef "cursor winow.ctl" = cluster{"left":dbl, "right ":dbl, "center":dbl, "window":dbl, "cursors":i32[], "relative":i32, "absolute":i32, "fixed vertical offset":dbl, "vertical offset":dbl, "skew":dbl, "default window frac":dbl, "kind":enum16{"symmetric", "skewed", "fancy"}, "skew.left":dbl, "skew.right":dbl, "Plot ref":refnum<vi>, "wing order":enum16{"forw", "back"}}
  T6 = typedef "show-win- control.ctl" = cluster{"cen (Hz)":dbl, "win (Hz)":dbl, "left (Hz)":dbl, "right (Hz)":dbl}
  T7 = typedef "NI_Gmath.lvlib/stopping criteria.ctl" = cluster{"function tolerance":dbl, "parameter tolerance":dbl, "max iterations":i32, "max function calls":i32, "gradient tolerance":dbl, "max time (sec)":dbl}
  T8 = typedef "filename-pattern.ctl" = cluster{"prefix":string, "group":string}
  T9 = typedef "3-lorentzian-heat-response action.ctl" = enum16{"calc R", "create string", "calc m1m2m3", "dζ", "dT1", "dτS", "dτN", "dτC", "d-all", "dκ0", "T(K)", "m1", "m2", "m3", "parse string", "θ (deg)", "B (T)"}
  T10 = typedef "cursor action.ctl" = enum16{"range", "read", "write", "check", "zoom out", "smart zoom out", "zoom to aspect ratio 1", "zoom to win", "zoom out 20%", "zoom in 20%", "-empty", "smart zoom out&aspect", "move range left 20%", "move range right 20%", "move range up 20%", "move range down 20%", "zoom to X win", "zoom to Y win", "zoom out X", "zoom out Y", "zoom in X", "zoom in Y", "check plot scale"}
  T11 = typedef "cursor window action.ctl" = enum16{"balance", "h. offset change", "cursor moves", "change center", "change window", "init", "check", "reset", "set y to middle", "idle", "-write all Y", "-write left.X", "-write center.X", "-write right.X", "-write all X", "-change center", "-change window", "-change skew", "-read cursor 2", "-read cursor 1", "-read cursor 0", "-read all cursors", "-reset", "-read plot scale", "-set y to middle", "-Q: center.Y is visible", "-Q: window is visible", "-parse center.Y", "-right left from center", "-left move", "-right move", "-set center.Y", "-empty", "-set cursors to default", "-check", "-write center.Y", "-copy cursor 1", "-copy cursor 0", "-copy cursor 2", "move right", "move left", "shrink", "broaden", "skew up", "skew down", "-write plot scale", "zoom X", "change cen&win", "zoom to all data", "color--red", "color--green", "color--yellow", "read", "zoom out", "zoom in", "slide right", "slide left", "set range aspect ratio to 1"}
  T12 = typedef "mathematica string map action.ctl" = enum16{"create string", "calc m1m2m3", "parse string"}
  T13 = typedef "publisher action.ctl" = enum16{"set", "get", "init", "check"}
  T14 = typedef "3-lorentzian-parameters -- action.ctl" = enum16{"to array", "to parameters"}
  T15 = typedef "NI_Gmath.lvlib/objective function data.ctl" = variant
  T16 = typedef "filename-action.ctl" = enum16{"rewrite", "parse", "force pattern", "uniquenum", "get T", "get B", "get ind", "get deg", "get name", "get folder", "get extension", "get basename"}
  T17 = typedef "LVMapReplaceAction.ctl" = enum32{"Modify Entry only if found", "Add or Modify Entry", "Delete Entry"}
  T18 = typedef "file -- read-write control.ctl" = enum16{"read", "write all", "append one line"}
  T19 = typedef "array -- freq-voltage transformations action.ctl" = enum16{"as is", "add -ω", "sort ω", "2 x ω", "R-phase(deg) to Re-Im", "select ω>0"}
  T20 = typedef "KM_file -- read-write control.ctl" = enum16{"read", "write all", "append one line"}
  T21 = typedef "2Dwindow.ctl" = cluster{"window y":dbl, "center x":dbl, "center y":dbl, "window x":dbl}
  T22 = typedef "eventvkey.ctl" = enum16{"ASCII", "Enter", "Return", "Shift", "Ctrl", "Alt", "Cmd", "Opt", "Caps", "NumLock", "Clear", "Break", "Up", "Down", "Left", "Right", "Insert", "Delete", "Home", "End", "PageUp", "PageDown", "Escape", "Help", "Pause", "ScrollLock", "F1", "F2", "F3", "F4", "F5", "F6", "F7", "F8", "F9", "F10", "F11", "F12", "F13", "F14", "F15", "F16", "F17", "F18", "F19", "F20", "F21", "F22", "F23", "F24", "Play", "VolumeUp", "VolumeDown", "Mute", "Two Byte Char"}
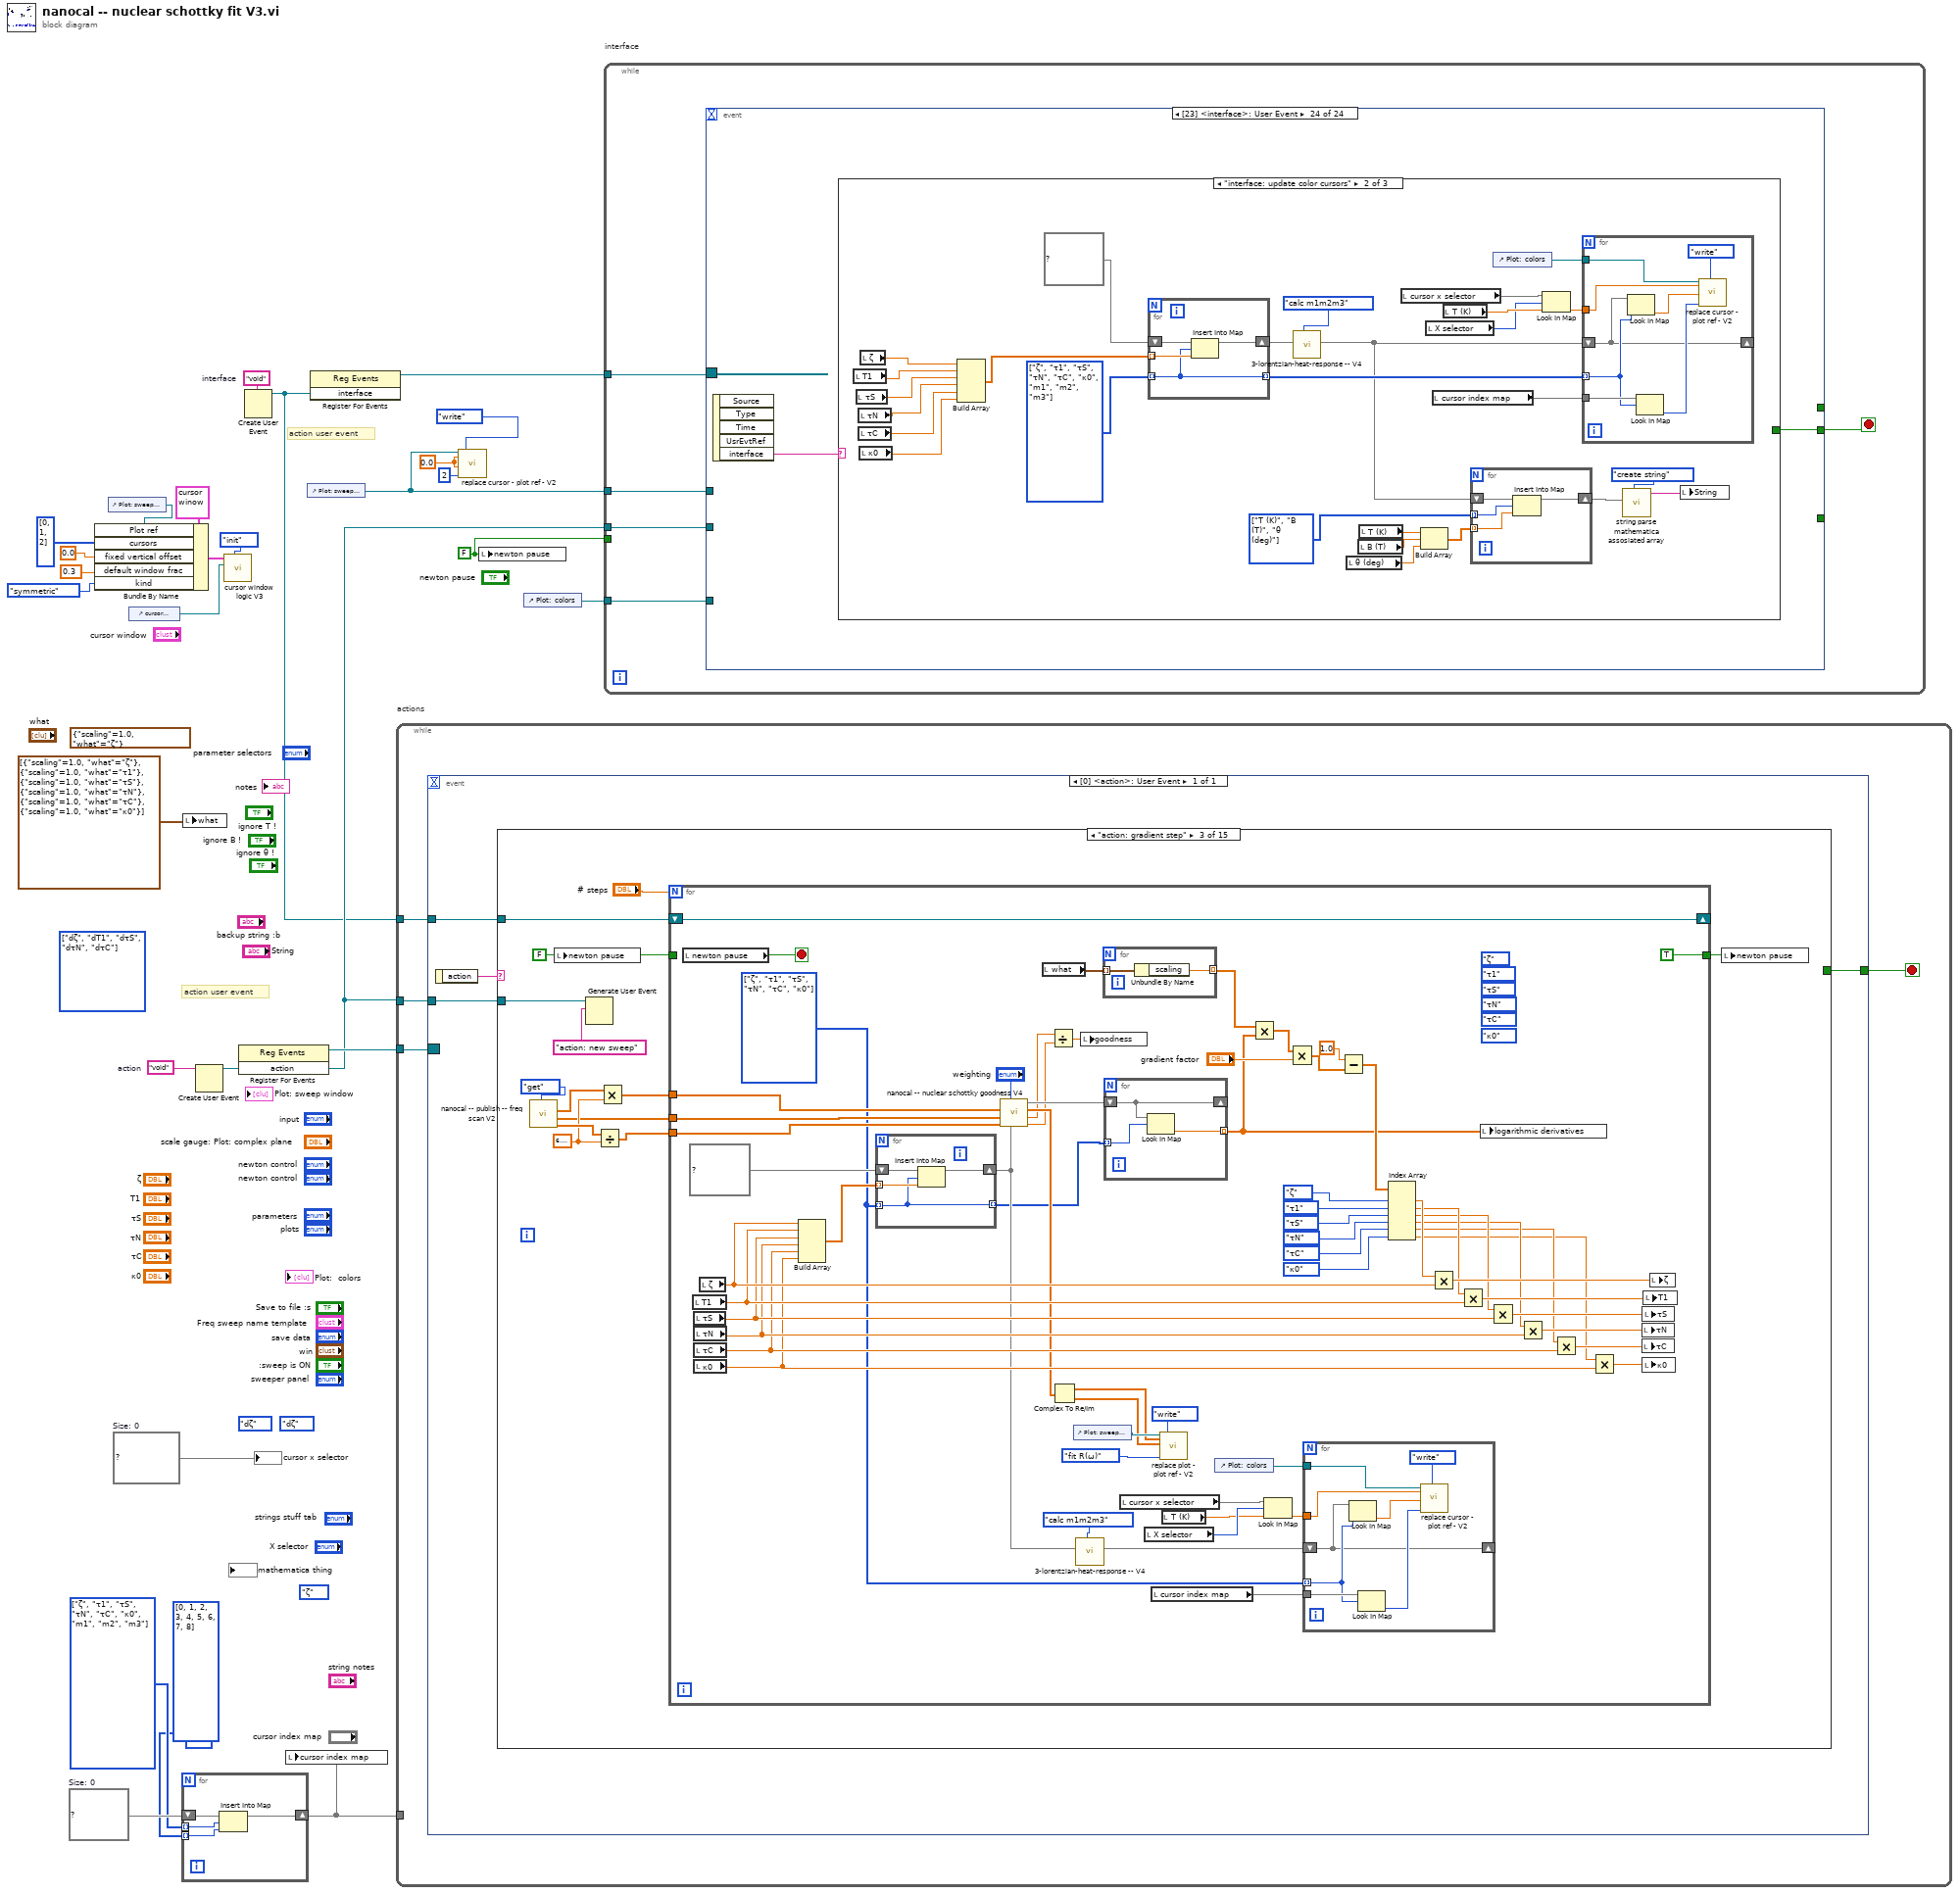
[diagram p0: block diagram]
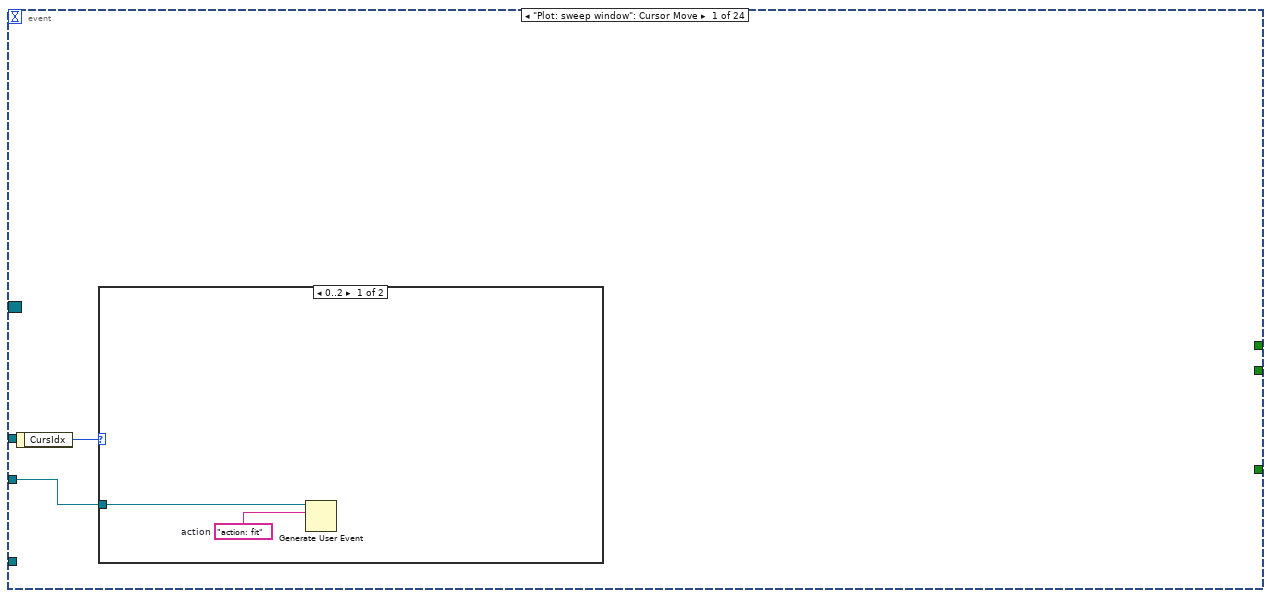
[diagram p2: hidden frame]
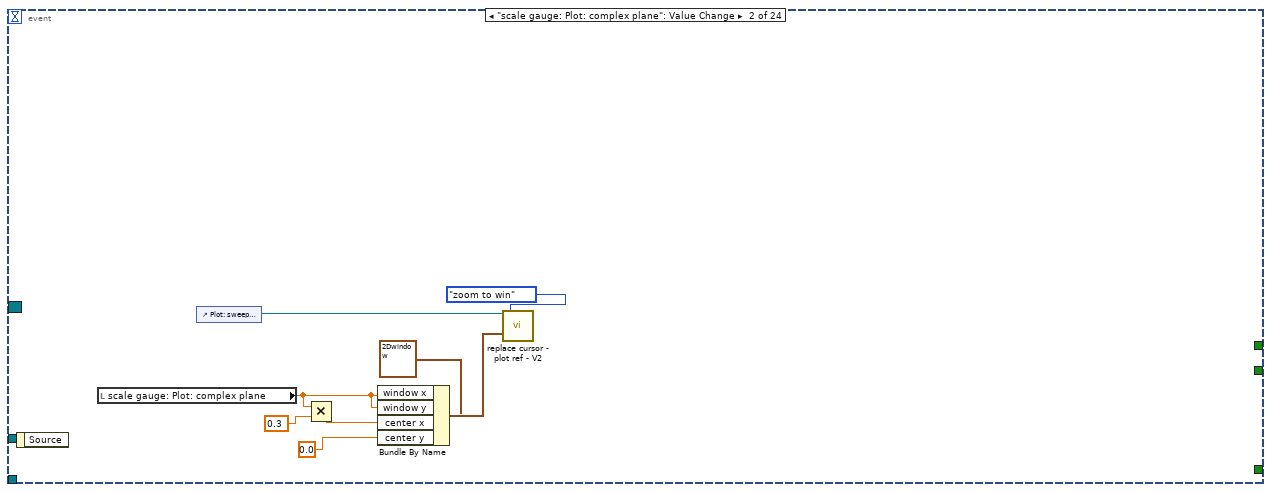
[diagram p4: hidden frame]
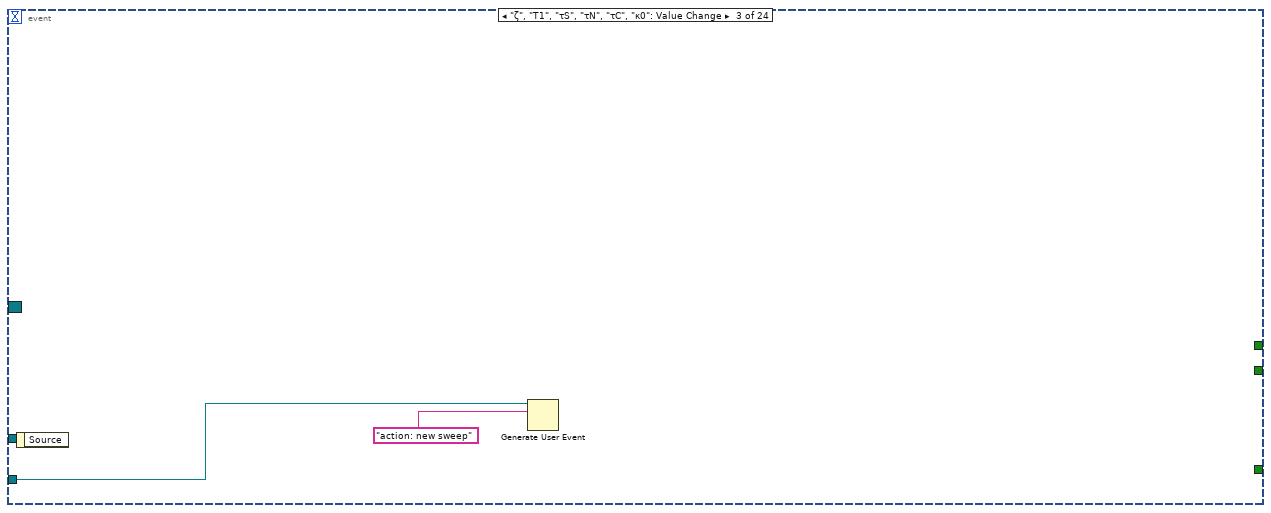
[diagram p5: hidden frame]
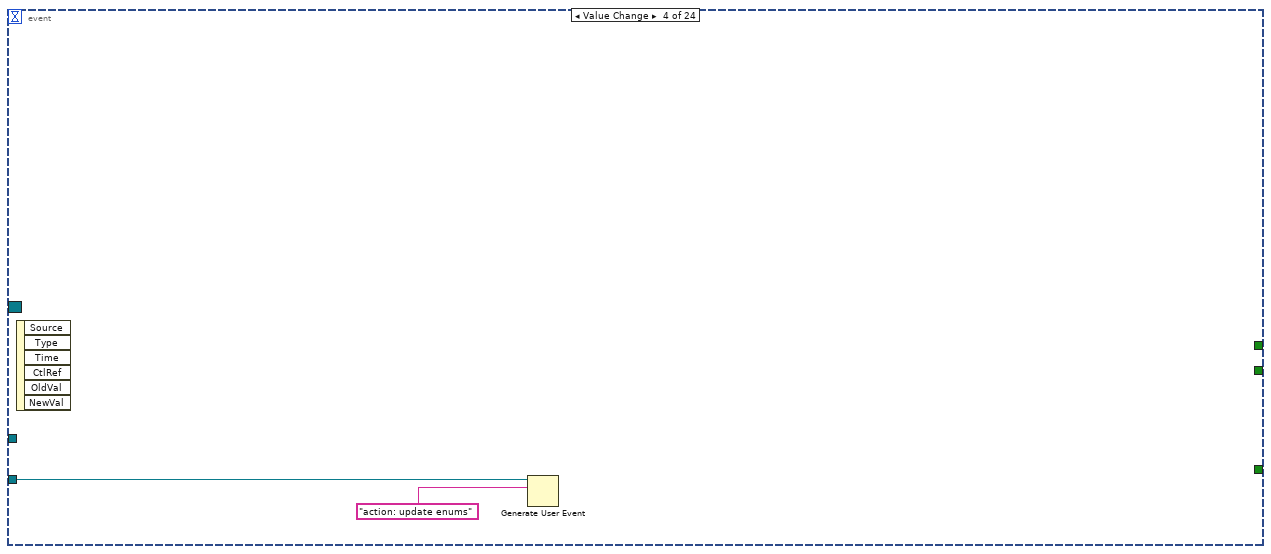
[diagram p6: hidden frame]
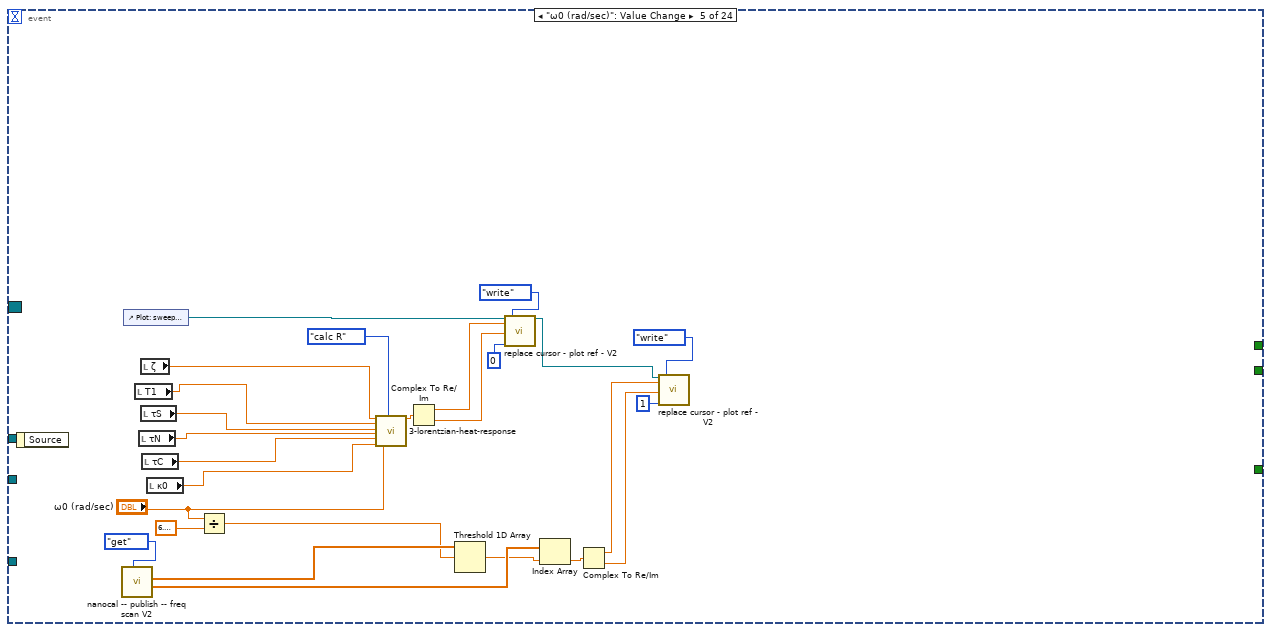
[diagram p7: hidden frame]
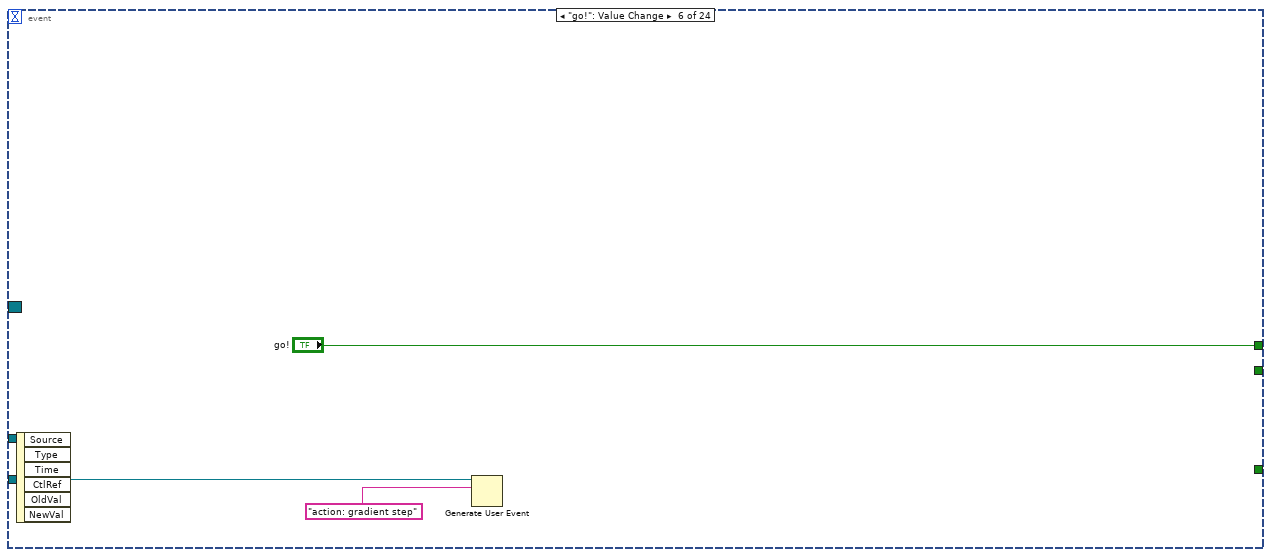
[diagram p8: hidden frame]
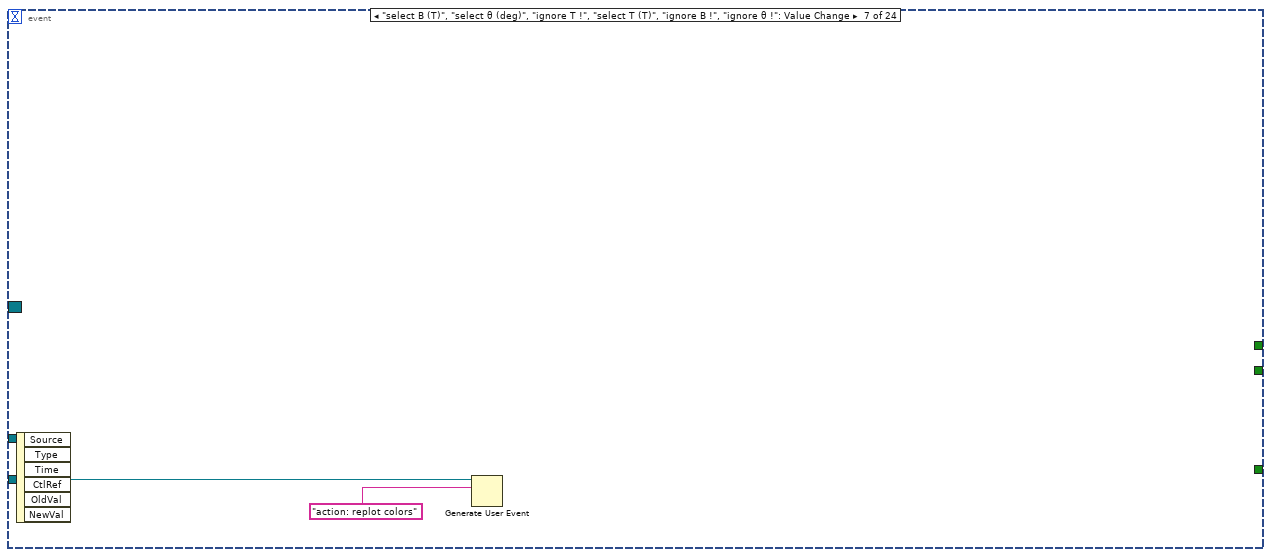
[diagram p9: hidden frame]
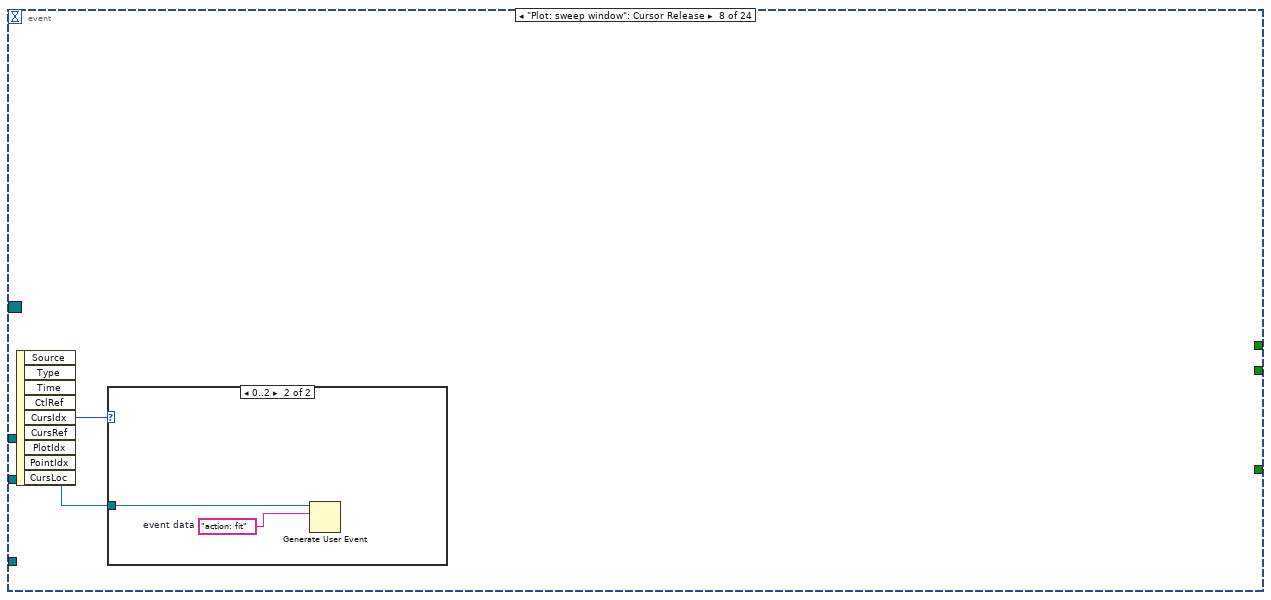
[diagram p10: hidden frame]
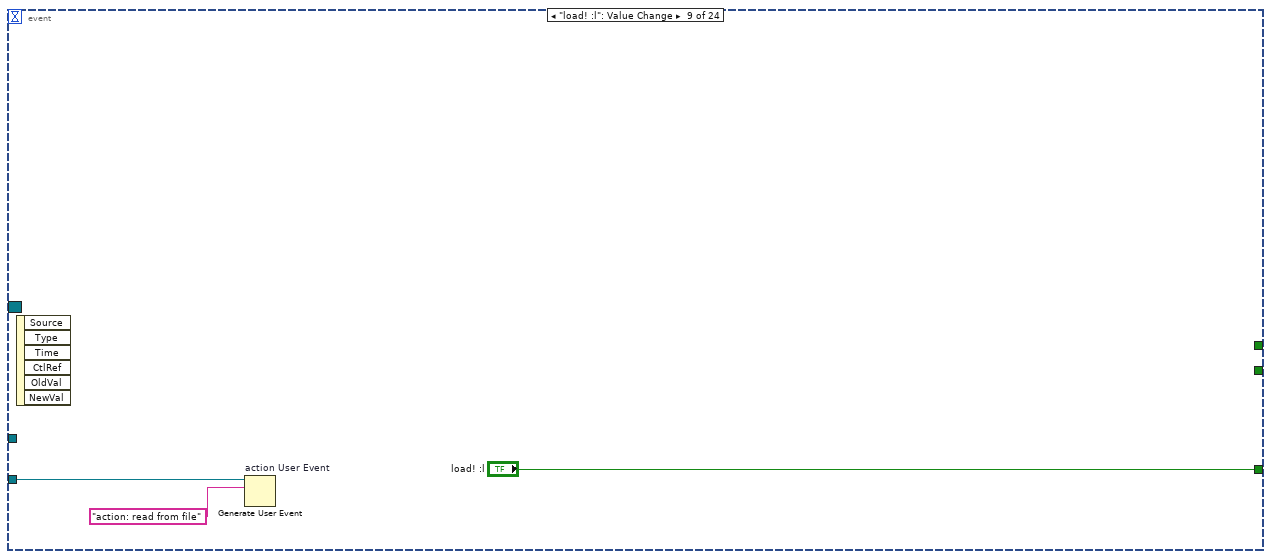
[diagram p12: hidden frame]
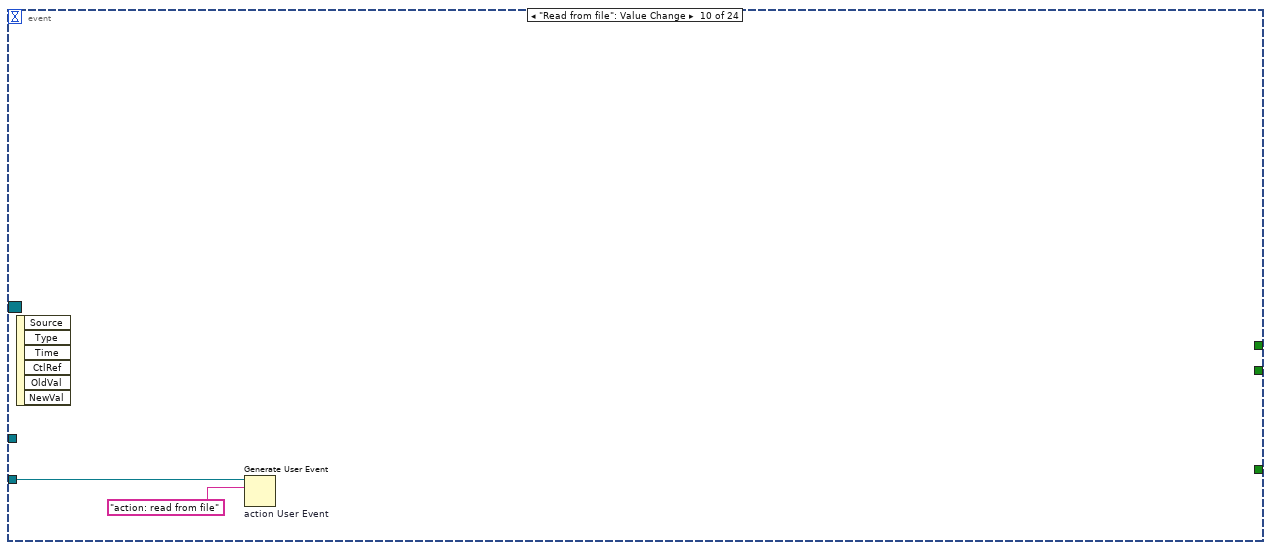
[diagram p13: hidden frame]
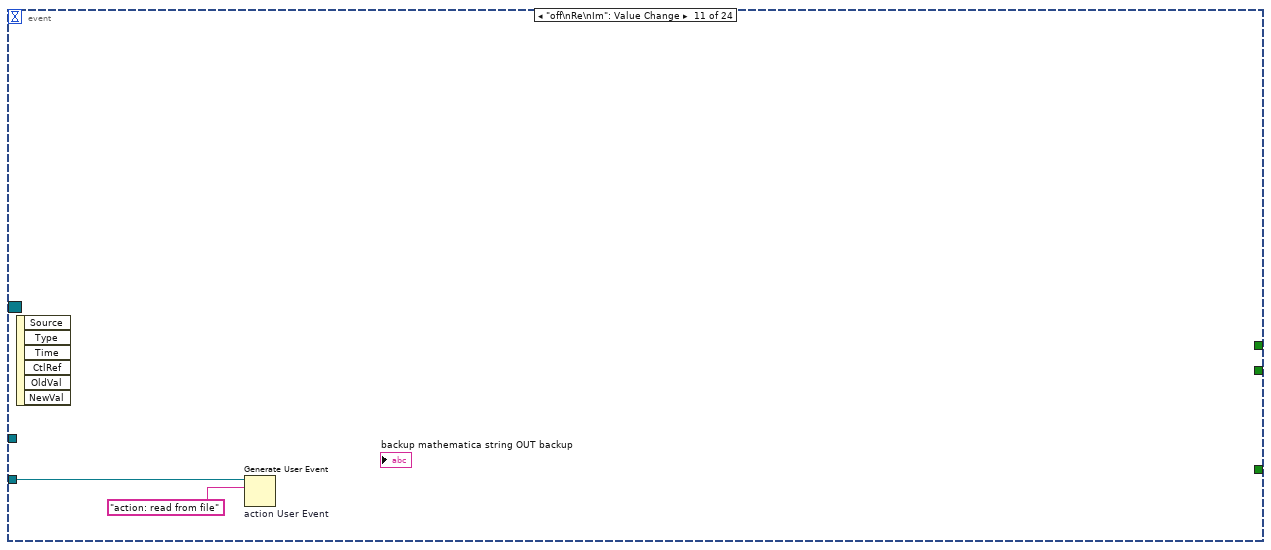
[diagram p14: hidden frame]
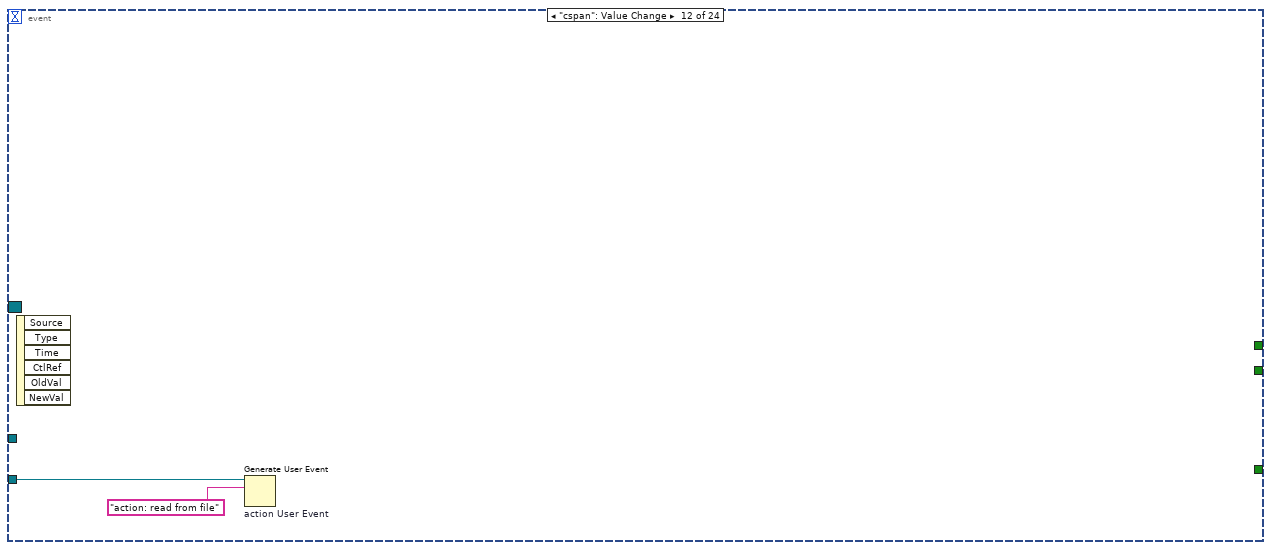
[diagram p15: hidden frame]
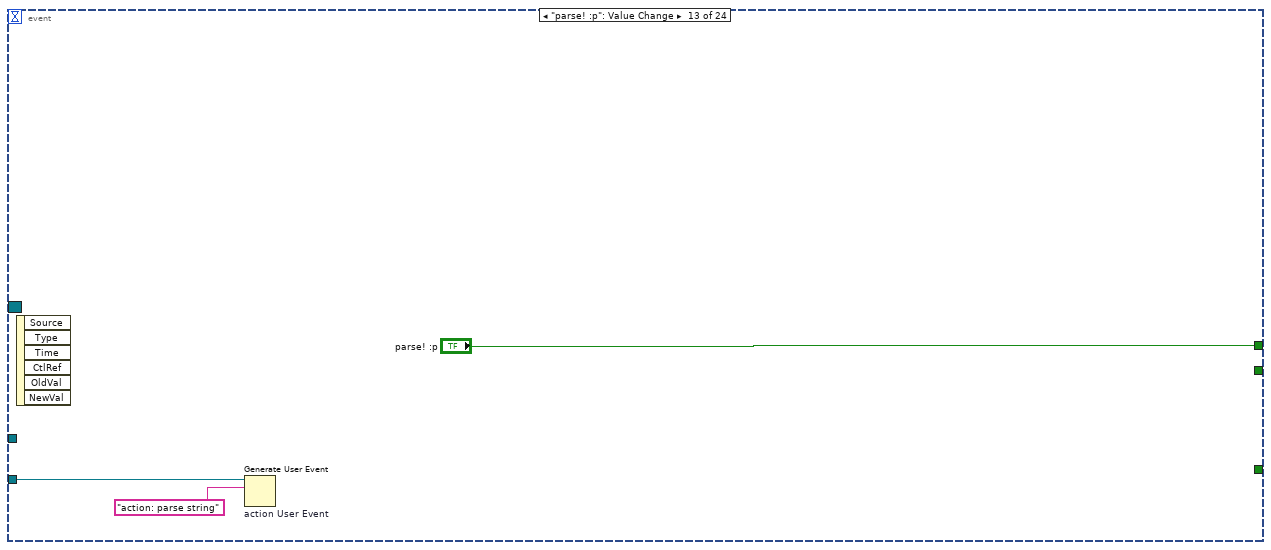
[diagram p16: hidden frame]
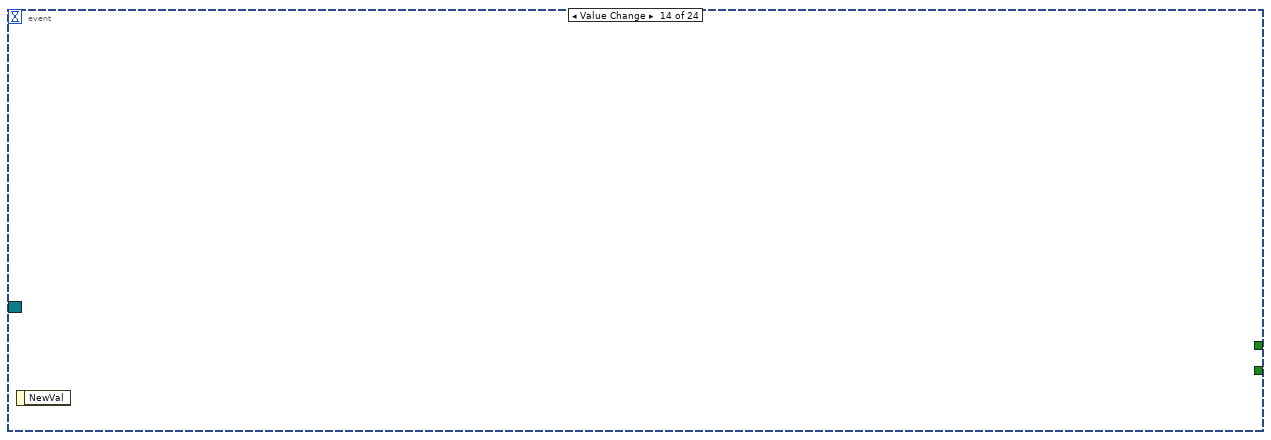
[diagram p17: hidden frame]
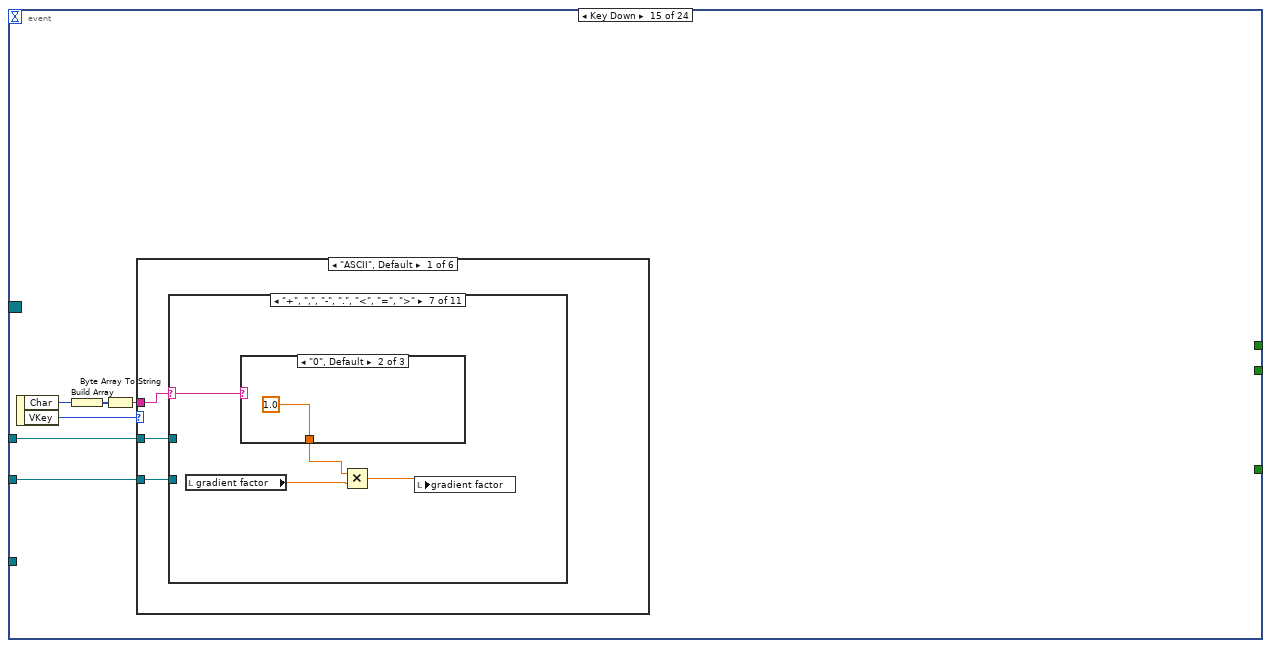
[diagram p18: hidden frame]
diagram:
  (unwired) cluster{"scaling":dbl, "what":T1} {"scaling"=1.0, "what"=enum."ζ"}
  (unwired) 3-lorentzian-parameters."ζ" ("X selector")
  w6 = map{T1, i32} {}  # Size: 0
  w5 = T1[] [enum."ζ", enum."τ1", enum."τS", enum."τN", enum."τC", enum."κ0", enum."m1", enum."m2", enum."m3"] items=["ζ", "τ1", "τS", "τN", "τC", "κ0", "m1", "m2", "m3", "T (K)", "B (T)", "θ (deg)"]
  w7 = FALSE ("newton pause")
  w9 = map{T1, dbl} {}  # Size: 0
  (unwired) 3-lorentzian-heat-response_action."dζ" ("derivative")
  (unwired) 3-lorentzian-heat-response_action."dζ" ("derivative")
  w10 = 0.0 ("new X")
  (unwired) T9[] [enum."dζ", enum."dT1", enum."dτS", enum."dτN", enum."dτC"] items=["calc R", "create string", "calc m1m2m3", "dζ", "dT1", "dτS", "dτN", "dτC", "d-all", "dκ0", "T(K)", "m1", "m2", "m3", "parse string", "θ (deg)", "B (T)"] ("Array")
  w24 = "void"  # interface
  w26 = "void"  # action
  # "action user event"
  # "action user event"
  n1 = control-ref of="Plot: sweep window"() -> (w16:refnum<vi>)
  n2 = Bundle By Name(cluster=T5 {"left"=0.0, "right "=0.0, "center"=0.0, "window"=0.0, "cursors"=[], "relative"=0, "absolute"=0, "fixed vertical offset"=0.0, "vertical offset"=0.0, "skew"=0.0, "default window frac"=0.0, "kind"=enum."symmetric", "skew.left"=0.0, "skew.right"=0.0, "Plot ref"=refnum, "wing order"=enum."forw"} ("cursor bracket: All, data window"), "Plot ref"=w16, "cursors"=i32[] [0, 1, 2], "fixed vertical offset"=0.0, "default window frac"=0.3 ("fixed vertical offset"), "kind"=enum16{"symmetric", "skewed", "fancy"}."symmetric") -> (w19:T5)
  n3 = control-ref of="cursor window"() -> (w15:refnum<vi>)
  n4 = for {
    shift-right: [w30] -> w3
    shift-left: w6 -> [w31]
    tunnel: w5 -> [w29] mode=indexing
    tunnel: i32[] [0, 1, 2, 3, 4, 5, 6, 7, 8] -> [w28] mode=indexing
    n5 = Insert Into Map(map in=w31, key=w29, value=w28) -> (map out=w30:map{T1, i32})  [unwired: 2 out]
  }
  n6 = local write "what"(cluster{"scaling":dbl, "what":T1}[] [{"scaling"=1.0, "what"=enum."ζ"}, {"scaling"=1.0, "what"=enum."τ1"}, {"scaling"=1.0, "what"=enum."τS"}, {"scaling"=1.0, "what"=enum."τN"}, {"scaling"=1.0, "what"=enum."τC"}, {"scaling"=1.0, "what"=enum."κ0"}]) -> ()
  n7 = Create User Event(user event datatype=w26) -> (user event=w14:refnum<user-event>)  [unwired: 1 in, 1 out]
  n8 = call "cursor window logic V3.vi"("cursor window action"=cursor_window_action."init", "cursor window in"=w15, "cursor window init"=w19) -> ()  [unwired: 7 in, 2 out]
  n9 = register-events(w14) -> (reference out=w27:refnum<event-registration>)  [unwired: 2 in, 1 out]
  n10 = Create User Event(user event datatype=w24) -> (user event=w1:refnum<user-event>)  [unwired: 1 in, 1 out]
  n11 = local write "cursor index map"(w3) -> ()
  n12 = control-ref of="Plot: sweep window"() -> (w11:refnum<vi>)
  n13 = register-events(w1) -> (reference out=w25:refnum<event-registration>)  [unwired: 2 in, 1 out]
  n14 = while "actions" {
    tunnel: w27 -> [w35]
    tunnel: w14 -> [w34]
    tunnel: w3 -> [_]
    tunnel: w1 -> [w32]
    stop <- w33 stop-if-true
    n15 = event shown="[0] <action>: User Event" {
      selector: w35 -> [_]
      dyn-events: _ -> [_]
      timeout: _ -> [_]
      tunnel: w34 -> [w38]
      tunnel: [w37] -> w33
      tunnel: w32 -> [w36]
      event User Event {
        n16 = event-data() -> ("action"=w39:string)  [unwired: 1 in]
        n17 = case shown="\"action: gradient step\"" w39 {
          tunnel: w38 -> [_ _ w158 w264 w280 w286 w369 _ _ w495 w534 _ w588 _ _]
          tunnel: [_ _ _ _ _ _ _ _ _ _ _ TRUE _ _ _] -> w37
          tunnel: w36 -> [_ _ w157 _ _ _ _ _ _ _ _ _ _ _ _]
          frame "action: new sweep" {
            w45 = T1[] [enum."T (K)", enum."B (T)", enum."θ (deg)"] items=["ζ", "τ1", "τS", "τN", "τC", "κ0", "m1", "m2", "m3", "T (K)", "B (T)", "θ (deg)"]
            w53 = T1[] [enum."ζ", enum."τ1", enum."τS", enum."τN", enum."τC", enum."κ0"] items=["ζ", "τ1", "τS", "τN", "τC", "κ0", "m1", "m2", "m3", "T (K)", "B (T)", "θ (deg)"]
            w88 = 6.283185307179586
            n18 = call "nanocal -- publish -- freq scan V2.vi"("publisher action"=publisher_action."get") -> ("dz/dω out (V)"=w89:cdb[], "z out (V)"=w83:cdb[], "ω out (Hz)"=w91:dbl[])  [unwired: 8 in]
            n19 = Divide(x=w89, y=w88) -> (x/y=w85:cdb[])
            n20 = Multiply(x=w91, y=w88) -> (x*y=w82:dbl[])
            n21 = local read "T1"() -> (w70:dbl)
            n22 = local read "τS"() -> (w69:dbl)
            n23 = local read "τN"() -> (w68:dbl)
            n24 = local read "τC"() -> (w67:dbl)
            n25 = local read "κ0"() -> (w66:dbl)
            n26 = local read "ζ"() -> (w71:dbl)
            n27 = Build Array(w71, w70, w69, w68, w67, w66) -> (w52:dbl[])
            n28 = for {
              shift-right: [w99] -> w51
              shift-left: map{T1, dbl} {} ("Map IN") -> [w100]
              tunnel: w53 -> [w97] mode=indexing
              tunnel: w52 -> [w98] mode=indexing
              tunnel: [w97] -> w40 mode=indexing
              n29 = Insert Into Map(map in=w100, key=w97, value=w98) -> (map out=w99:map{T1, dbl})  [unwired: 2 out]
            }
            n30 = local read "weighting"() -> (w84:T3)
            n31 = call "nanocal -- nuclear schottky goodness V3.vi"("weighting strategy"=w84, "dz/dω IN (V)"=w85, "Voltage IN (V)"=w83, "ω (rad/sec)"=w82, "parameters"=w52) -> ("R norm"=w81:dbl, "G"=w77:dbl, "derivatives"=w79:dbl[], "parameters OUT"=w80:dbl[], "R(ω) out"=w76:cdb[])  [unwired: 2 in]
            n32 = Multiply(x=w80, y=w79) -> (x*y=w78:dbl[])
            n33 = disable-structure shown="Disabled" {
              disable-tunnel: w83 -> [w108 _]
              disable-tunnel: w82 -> [w105 _]
              disable-tunnel: w76 -> [w101 _]
              frame Disabled {
                n34 = Complex To Polar(r * e^(i*theta)=w108) -> (theta=w107:dbl[])  [unwired: 1 out]
                n35 = Complex To Polar(r * e^(i*theta)=w101) -> (theta=w106:dbl[])  [unwired: 1 out]
                n36 = Bundle(w105, w107) -> (w104:cluster{dbl[], dbl[]})  [unwired: 1 in]
                n37 = Bundle(w105, w106) -> (w103:cluster{dbl[], dbl[]})  [unwired: 1 in]
                n38 = Build Array(w104, w103) -> (→"Plot: phase":cluster{dbl[], dbl[]}[])
                n39 = control-ref of="Plot: phase"() -> ()  [unwired: 1 out]
              }
              frame Enabled {
              }
            }
            n40 = Divide(x=w77, y=w81) -> (x/y=→"goodness":dbl)
            n41 = call "3-lorentzian-heat-response -- V4.vi"("action"=3-lorentzian-heat-response_action."calc m1m2m3", "Map IN"=w51) -> ("Map OUT"=w46:map{T1, dbl})  [unwired: 7 in, 2 out]
            n42 = Divide(x=w78, y=w77) -> (x/y=→"logarithmic derivatives":dbl[])
            n43 = local read "θ (deg)"() -> (w47:dbl)
            n44 = local read "B (T)"() -> (w48:dbl)
            n45 = local read "T (K)"() -> (w49:dbl)
            n46 = Build Array(w49, w48, w47) -> (w44:dbl[])
            n47 = local read "cursor x selector"() -> (w75:map{T1, dbl})
            n48 = control-ref of="Plot: sweep window"() -> (w65:refnum<vi>)
            n49 = local read "X selector"() -> (w74:T1)
            n50 = local read "cursor index map"() -> (w55:map{T1, i32})
            n51 = for {
              shift-right: [w95] -> w43
              shift-left: w46 -> [w96]
              tunnel: w45 -> [w94] mode=indexing
              tunnel: w44 -> [w93] mode=indexing
              n52 = Insert Into Map(map in=w96, key=w94, value=w93) -> (map out=w95:map{T1, dbl})  [unwired: 2 out]
            }
            n53 = local read "T (K)"() -> (w73:dbl)
            n54 = control-ref of="Plot:  colors"() -> (w90:refnum<vi>)
            n55 = Complex To Re/Im(x + iy=w83) -> (x=w64:dbl[], y=w63:dbl[])
            n56 = Look In Map(map=w75, key=w74, default value=w73) -> (value=w72:dbl)  [unwired: 1 out]
            n57 = call "replace plot - plot ref - V2.vi"("Plot ref in"=w65, "Array X IN"=w64, "Array Y IN"=w63, "plot index"=enum16{"data R(ω)", "fit R(ω)"}."data R(ω)" ("Plost: sweep window"), "cursor action"=cursor_action."write") -> ("Plot ref out"=w62:refnum<vi>)  [unwired: 11 in, 3 out]
            n58 = for {
              tunnel: w72 -> [w116]
              tunnel: w90 -> [w115]
              tunnel: w40 -> [w111] mode=indexing
              tunnel: w55 -> [w113]
              shift-right: [w110] -> _
              shift-left: w46 -> [w110]
              n59 = Look In Map(map=w110, key=w111) -> (value=w109:dbl)  [unwired: 1 in, 1 out]
              n60 = Look In Map(map=w113, key=w111) -> (value=w112:i32)  [unwired: 1 in, 1 out]
              n61 = call "replace cursor - plot ref - V2.vi"("Plot ref in"=w115, "new X"=w116, "new  Y"=w109, "cursor index"=w112, "cursor action"=cursor_action."write") -> ()  [unwired: 11 in, 4 out]
            }
            n62 = call "string parse mathematica assosiated array.vi"("derivative"=mathematica_string_map_action."create string", "Map IN"=w43) -> ("String OUT"=w41:string)  [unwired: 8 in, 1 out]
            n63 = Complex To Re/Im(x + iy=w76) -> (x=w60:dbl[], y=w59:dbl[])
            n64 = local write "String"(w41) -> ()
            n65 = call "replace plot - plot ref - V2.vi"("Plot ref in"=w62, "Array X IN"=w60, "Array Y IN"=w59, "plot index"=enum16{"data R(ω)", "fit R(ω)"}."fit R(ω)" ("Plost: sweep window"), "cursor action"=cursor_action."write") -> ()  [unwired: 11 in, 4 out]
          }
          frame "action: replot circles" {
            w146 = 6.283185307179586
            n66 = local read "T1"() -> (w133:dbl)
            n67 = local read "τS"() -> (w132:dbl)
            n68 = local read "κ0"() -> (w129:dbl)
            n69 = local read "τN"() -> (w131:dbl)
            n70 = local read "τC"() -> (w130:dbl)
            n71 = local read "ζ"() -> (w134:dbl)
            n72 = call "nanocal -- publish -- freq scan V2.vi"("publisher action"=publisher_action."get") -> ("dz/dω out (V)"=w147:cdb[], "z out (V)"=w143:cdb[], "ω out (Hz)"=w148:dbl[])  [unwired: 8 in]
            n73 = Divide(x=w147, y=w146) -> (x/y=w145:cdb[])
            n74 = Multiply(x=w148, y=w146) -> (x*y=w142:dbl[])
            n75 = Build Array(w134, w133, w132, w131, w130, w129) -> (w141:dbl[])
            n76 = local read "weighting"() -> (w144:T3)
            n77 = call "nanocal -- nuclear schottky goodness V3.vi"("weighting strategy"=w144, "dz/dω IN (V)"=w145, "Voltage IN (V)"=w143, "ω (rad/sec)"=w142, "parameters"=w141) -> ("R norm"=w140:dbl, "G"=w136:dbl, "derivatives"=w138:dbl[], "parameters OUT"=w139:dbl[], "R(ω) out"=w135:cdb[])  [unwired: 2 in]
            n78 = Multiply(x=w139, y=w138) -> (x*y=w137:dbl[])
            n79 = control-ref of="Plot: sweep window"() -> (w124:refnum<vi>)
            n80 = Divide(x=w136, y=w140) -> (x/y=w127:dbl)
            n81 = Divide(x=w137, y=w136) -> (x/y=w128:dbl[])
            n82 = Complex To Re/Im(x + iy=w143) -> (x=w122:dbl[], y=w121:dbl[])
            n83 = local write "logarithmic derivatives"(w128) -> ()
            n84 = local write "goodness"(w127) -> ()
            n85 = call "replace plot - plot ref - V2.vi"("Plot ref in"=w124, "Array X IN"=w122, "Array Y IN"=w121, "plot index"=enum16{"data R(ω)", "fit R(ω)"}."data R(ω)" ("Plost: sweep window"), "cursor action"=cursor_action."write") -> ("Plot ref out"=w123:refnum<vi>)  [unwired: 11 in, 3 out]
            n86 = Complex To Re/Im(x + iy=w135) -> (x=w120:dbl[], y=w119:dbl[])
            n87 = call "replace plot - plot ref - V2.vi"("Plot ref in"=w123, "Array X IN"=w120, "Array Y IN"=w119, "plot index"=enum16{"data R(ω)", "fit R(ω)"}."fit R(ω)" ("Plost: sweep window"), "cursor action"=cursor_action."write") -> ()  [unwired: 11 in, 4 out]
          }
          frame "action: gradient step" {
            w154 = 6.283185307179586
            w159 = FALSE ("newton pause")
            n88 = call "nanocal -- publish -- freq scan V2.vi"("publisher action"=publisher_action."get") -> ("dz/dω out (V)"=w156:cdb[], "z out (V)"=w151:cdb[], "ω out (Hz)"=w155:dbl[])  [unwired: 8 in]
            n89 = local write "newton pause"(w159) -> ()
            n90 = Generate User Event(user event=w158, event data cluster="action: new sweep" ("event data")) -> ()  [unwired: 2 in, 2 out]
            n91 = Divide(x=w156, y=w154) -> (x/y=w152:cdb[])
            n92 = Multiply(x=w155, y=w154) -> (x*y=w150:dbl[])
            n93 = for {
              N: "# steps" -> [_]
              tunnel: [TRUE ("newton pause")] -> w160
              tunnel: w159 -> [_]
              shift-right: [w191] -> _
              shift-left: w157 -> [w191]
              tunnel: w152 -> [w174]
              tunnel: w151 -> [w173]
              tunnel: w150 -> [w172]
              stop <- w199 stop-if-true
              (unwired) 3-lorentzian-parameters."κ0" ("Plost: sweep window")
              (unwired) 3-lorentzian-parameters."τC" ("Plost: sweep window")
              (unwired) 3-lorentzian-parameters."τN" ("Plost: sweep window")
              (unwired) 3-lorentzian-parameters."τS" ("Plost: sweep window")
              (unwired) 3-lorentzian-parameters."τ1" ("Plost: sweep window")
              (unwired) 3-lorentzian-parameters."ζ" ("Plost: sweep window")
              w168 = T1[] [enum."ζ", enum."τ1", enum."τS", enum."τN", enum."τC", enum."κ0"] items=["ζ", "τ1", "τS", "τN", "τC", "κ0", "m1", "m2", "m3", "T (K)", "B (T)", "θ (deg)"]
              n94 = local read "newton pause"() -> (w199:bool)
              n95 = local read "T1"() -> (w204:dbl)
              n96 = local read "τS"() -> (w203:dbl)
              n97 = local read "τN"() -> (w202:dbl)
              n98 = local read "τC"() -> (w201:dbl)
              n99 = local read "κ0"() -> (w200:dbl)
              n100 = local read "ζ"() -> (w205:dbl)
              n101 = Build Array(w205, w204, w203, w202, w201, w200) -> (w176:dbl[])
              n102 = for {
                shift-right: [w230] -> w175
                shift-left: map{T1, dbl} {} ("Map IN") -> [w231]
                tunnel: w168 -> [w228] mode=indexing
                tunnel: w176 -> [w229] mode=indexing
                tunnel: [w228] -> w167 mode=indexing
                n103 = Insert Into Map(map in=w231, key=w228, value=w229) -> (map out=w230:map{T1, dbl})  [unwired: 2 out]
              }
              n104 = call "nanocal -- nuclear schottky goodness V4.vi"("parameters IN"=w175, "weighting strategy"="weighting", "dz/dω IN (V)"=w174, "Voltage IN (V)"=w173, "ω (rad/sec)"=w172) -> ("R norm"=w165:dbl, "G"=w166:dbl, "R(ω) out"=w171:cdb[], "derivatives OUT"=w170:map{T1, dbl})  [unwired: 3 in]
              n105 = local read "what"() -> (w217:cluster{"scaling":dbl, "what":T1}[])
              n106 = Divide(x=w166, y=w165) -> (x/y=w164:dbl)
              n107 = Complex To Re/Im(x + iy=w171) -> (x=w188:dbl[], y=w187:dbl[])
              n108 = control-ref of="Plot: sweep window"() -> (w190:refnum<vi>)
              n109 = call "3-lorentzian-heat-response -- V4.vi"("action"=3-lorentzian-heat-response_action."calc m1m2m3", "Map IN"=w175) -> ("Map OUT"=w179:map{T1, dbl})  [unwired: 7 in, 2 out]
              n110 = local write "goodness"(w164) -> ()
              n111 = for {
                tunnel: w217 -> [w241] mode=indexing
                tunnel: [w240] -> w216 mode=indexing
                n112 = Unbundle By Name(w241) -> ("scaling"=w240:dbl)
              }
              n113 = for {
                tunnel: w167 -> [w226] mode=indexing
                shift-right: [w227] -> _
                shift-left: w170 -> [w227]
                tunnel: [w225] -> w169 mode=indexing
                n114 = Look In Map(map=w227, key=w226) -> (value=w225:dbl)  [unwired: 1 in, 1 out]
              }
              n115 = local read "cursor x selector"() -> (w184:map{T1, dbl})
              n116 = local read "X selector"() -> (w183:T1)
              n117 = local read "cursor index map"() -> (w180:map{T1, i32})
              n118 = call "replace plot - plot ref - V2.vi"("Plot ref in"=w190, "Array X IN"=w188, "Array Y IN"=w187, "plot index"=enum16{"data R(ω)", "fit R(ω)"}."fit R(ω)" ("Plost: sweep window"), "cursor action"=cursor_action."write") -> ()  [unwired: 11 in, 4 out]
              n119 = local read "T (K)"() -> (w182:dbl)
              n120 = control-ref of="Plot:  colors"() -> (w185:refnum<vi>)
              n121 = Multiply(x=w216, y=w169) -> (x*y=w215:dbl[])
              n122 = Look In Map(map=w184, key=w183, default value=w182) -> (value=w181:dbl)  [unwired: 1 out]
              n123 = Multiply(x=w215, y="gradient factor") -> (x*y=w220:dbl[])
              n124 = for {
                tunnel: w181 -> [w239]
                tunnel: w185 -> [w238]
                tunnel: w168 -> [w234] mode=indexing
                tunnel: w180 -> [w236]
                shift-right: [w233] -> _
                shift-left: w179 -> [w233]
                n125 = Look In Map(map=w233, key=w234) -> (value=w232:dbl)  [unwired: 1 in, 1 out]
                n126 = Look In Map(map=w236, key=w234) -> (value=w235:i32)  [unwired: 1 in, 1 out]
                n127 = call "replace cursor - plot ref - V2.vi"("Plot ref in"=w238, "new X"=w239, "new  Y"=w232, "cursor index"=w235, "cursor action"=cursor_action."write") -> ()  [unwired: 11 in, 4 out]
              }
              n128 = Subtract(x=1.0 ("index"), y=w220) -> (x-y=w213:dbl[])
              n129 = Index Array(array=w213, index #1=3-lorentzian-parameters."ζ" ("Plost: sweep window"), index #2=3-lorentzian-parameters."τ1" ("Plost: sweep window"), index #3=3-lorentzian-parameters."τS" ("Plost: sweep window"), index #4=3-lorentzian-parameters."τN" ("Plost: sweep window"), index #5=3-lorentzian-parameters."τC" ("Plost: sweep window"), index #6=3-lorentzian-parameters."κ0" ("Plost: sweep window")) -> (element #1=w214:dbl, element #2=w212:dbl, element #3=w211:dbl, element #4=w210:dbl, element #5=w209:dbl, element #6=w207:dbl)
              n130 = Multiply(x=w214, y=w205) -> (x*y=w224:dbl)
              n131 = Multiply(x=w212, y=w204) -> (x*y=w223:dbl)
              n132 = local write "logarithmic derivatives"(w169) -> ()
              n133 = Multiply(x=w211, y=w203) -> (x*y=w222:dbl)
              n134 = Multiply(x=w210, y=w202) -> (x*y=w221:dbl)
              n135 = Multiply(x=w209, y=w201) -> (x*y=w218:dbl)
              n136 = Multiply(x=w207, y=w200) -> (x*y=w208:dbl)
              n137 = local write "τN"(w221) -> ()
              n138 = local write "τC"(w218) -> ()
              n139 = local write "τS"(w222) -> ()
              n140 = local write "κ0"(w208) -> ()
              n141 = local write "T1"(w223) -> ()
              n142 = local write "ζ"(w224) -> ()
            }
            n143 = local write "newton pause"(w160) -> ()
          }
          frame "action: uco" {
            (unwired) 3-lorentzian-parameters."κ0" ("Plost: sweep window")
            n144 = Generate User Event(user event=w264, event data cluster="action: new sweep" ("event data")) -> ()  [unwired: 2 in, 2 out]
            n145 = local read "T1"() -> (w256:dbl)
            n146 = local read "τN"() -> (w254:dbl)
            n147 = local read "τC"() -> (w253:dbl)
            n148 = local read "κ0"() -> (w252:dbl)
            n149 = local read "τS"() -> (w255:dbl)
            n150 = local read "ζ"() -> (w257:dbl)
            n151 = call "3-lorentzian-parameters - manage.vi"("ζ"=w257, "T1"=w256, "τS"=w255, "τN"=w254, "τC"=w253, "κ0"=w252, "parameters"=3-lorentzian-parameters_--_action."to array") -> ("parameter array OUT"=w250:dbl[])  [unwired: 6 in, 6 out]
            n152 = Natural Logarithm(1:w250) -> (0:w262:dbl[])
            n153 = vi-ref "nanocal -- nuclear schottky goodness -- for UCO -- V3.vi"() -> (w263:refnum<vi>)
            n154 = call-poly <vilib>:"Unconstrained Optimization.vi"("function data"=T15 variant, "objective function"=w263, "start"=w262) -> ("f(minimum)"=w260:dbl, "minimum"=w261:dbl[])  [unwired: 5 in, 2 out]
            n155 = Exponential(1:w260) -> (0:w259:dbl)
            n156 = Exponential(1:w261) -> (0:w249:dbl[])
            n157 = call "3-lorentzian-parameters - manage.vi"("parameter array"=w249, "parameters"=3-lorentzian-parameters_--_action."to parameters") -> ("ζ OUT"=w248:dbl, "T1 OUT"=w247:dbl, "τS  OUT"=w246:dbl, "τN  OUT"=w245:dbl, "τC  OUT"=w244:dbl, "κ0  OUT"=w243:dbl)  [unwired: 11 in, 1 out]
            n158 = local write "goodness"(w259) -> ()
            n159 = local write "T1"(w247) -> ()
            n160 = local write "τN"(w245) -> ()
            n161 = local write "τC"(w244) -> ()
            n162 = local write "κ0"(w243) -> ()
            n163 = local write "τS"(w246) -> ()
            n164 = local write "ζ"(w248) -> ()
          }
          frame "action: parse string" {
            n165 = local read "String"() -> (w282:string)
            n166 = call "string parse mathematica assosiated array.vi"("derivative"=mathematica_string_map_action."parse string", "String in"=w282) -> ("Map OUT"=w276:map{T1, dbl})  [unwired: 8 in, 1 out]
            n167 = Generate User Event "action User Event"(user event=w280, event data cluster="action: replot colors" ("event data")) -> ()  [unwired: 2 in, 2 out]
            n168 = Look In Map(map=w276, key=3-lorentzian-parameters."ζ" ("Plost: sweep window")) -> (value=w271:dbl)  [unwired: 1 in, 1 out]
            n169 = Look In Map(map=w276, key=3-lorentzian-parameters."τ1" ("Plost: sweep window")) -> (value=w270:dbl)  [unwired: 1 in, 1 out]
            n170 = Look In Map(map=w276, key=3-lorentzian-parameters."τS" ("Plost: sweep window")) -> (value=w269:dbl)  [unwired: 1 in, 1 out]
            n171 = Look In Map(map=w276, key=3-lorentzian-parameters."τN" ("Plost: sweep window")) -> (value=w268:dbl)  [unwired: 1 in, 1 out]
            n172 = Look In Map(map=w276, key=3-lorentzian-parameters."τC" ("Plost: sweep window")) -> (value=w267:dbl)  [unwired: 1 in, 1 out]
            n173 = Look In Map(map=w276, key=3-lorentzian-parameters."κ0" ("Plost: sweep window")) -> (value=w266:dbl)  [unwired: 1 in, 1 out]
            n174 = local write "ζ"(w271) -> ()
            n175 = local write "T1"(w270) -> ()
            n176 = local write "τS"(w269) -> ()
            n177 = local write "τN"(w268) -> ()
            n178 = local write "τC"(w267) -> ()
            n179 = local write "κ0"(w266) -> ()
          }
          frame "action: read mathematica string" {
            w291 = map{T1, dbl} {}  # Size: 0
            w288 = set{dbl} {}  # Size: 0
            w294 = map{i32, map{T1, dbl}} {}  # Size: 0
            w295 = map{i32, string} {}  # Size: 0
            n180 = call "string parse mathematica list assosiated array.vi"("derivative"=3-lorentzian-heat-response_action."parse string", "string IN"="string IN") -> ("Map OUT"=w296:map{i32, map{T1, dbl}})  [unwired: 8 in, 1 out]
            n181 = List Folder(path="folder", pattern="file pattern") -> (filenames=w297:string[])  [unwired: 2 in, 3 out]
            n182 = Generate User Event(user event=w286, event data cluster="action: update enums" ("event data")) -> ()  [unwired: 2 in, 2 out]
            n183 = for {
              tunnel: w297 -> [w325] mode=indexing
              shift-right: [w328] -> w283
              shift-left: w296 -> [w330]
              shift-right: [w326] -> w292
              shift-left: w295 -> [w327]
              shift-right: [w304] -> w284
              shift-left: w294 -> [w305]
              shift-right: [w311] -> w289
              shift-left: w288 -> [w312]
              shift-right: [w314] -> w290
              shift-left: w288 -> [w315]
              tunnel: w291 -> [w319]
              shift-right: [w308] -> w285
              shift-left: w288 -> [w309]
              n184 = call "filename-manage.vi"("filename-action"=filename-action."get T", "file name IN"=w325) -> ("number OUT"=w310:dbl, "filename OUT"=w323:string)  [unwired: 7 in, 1 out]
              n185 = call "filename-manage.vi"("filename-action"=filename-action."get B", "file name IN"=w323) -> ("number OUT"=w316:dbl, "filename OUT"=w322:string)  [unwired: 7 in, 1 out]
              n186 = Insert Into Map(map in=w319, key=3-lorentzian-parameters."T (K)", value=w310) -> (map out=w318:map{T1, dbl})  [unwired: 2 out]
              n187 = Insert Into Map(map in=w318, key=3-lorentzian-parameters."B (T)", value=w316) -> (map out=w317:map{T1, dbl})  [unwired: 2 out]
              n188 = call "filename-manage.vi"("filename-action"=filename-action."get deg", "file name IN"=w322) -> ("number OUT"=w313:dbl, "filename OUT"=w334:string)  [unwired: 7 in, 1 out]
              n189 = Insert Into Map(map in=w317, key=3-lorentzian-parameters."θ (deg)", value=w313) -> (map out=w307:map{T1, dbl})  [unwired: 2 out]
              n190 = call "filename-manage.vi"("filename-action"=filename-action."get ind", "file name IN"=w334) -> ("number OUT"=w329:dbl)  [unwired: 7 in, 2 out]
              n191 = To Long Integer(number=w329) -> (32bit integer=w306:i32)
              n192 = in-place {
                in-place-border: w316 -> [w368]
                in-place-border: w313 -> [w367]
                in-place-border: w310 -> [w361]
                in-place-border: [w360] -> w321
                n193 = in-place-map #1(w330, w306) -> (w363:map{T1, dbl}, w360:bool)  [unwired: 1 in]
                n194 = Insert Into Map(map in=w363, key=3-lorentzian-parameters."T (K)", value=w361) -> (map out=w362:map{T1, dbl})  [unwired: 2 out]
                n195 = Insert Into Map(map in=w362, key=3-lorentzian-parameters."B (T)", value=w368) -> (map out=w364:map{T1, dbl})  [unwired: 2 out]
                n196 = Insert Into Map(map in=w364, key=3-lorentzian-parameters."θ (deg)", value=w367) -> (map out=w366:map{T1, dbl})  [unwired: 2 out]
                n197 = in-place-map #1(w366, LVMapReplaceAction."Modify Entry only if found" ("action")) -> (w328:map{i32, map{T1, dbl}})  [unwired: 2 out]
              }
              n198 = Not(x=w321) -> (.not. x?=w320:bool)
              n199 = case shown="True" w320 {
                tunnel: w327 -> [w339 w356]
                tunnel: [w339 w355] -> w326
                tunnel: w325 -> [_ w354]
                tunnel: w306 -> [_ w353]
                tunnel: w316 -> [_ w352]
                tunnel: w315 -> [w337 w351]
                tunnel: [w337 w350] -> w314
                tunnel: w313 -> [_ w349]
                tunnel: w312 -> [w338 w348]
                tunnel: [w338 w347] -> w311
                tunnel: w310 -> [_ w346]
                tunnel: [w335 w345] -> w308
                tunnel: w309 -> [w335 w344]
                tunnel: w307 -> [_ w343]
                tunnel: w306 -> [_ w342]
                tunnel: w305 -> [w336 w341]
                tunnel: [w336 w340] -> w304
                frame False {
                }
                frame True {
                  n200 = Insert Into Set(10:w346, 11:w344) -> (3:w345:set{dbl})  [unwired: 1 out]
                  n201 = Insert Into Set(10:w352, 11:w351) -> (3:w350:set{dbl})  [unwired: 1 out]
                  n202 = Insert Into Set(10:w349, 11:w348) -> (3:w347:set{dbl})  [unwired: 1 out]
                  n203 = Insert Into Map(map in=w341, key=w342, value=w343) -> (map out=w340:map{i32, map{T1, dbl}})  [unwired: 2 out]
                  n204 = Insert Into Map(map in=w356, key=w353, value=w354) -> (map out=w355:map{i32, string})  [unwired: 2 out]
                }
              }
            }
            "filenames" <- w292
            "Set of B's" <- w290
            "Set of θ's" <- w289
            "Set of T's" <- w285
            "temps&degs" <- w284
            n205 = local write "mathematica thing"(w283) -> ()
          }
          frame "action: update enums" {
            w374 = map{i32, dbl} {}  # Size: 0
            (unwired) set{dbl} {0.0, 5.0, 10.0, 15.0, 20.0, 25.0, 30.0, 35.0} ("Set of B's")
            w382 = map{i32, i32} {}  # Size: 0
            w381 = map{i32, dbl} {}  # Size: 0
            w380 = map{i32, dbl} {}  # Size: 0
            n206 = local read "temps&degs"() -> (w378:map{i32, map{T1, dbl}})
            n207 = local read "X selector"() -> (w377:T1)
            n208 = local read "filenames"() -> (w379:map{i32, string})
            n209 = Generate User Event(user event=w369, event data cluster="action: replot colors" ("event data")) -> ()  [unwired: 2 in, 2 out]
            n210 = for {
              tunnel: [w422] -> w389 mode=indexing
              tunnel: [w419] -> w387 mode=indexing
              tunnel: [w416] -> w391 mode=indexing
              tunnel: w377 -> [w420]
              tunnel: w379 -> [w418] mode=indexing
              tunnel: w378 -> [w417]
              n211 = Unbundle(w418) -> ("32bit integer"=w416:i32, "file pattern"=w422:string)
              n212 = Look In Map(map=w417, key=w416) -> (value=w421:map{T1, dbl})  [unwired: 1 in, 1 out]
              n213 = Look In Map(map=w421, key=w420) -> (value=w419:dbl)  [unwired: 1 in, 1 out]
            }
            n214 = call "array - sorted inexes.vi"("x"=w387) -> ("index array"=w388:i32[])  [unwired: 9 in, 1 out]
            n215 = local read "Set of T's"() -> (w373:set{dbl})
            n216 = local read "Set of B's"() -> (w375:set{dbl})
            n217 = local read "Set of θ's"() -> (w376:set{dbl})
            n218 = for {
              tunnel: w388 -> [w402] mode=indexing
              tunnel: w389 -> [w405]
              tunnel: [w404] -> w390 mode=indexing
              tunnel: w391 -> [w403]
              shift-right: [w398] -> w392
              shift-left: w382 -> [w401]
              i -> [w400]
              n219 = Index Array(array=w405, index=w402) -> (element=w404:string)
              n220 = Index Array(array=w403, index=w402) -> (element=w399:i32)
              n221 = Insert Into Map(map in=w401, key=w400, value=w399) -> (map out=w398:map{i32, i32})  [unwired: 2 out]
            }
            "filesnames lookup" <- w392
            n222 = for {
              shift-right: [w396] -> w372
              shift-left: w374 -> [w397]
              tunnel: [w394] -> w371 mode=indexing
              tunnel: w373 -> [w393] mode=indexing
              i -> [w395]
              n223 = Insert Into Map(map in=w397, key=w395, value=w393) -> (map out=w396:map{i32, dbl})  [unwired: 2 out]
              n224 = Number To Fractional String(number=w393) -> (F-format string=w394:string)  [unwired: 3 in]
            }
            "T lookup" <- w372
            n225 = for {
              shift-right: [w409] -> w386
              shift-left: w381 -> [w410]
              tunnel: [w407] -> w385 mode=indexing
              tunnel: w375 -> [w406] mode=indexing
              i -> [w408]
              n226 = Insert Into Map(map in=w410, key=w408, value=w406) -> (map out=w409:map{i32, dbl})  [unwired: 2 out]
              n227 = Number To Fractional String(number=w406) -> (F-format string=w407:string)  [unwired: 3 in]
            }
            "B lookup" <- w386
            n228 = for {
              shift-right: [w414] -> w384
              shift-left: w380 -> [w415]
              tunnel: [w412] -> w383 mode=indexing
              tunnel: w376 -> [w411] mode=indexing
              i -> [w413]
              n229 = Insert Into Map(map in=w415, key=w413, value=w411) -> (map out=w414:map{i32, dbl})  [unwired: 2 out]
              n230 = Number To Fractional String(number=w411) -> (F-format string=w412:string)  [unwired: 3 in]
            }
            "θ lookup" <- w384
            n231 = property on="select T (T)" class="Ring (strict)"("Strings []"=w371) -> ()  [unwired: 2 in, 2 out]
            n232 = property on="select B (T)" class="Ring (strict)"("Strings []"=w385) -> ()  [unwired: 2 in, 2 out]
            n233 = property on="select θ (deg)" class="Ring (strict)"("Strings []"=w383) -> ()  [unwired: 2 in, 2 out]
            n234 = property on="filenames" class="Ring (strict)"("Strings []"=w390) -> ()  [unwired: 2 in, 2 out]
          }
          frame "action: write mathematica string" {
            n235 = local read "mathematica thing"() -> (w424:map{i32, map{T1, dbl}})
            n236 = call "string parse mathematica list assosiated array.vi"("derivative"=3-lorentzian-heat-response_action."create string", "Map IN"=w424) -> ("string out"=→"string OUT":string)  [unwired: 8 in, 1 out]
          }
          frame "action: replot colors" {
            w429 = T1[] [enum."ζ", enum."τ1", enum."τS", enum."τN", enum."τC"] items=["ζ", "τ1", "τS", "τN", "τC", "κ0", "m1", "m2", "m3", "T (K)", "B (T)", "θ (deg)"]
            n237 = local read "mathematica thing"() -> (w443:map{i32, map{T1, dbl}})
            n238 = local read "select θ (deg)"() -> (w441:u16)
            n239 = local read "ignore T !"() -> (w433:bool)
            n240 = local read "select B (T)"() -> (w438:u16)
            n241 = local read "select T (T)"() -> (w435:u16)
            n242 = local read "ignore B !"() -> (w432:bool)
            n243 = local read "θ lookup"() -> (w442:map{i32, dbl})
            n244 = local read "ignore θ !"() -> (w431:bool)
            n245 = local read "X selector"() -> (w430:T1)
            n246 = local read "T lookup"() -> (w436:map{i32, dbl})
            n247 = local read "B lookup"() -> (w439:map{i32, dbl})
            n248 = Look In Map(map=w436, key=w435) -> (value=w434:dbl)  [unwired: 1 in, 1 out]
            n249 = Look In Map(map=w442, key=w441) -> (value=w440:dbl)  [unwired: 1 in, 1 out]
            n250 = Look In Map(map=w439, key=w438) -> (value=w437:dbl)  [unwired: 1 in, 1 out]
            n251 = for {
              tunnel: w443 -> [w464]
              tunnel: w440 -> [w460]
              tunnel: 3-lorentzian-parameters."θ (deg)" ("Plost: sweep window") -> [w459]
              tunnel: w430 -> [w458]
              tunnel: 3-lorentzian-parameters."B (T)" ("Plost: sweep window") -> [w457]
              tunnel: w437 -> [w456]
              tunnel: 3-lorentzian-parameters."T (K)" ("Plost: sweep window") -> [w455]
              tunnel: w434 -> [w454]
              tunnel: w433 -> [w453]
              tunnel: w432 -> [w452]
              tunnel: w431 -> [w451]
              tunnel: w429 -> [w445] mode=indexing
              n252 = for {
                tunnel: w464 -> [w494] mode=indexing
                tunnel: w445 -> [w493]
                tunnel: [w492] -> w463 mode=indexing if=w470
                tunnel: [w491] -> w462 mode=indexing if=w470
                tunnel: w460 -> [w489]
                tunnel: w459 -> [w488]
                tunnel: w458 -> [w487]
                tunnel: w457 -> [w485]
                tunnel: w456 -> [w484]
                tunnel: w455 -> [w482]
                tunnel: w454 -> [w474]
                tunnel: w453 -> [w473]
                tunnel: w452 -> [w481]
                tunnel: w451 -> [w479]
                n253 = Unbundle(w494) -> ("Map"=w483:map{T1, dbl})  [unwired: 1 out]
                n254 = Look In Map(map=w483, key=w485) -> (value=w486:dbl)  [unwired: 1 in, 1 out]
                n255 = Look In Map(map=w483, key=w487) -> (value=w492:dbl)  [unwired: 1 in, 1 out]
                n256 = Look In Map(map=w483, key=w488) -> (value=w490:dbl)  [unwired: 1 in, 1 out]
                n257 = Look In Map(map=w483, key=w493) -> (value=w491:dbl)  [unwired: 1 in, 1 out]
                n258 = Look In Map(map=w483, key=w482) -> (value=w475:dbl)  [unwired: 1 in, 1 out]
                n259 = Equal?(x=w486, y=w484) -> (x = y?=w480:bool)
                n260 = Equal?(x=w475, y=w474) -> (x = y?=w472:bool)
                n261 = Equal?(x=w490, y=w489) -> (x = y?=w478:bool)
                n262 = Or(x=w473, y=w472) -> (x .or. y?=w471:bool)
                n263 = Or(x=w481, y=w480) -> (x .or. y?=w477:bool)
                n264 = Or(x=w479, y=w478) -> (x .or. y?=w476:bool)
                n265 = Compound Arithmetic op=AND(w471, w477, w476) -> (w470:bool)
              }
              n266 = local read "cursor index map"() -> (w446:map{T1, i32})
              n267 = call "array - sorted inexes.vi"("x"=w463) -> ("index array"=w461:i32[])  [unwired: 9 in, 1 out]
              n268 = for {
                tunnel: w463 -> [w469]
                tunnel: w462 -> [w468]
                tunnel: w461 -> [w465] mode=indexing
                tunnel: [w467] -> w449 mode=indexing
                tunnel: [w466] -> w448 mode=indexing
                n269 = Index Array(array=w469, index=w465) -> (element=w467:dbl)
                n270 = Index Array(array=w468, index=w465) -> (element=w466:dbl)
              }
              n271 = Look In Map(map=w446, key=w445) -> (value=w444:i32)  [unwired: 1 in, 1 out]
              n272 = control-ref of="Plot:  colors"() -> (w447:refnum<vi>)
              n273 = call "replace plot - plot ref - V2.vi"("Plot ref in"=w447, "Array X IN"=w449, "Array Y IN"=w448, "plot index"=w444, "cursor action"=cursor_action."write") -> ()  [unwired: 11 in, 4 out]
            }
          }
          frame "action: copy from math" {
            (unwired) 3-lorentzian-heat-response_action."dζ" ("derivative")
            n274 = local read "mathematica thing"() -> (w500:map{i32, map{T1, dbl}})
            n275 = local read "file index"() -> (w499:i32)
            n276 = Look In Map(map=w500, key=w499) -> (key not found?=w497:bool, value=w498:map{T1, dbl})  [unwired: 1 in]
            n277 = Generate User Event(user event=w495, event data cluster="action: new sweep" ("event data")) -> ()  [unwired: 2 in, 2 out]
            n278 = case shown="False" w497 {
              tunnel: w498 -> [w506 _]
              frame False {
                n279 = Look In Map(map=w506, key=3-lorentzian-parameters."ζ" ("Plost: sweep window")) -> (value=w507:dbl)  [unwired: 1 in, 1 out]
                n280 = Look In Map(map=w506, key=3-lorentzian-parameters."τ1" ("Plost: sweep window")) -> (value=w505:dbl)  [unwired: 1 in, 1 out]
                n281 = Look In Map(map=w506, key=3-lorentzian-parameters."τS" ("Plost: sweep window")) -> (value=w504:dbl)  [unwired: 1 in, 1 out]
                n282 = Look In Map(map=w506, key=3-lorentzian-parameters."τN" ("Plost: sweep window")) -> (value=w503:dbl)  [unwired: 1 in, 1 out]
                n283 = Look In Map(map=w506, key=3-lorentzian-parameters."τC" ("Plost: sweep window")) -> (value=w502:dbl)  [unwired: 1 in, 1 out]
                n284 = Look In Map(map=w506, key=3-lorentzian-parameters."κ0" ("Plost: sweep window")) -> (value=w501:dbl)  [unwired: 1 in, 1 out]
                n285 = local write "ζ"(w507) -> ()
                n286 = local write "T1"(w505) -> ()
                n287 = local write "τS"(w504) -> ()
                n288 = local write "τN"(w503) -> ()
                n289 = local write "τC"(w502) -> ()
                n290 = local write "κ0"(w501) -> ()
              }
              frame True {
              }
            }
          }
          frame "action: copy to math" {
            (unwired) 0.0
            (unwired) 0.0
            w524 = 0.0
            w519 = T1[] [enum."ζ", enum."τ1", enum."τS", enum."τN", enum."τC", enum."κ0", enum."m1", enum."m2", enum."m3", enum."T (K)", enum."B (T)", enum."θ (deg)"] items=["ζ", "τ1", "τS", "τN", "τC", "κ0", "m1", "m2", "m3", "T (K)", "B (T)", "θ (deg)"]
            n291 = local read "ζ"() -> (w533:dbl)
            n292 = local read "T1"() -> (w532:dbl)
            n293 = local read "τS"() -> (w531:dbl)
            n294 = local read "τN"() -> (w530:dbl)
            n295 = local read "τC"() -> (w529:dbl)
            n296 = local read "κ0"() -> (w528:dbl)
            n297 = local read "T (K)"() -> (w523:dbl)
            n298 = local read "B (T)"() -> (w522:dbl)
            n299 = local read "θ (deg)"() -> (w521:dbl)
            n300 = Build Array(w533, w532, w531, w530, w529, w528, w524, w524, w524, w523, w522, w521) -> (w520:dbl[])
            n301 = Generate User Event(user event=w534, event data cluster="action: replot colors" ("event data")) -> ()  [unwired: 2 in, 2 out]
            n302 = for {
              tunnel: w520 -> [w536] mode=indexing
              tunnel: w519 -> [w537] mode=indexing
              tunnel: [w537] -> w518 mode=indexing
              shift-right: [w538] -> w516
              shift-left: map{T1, dbl} {} ("Map") -> [w539]
              n303 = Insert Into Map(map in=w539, key=w537, value=w536) -> (map out=w538:map{T1, dbl})  [unwired: 2 out]
            }
            n304 = local read "mathematica thing"() -> (w527:map{i32, map{T1, dbl}})
            n305 = local read "file index"() -> (w526:i32)
            n306 = call "3-lorentzian-heat-response -- V4.vi"("action"=3-lorentzian-heat-response_action."calc m1m2m3", "Map IN"=w516) -> ("Map OUT"=w515:map{T1, dbl})  [unwired: 7 in, 2 out]
            n307 = in-place {
              in-place-border: w518 -> [w544]
              in-place-border: w515 -> [w540]
              n308 = in-place-map #2(w527, w526) -> (w543:map{T1, dbl})  [unwired: 1 in, 1 out]
              n309 = for {
                tunnel: w544 -> [w546] mode=indexing
                shift-right: [w548] -> w542
                shift-left: w543 -> [w549]
                shift-right: [w547] -> _
                shift-left: w540 -> [w547]
                n310 = Look In Map(map=w547, key=w546) -> (value=w545:dbl)  [unwired: 1 in, 1 out]
                n311 = Insert Into Map(map in=w549, key=w546, value=w545) -> (map out=w548:map{T1, dbl})  [unwired: 2 out]
              }
              n312 = in-place-map #2(w542, LVMapReplaceAction."Modify Entry only if found" ("action")) -> (w525:map{i32, map{T1, dbl}})  [unwired: 2 out]
            }
            n313 = local write "mathematica thing"(w525) -> ()
          }
          frame "action: exit" {
          }
          frame "action: read from file" {
            n314 = call "file - read-write - list of lines.vi"("read/write control"=file_--_read-write_control."read", "file path"="Read from file") -> ("list of lines OUT"=w591:string[], "filename out"=w584:string)  [unwired: 7 in, 1 out]
            n315 = local read "cursor x selector"() -> (w560:map{T1, dbl})
            n316 = for {
              tunnel: w591 -> [w625] mode=indexing
              tunnel: [w620] -> w568 mode=indexing if=w616
              tunnel: [w619] -> w587 mode=indexing if=w616
              w621 = 0.0
              n317 = Scan From String(format string="%f%f%f", input string=w625, initial scan location=u32 0, default 1=w621, default 2=w621, default 3=w621) -> (offset past scan=w617:u32, output 1=w619:dbl, output 2=w623:dbl, output 3=w622:dbl)  [unwired: 1 in, 2 out]
              n318 = Greater Than 0?(x=w617) -> (x > 0?=w616:bool)
              n319 = Re/Im To Complex(1:w622, 2:w623) -> (0:w620:cdb)
            }
            n320 = call "filename-manage.vi"("filename-action"=filename-action."get name", "file name IN"=w584) -> ("string OUT"=w581:string)  [unwired: 7 in, 2 out]
            n321 = call "filename-manage.vi"("filename-action"=filename-action."get T", "file name IN"=w581) -> ("number OUT"=w559:dbl, "filename OUT"=w580:string)  [unwired: 7 in, 1 out]
            "T (K)" <- w559
            n322 = Unbundle("off\nRe\nIm") -> ("Numeric"=w564:dbl, "Numeric"=w563:dbl)
            n323 = Re/Im To Complex(1:w563, 2:w564) -> (0:w567:cdb)
            n324 = Insert Into Map(map in=w560, key=3-lorentzian-parameters."T (K)" ("Plost: sweep window"), value=w559) -> (map out=w558:map{T1, dbl})  [unwired: 2 out]
            n325 = Subtract(x=w568, y=w567) -> (x-y=w566:cdb[])
            n326 = call "filename-manage.vi"("filename-action"=filename-action."get deg", "file name IN"=w580) -> ("number OUT"=w555:dbl, "filename OUT"=w570:string)  [unwired: 7 in, 1 out]
            "θ (deg)" <- w555
            n327 = Generate User Event(user event=w588, event data cluster="action: new sweep" ("event data")) -> ()  [unwired: 2 in, 2 out]
            n328 = case shown="\"add - ω\"" "tr" {
              tunnel: w566 -> [w592 w594 w606]
              tunnel: w587 -> [w593 w601 w615]
              tunnel: [w593 w598 w612] -> w577
              tunnel: [w592 w597 w611] -> w569
              frame "as is", Default {
              }
              frame "add - ω" {
                n329 = call "array -- freq-voltage transformations.vi"("freq voltage action"=array_--_freq-voltage_transformations_action."add -ω", "z In"=w594, "ω IN"=w601) -> ("z out"=w599:cdb[], "ω out"=w600:dbl[])  [unwired: 7 in]
                n330 = call "array -- freq-voltage transformations.vi"("freq voltage action"=array_--_freq-voltage_transformations_action."sort ω", "z In"=w599, "ω IN"=w600) -> ("z out"=w597:cdb[], "ω out"=w598:dbl[])  [unwired: 7 in]
              }
              frame "full rydh" {
                n331 = call "array -- freq-voltage transformations.vi"("freq voltage action"=array_--_freq-voltage_transformations_action."2 x ω", "z In"=w606, "ω IN"=w615) -> ("z out"=w605:cdb[], "ω out"=w608:dbl[])  [unwired: 7 in]
                n332 = call "array -- freq-voltage transformations.vi"("freq voltage action"=array_--_freq-voltage_transformations_action."R-phase(deg) to Re-Im", "z In"=w605, "ω IN"=w608) -> ("z out"=w604:cdb[], "ω out"=w607:dbl[])  [unwired: 7 in]
                n333 = call "array -- freq-voltage transformations.vi"("freq voltage action"=array_--_freq-voltage_transformations_action."add -ω", "z In"=w604, "ω IN"=w607) -> ("z out"=w613:cdb[], "ω out"=w614:dbl[])  [unwired: 7 in]
                n334 = call "array -- freq-voltage transformations.vi"("freq voltage action"=array_--_freq-voltage_transformations_action."sort ω", "z In"=w613, "ω IN"=w614) -> ("z out"=w611:cdb[], "ω out"=w612:dbl[])  [unwired: 7 in]
              }
            }
            n335 = Insert Into Map(map in=w558, key=3-lorentzian-parameters."θ (deg)" ("Plost: sweep window"), value=w555) -> (map out=w557:map{T1, dbl})  [unwired: 2 out]
            n336 = call "filename-manage.vi"("filename-action"=filename-action."get ind", "file name IN"=w570) -> ("number OUT"=→"file index":dbl, "filename OUT"=w562:string)  [unwired: 7 in, 1 out]
            n337 = call "filename-manage.vi"("filename-action"=filename-action."get B", "file name IN"=w562) -> ("number OUT"=w554:dbl)  [unwired: 7 in, 2 out]
            "B (T)" <- w554
            n338 = Insert Into Map(map in=w557, key=3-lorentzian-parameters."B (T)" ("Plost: sweep window"), value=w554) -> (map out=w556:map{T1, dbl})  [unwired: 2 out]
            n339 = call "filter - complex - four.vi"("omega  in"=w577, "z in"=w569, "span"="cspan") -> ("omega out"=w576:dbl[], "z out"=w575:cdb[], "dz/domega out"=w574:cdb[])  [unwired: 9 in, 5 out]
            n340 = local write "cursor x selector"(w556) -> ()
            n341 = call "nanocal -- publish -- freq scan V2.vi"("publisher action"=publisher_action."set", "dz/dω IN (V)"=w574, "z IN (V)"=w575, "ω IN (Hz)"=w576) -> ()  [unwired: 5 in, 3 out]
          }
          frame "action: save freq scan" {
            n342 = local read "Freq sweep name template"() -> (w631:T8)
            n343 = call "MFLI -- publish -- freq scan.vi"("publisher action"=publisher_action."get") -> ("Voltage out (V)"=w627:cdb[], "Freq out (Hz)"=w628:dbl[])  [unwired: 9 in]
            n344 = call "filename-manage.vi"("filename pattern"=w631, "filename-action"=filename-action."uniquenum", "folder IN"="Save folder", "file name IN"="freq sweep file name") -> ("filename OUT"=w630:string)  [unwired: 5 in, 2 out]
            n345 = call "KM_appendline -- freq sweep.vi"("freq"=w628, "Vout(V)"=w627, "Save frequency scan"="Save folder", "read/write control"=KM_file_--_read-write_control."append one line", "name or relative path"=w630) -> ()  [unwired: 15 in]
            n346 = local write "freq sweep file name"(w630) -> ()
          }
          frame "void", Default {
          }
        }
      }
    }
  }
  n347 = call "replace cursor - plot ref - V2.vi"("Plot ref in"=w11, "new X"=w10, "new  Y"=w10, "cursor index"=2, "cursor action"=cursor_action."write") -> ()  [unwired: 11 in, 4 out]
  n348 = local write "newton pause"(w7) -> ()
  n349 = control-ref of="Plot:  colors"() -> (w8:refnum<vi>)
  n350 = while "interface" {
    tunnel: w25 -> [w639]
    tunnel: w14 -> [w638]
    tunnel: w11 -> [w636]
    tunnel: w8 -> [w635]
    tunnel: w7 -> [_]
    stop <- w637 stop-if-true
    n351 = event shown="[23] <interface>: User Event" {
      selector: w639 -> [_ _ _ _ _ _ _ _ _ _ _ _ _ _ _ _ _ _ _ _ _ _ _ _]
      dyn-events: _ -> [_ _ _ _ _ _ _ _ _ _ _ _ _ _ _ _ _ _ _ _ _ _ _ _]
      timeout: _ -> [_ _ _ _ _ _ _ _ _ _ _ _ _ _ _ _ _ _ _ _ _ _ _ _]
      tunnel: w638 -> [w640 _ w652 w654 _ w683 w685 w688 w693 w694 w696 w698 w701 _ w707 w747 _ w775 w778 w781 w784 w787 w797 _]
      tunnel: [_ _ _ _ _ _ _ _ "load! :l" _ _ _ _ _ _ _ _ _ _ _ _ _ _ _] -> _
      tunnel: [_ _ _ _ _ _ _ _ _ _ _ _ _ _ _ _ _ _ _ _ _ _ _ w801] -> w637
      tunnel: [_ _ _ _ _ "go!" _ _ _ _ _ _ "parse! :p" _ _ _ "pause!" "uco! :u" "math -->   τ's !" "τ's --> math!" "math --> string!" "string --> math!" _ _] -> _
      tunnel: w636 -> [_ _ _ _ _ _ _ _ _ _ _ _ _ _ w703 _ _ _ _ _ _ _ _ _]
      tunnel: w635 -> [_ _ _ _ _ _ _ _ _ _ _ _ _ _ _ w770 _ _ _ _ _ _ _ _]
      event "Plot: sweep window": Cursor Move {
        n352 = event-data() -> ("CursIdx"=w641:i32)  [unwired: 1 in]
        n353 = case shown="0..2" w641 {
          tunnel: w640 -> [w643 _]
          frame 0..2 {
            w642 = "action: fit"  # action
            n354 = Generate User Event(user event=w643, event data cluster=w642) -> ()  [unwired: 2 in, 2 out]
          }
          frame 3..5, Default {
          }
        }
      }
      event "scale gauge: Plot: complex plane": Value Change {
        n355 = event-data() -> ()  [unwired: 1 in, 1 out]
        n356 = local read "scale gauge: Plot: complex plane"() -> (w650:dbl)
        n357 = control-ref of="Plot: sweep window"() -> (w649:refnum<vi>)
        n358 = Multiply(x=w650, y=0.3) -> (x*y=w651:dbl)
        n359 = Bundle By Name(cluster=T21 {"window y"=0.0021014740628288917, "center x"=44850.89441339177, "center y"=2.5658109925320947, "window x"=17480.201988350764} ("window IN"), "window x"=w650, "window y"=w650, "center x"=w651, "center y"=0.0) -> (w648:T21)
        n360 = call "replace cursor - plot ref - V2.vi"("Plot ref in"=w649, "window IN"=w648, "cursor action"=cursor_action."zoom to win") -> ()  [unwired: 13 in, 4 out]
      }
      event "ζ", "T1", "τS", "τN", "τC", "κ0": Value Change {
        n361 = event-data() -> ()  [unwired: 1 in, 1 out]
        n362 = Generate User Event(user event=w652, event data cluster="action: new sweep" ("event data")) -> ()  [unwired: 2 in, 2 out]
      }
      event Value Change {
        n363 = event-data() -> ()  [unwired: 1 in, 6 out]
        n364 = Generate User Event(user event=w654, event data cluster="action: update enums" ("event data")) -> ()  [unwired: 2 in, 2 out]
      }
      event "ω0 (rad/sec)": Value Change {
        n365 = event-data() -> ()  [unwired: 1 in, 1 out]
        n366 = call "nanocal -- publish -- freq scan V2.vi"("publisher action"=publisher_action."get") -> ("z out (V)"=w681:cdb[], "ω out (Hz)"=w676:dbl[])  [unwired: 8 in, 1 out]
        n367 = control-ref of="Plot: sweep window"() -> (w663:refnum<vi>)
        n368 = local read "T1"() -> (w665:dbl)
        n369 = local read "τN"() -> (w667:dbl)
        n370 = local read "ζ"() -> (w664:dbl)
        n371 = local read "τS"() -> (w666:dbl)
        n372 = local read "τC"() -> (w668:dbl)
        n373 = local read "κ0"() -> (w669:dbl)
        n374 = Divide(x="ω0 (rad/sec)", y=6.283185307179586) -> (x/y=w674:dbl)
        n375 = call "3-lorentzian-heat-response.vi"("zeta"=w664, "T1"=w665, "tauS"=w666, "tauN"=w667, "tauC"=w668, "kappa0"=w669, "omega (rad/sec)"="ω0 (rad/sec)", "action"=3-lorentzian-heat-response_action."calc R") -> ("Romega"=w672:cdb)  [unwired: 7 in, 4 out]
        n376 = Complex To Re/Im(x + iy=w672) -> (x=w670:dbl, y=w671:dbl)
        n377 = Threshold 1D Array(2:w674, 3:w676) -> (0:w675:dbl)  [unwired: 1 in]
        n378 = call "replace cursor - plot ref - V2.vi"("Plot ref in"=w663, "new X"=w670, "new  Y"=w671, "cursor index"=0, "cursor action"=cursor_action."write") -> ("Plot ref out"=w677:refnum<vi>)  [unwired: 11 in, 3 out]
        n379 = Index Array(array=w681, index=w675) -> (element=w678:cdb)
        n380 = Complex To Re/Im(x + iy=w678) -> (x=w679:dbl, y=w680:dbl)
        n381 = call "replace cursor - plot ref - V2.vi"("Plot ref in"=w677, "new X"=w679, "new  Y"=w680, "cursor index"=1, "cursor action"=cursor_action."write") -> ()  [unwired: 11 in, 4 out]
      }
      event "go!": Value Change {
        n382 = event-data() -> ()  [unwired: 1 in, 6 out]
        n383 = Generate User Event(user event=w683, event data cluster="action: gradient step" ("event data")) -> ()  [unwired: 2 in, 2 out]
      }
      event "select B (T)", "select θ (deg)", "ignore T !", "select T (T)", "ignore B !", "ignore θ !": Value Change {
        n384 = event-data() -> ()  [unwired: 1 in, 6 out]
        n385 = Generate User Event(user event=w685, event data cluster="action: replot colors" ("event data")) -> ()  [unwired: 2 in, 2 out]
      }
      event "Plot: sweep window": Cursor Release {
        n386 = event-data() -> ("CursIdx"=w687:i32)  [unwired: 1 in, 8 out]
        n387 = case shown="0..2" w687 {
          tunnel: w688 -> [_ w689]
          frame 3, Default {
          }
          frame 0..2 {
            w690 = "action: fit"  # event data
            n388 = Generate User Event(user event=w689, event data cluster=w690) -> ()  [unwired: 2 in, 2 out]
          }
        }
      }
      event "load! :l": Value Change {
        n389 = event-data() -> ()  [unwired: 1 in, 6 out]
        n390 = Generate User Event "action User Event"(user event=w693, event data cluster="action: read from file" ("event data")) -> ()  [unwired: 2 in, 2 out]
      }
      event "Read from file": Value Change {
        n391 = event-data() -> ()  [unwired: 1 in, 6 out]
        n392 = Generate User Event "action User Event"(user event=w694, event data cluster="action: read from file" ("event data")) -> ()  [unwired: 2 in, 2 out]
      }
      event "off\nRe\nIm": Value Change {
        n393 = event-data() -> ()  [unwired: 1 in, 6 out]
        n394 = Generate User Event "action User Event"(user event=w696, event data cluster="action: read from file" ("event data")) -> ()  [unwired: 2 in, 2 out]
      }
      event "cspan": Value Change {
        n395 = event-data() -> ()  [unwired: 1 in, 6 out]
        n396 = Generate User Event "action User Event"(user event=w698, event data cluster="action: read from file" ("event data")) -> ()  [unwired: 2 in, 2 out]
      }
      event "parse! :p": Value Change {
        n397 = event-data() -> ()  [unwired: 1 in, 6 out]
        n398 = Generate User Event "action User Event"(user event=w701, event data cluster="action: parse string" ("event data")) -> ()  [unwired: 2 in, 2 out]
      }
      event Value Change {
        n399 = event-data() -> ()  [unwired: 1 in, 1 out]
      }
      event Key Down {
        n400 = event-data() -> ("Char"=w705:i16, "VKey"=w708:T22)  [unwired: 1 in]
        n401 = Build Array(w705) -> (w706:i16[])
        n402 = Byte Array To String(unsigned byte array=w706) -> (string=w704:string)
        n403 = case shown="\"ASCII\", Default" w708 {
          selector: w708 -> [_ _ _ _ _ w740]
          tunnel: w707 -> [w711 _ _ w736 _ _]
          tunnel: w704 -> [w710 _ _ _ _ _]
          tunnel: w703 -> [w709 _ _ _ _ w739]
          frame "ASCII", Default {
            n404 = case shown="\"+\", \",\", \"-\", \".\", \"<\", \"=\", \">\"" w710 {
              selector: w710 -> [_ _ _ _ _ _ w723 _ _ _ _]
              tunnel: w711 -> [_ _ w712 w714 w717 _ _ _ w730 w732 w734]
              tunnel: w709 -> [_ _ _ _ _ w721 _ _ _ _ _]
              frame "0", Default {
              }
              frame "a" {
              }
              frame "s" {
                n405 = Generate User Event(user event=w712, event data cluster="action: save freq scan" ("event data")) -> ()  [unwired: 2 in, 2 out]
              }
              frame "l" {
                n406 = Generate User Event(user event=w714, event data cluster="action: read from file" ("event data")) -> ()  [unwired: 2 in, 2 out]
              }
              frame " " {
                n407 = Generate User Event(user event=w717, event data cluster="action: gradient step" ("event data")) -> ()  [unwired: 2 in, 2 out]
              }
              frame "?" {
                # "?"
                n408 = call "replace cursor - plot ref - V2.vi"("Plot ref in"=w721, "cursor action"=cursor_action."zoom to win") -> ("Plot ref out"=w720:refnum<vi>)  [unwired: 14 in, 3 out]
                n409 = call "replace cursor - plot ref - V2.vi"("Plot ref in"=w720, "cursor action"=cursor_action."smart zoom out&aspect") -> ()  [unwired: 14 in, 4 out]
              }
              frame "+", ",", "-", ".", "<", "=", ">" {
                n410 = local read "gradient factor"() -> (w725:dbl)
                n411 = case shown="\"0\", Default" w723 {
                  tunnel: [0.7 1.0 1.5] -> w722
                  frame ",", "-", "<" {
                  }
                  frame "0", Default {
                  }
                  frame "+", ".", "=", ">" {
                  }
                }
                n412 = Multiply(x=w722, y=w725) -> (x*y=w724:dbl)
                n413 = local write "gradient factor"(w724) -> ()
              }
              frame "b" {
                n414 = local read "String"() -> (w729:string)
                n415 = local write "backup string :b"(w729) -> ()
              }
              frame "u" {
                n416 = Generate User Event(user event=w730, event data cluster="ignoreaction: uco" ("event data")) -> ()  [unwired: 2 in, 2 out]
              }
              frame "p" {
                n417 = Generate User Event "action User Event"(user event=w732, event data cluster="action: parse string" ("event data")) -> ()  [unwired: 2 in, 2 out]
              }
              frame "m" {
                n418 = Generate User Event "action User Event"(user event=w734, event data cluster="action: copy from math" ("event data")) -> ()  [unwired: 2 in, 2 out]
              }
            }
          }
          frame "Escape" {
          }
          frame "PageUp" {
          }
          frame "Enter" {
            n419 = Generate User Event "action User Event"(user event=w736, event data cluster="action: replot colors" ("event data")) -> ()  [unwired: 2 in, 2 out]
            n420 = Generate User Event "action User Event"(user event=w736, event data cluster="action: new sweep" ("event data")) -> ()  [unwired: 2 in, 2 out]
          }
          frame "PageDown" {
          }
          frame "Up".."Right" {
            n421 = case shown="\"Down\"" w740 {
              tunnel: [cursor_action."zoom in 20%" ("cursor action") cursor_action."zoom out 20%" ("cursor action") cursor_action."zoom out 20%" ("cursor action") cursor_action."zoom in 20%" ("cursor action")] -> w741
              frame "Up", Default {
              }
              frame "Down" {
              }
              frame "Left" {
              }
              frame "Right" {
              }
            }
            n422 = call "replace cursor - plot ref - V2.vi"("Plot ref in"=w739, "cursor action"=w741) -> ()  [unwired: 14 in, 4 out]
          }
        }
      }
      event "Plot:  colors": Cursor Move {
        n423 = event-data() -> ("CursIdx"=w749:i32)  [unwired: 1 in]
        n424 = local read "T1"() -> (w765:dbl)
        n425 = local read "τS"() -> (w766:dbl)
        n426 = local read "τN"() -> (w767:dbl)
        n427 = local read "τC"() -> (w768:dbl)
        n428 = local read "κ0"() -> (w769:dbl)
        n429 = local read "ζ"() -> (w764:dbl)
        n430 = call "replace cursor - plot ref - V2.vi"("Plot ref in"=w770, "cursor index"=w749, "cursor action"=cursor_action."read") -> ("read Y"=w748:dbl)  [unwired: 13 in, 3 out]
        n431 = Build Array(w764, w765, w766, w767, w768, w769) -> (w751:dbl[])
        n432 = Replace Array Subset(array=w751, new element=w748, index=w749) -> (w750:dbl[])
        n433 = Generate User Event(user event=w747, event data cluster="action: replot circles" ("event data")) -> ()  [unwired: 2 in, 2 out]
        n434 = Index Array(array=w750, index #1=0 ("index"), index #2=1 ("index"), index #3=2 ("index"), index #4=3 ("index"), index #5=4 ("index"), index #6=5 ("index")) -> (element #1=w757:dbl, element #2=w756:dbl, element #3=w755:dbl, element #4=w754:dbl, element #5=w753:dbl, element #6=w752:dbl)
        n435 = local write "τN"(w754) -> ()
        n436 = local write "τC"(w753) -> ()
        n437 = local write "τS"(w755) -> ()
        n438 = local write "κ0"(w752) -> ()
        n439 = local write "T1"(w756) -> ()
        n440 = local write "ζ"(w757) -> ()
      }
      event "pause!": Value Change {
        n441 = event-data() -> ()  [unwired: 1 in, 6 out]
        n442 = local write "newton pause"(TRUE ("newton pause")) -> ()
      }
      event "uco! :u": Value Change {
        n443 = event-data() -> ()  [unwired: 1 in, 1 out]
        n444 = Generate User Event(user event=w775, event data cluster="ignoreaction: uco" ("event data")) -> ()  [unwired: 2 in, 2 out]
      }
      event "math -->   τ's !": Value Change {
        n445 = event-data() -> ()  [unwired: 1 in, 1 out]
        n446 = Generate User Event(user event=w778, event data cluster="action: copy from math" ("event data")) -> ()  [unwired: 2 in, 2 out]
      }
      event "τ's --> math!": Value Change {
        n447 = event-data() -> ()  [unwired: 1 in, 1 out]
        n448 = Generate User Event(user event=w781, event data cluster="action: copy to math" ("event data")) -> ()  [unwired: 2 in, 2 out]
      }
      event "math --> string!": Value Change {
        n449 = event-data() -> ()  [unwired: 1 in, 1 out]
        n450 = Generate User Event(user event=w784, event data cluster="action: write mathematica string" ("event data")) -> ()  [unwired: 2 in, 2 out]
      }
      event "string --> math!": Value Change {
        n451 = event-data() -> ()  [unwired: 1 in, 1 out]
        n452 = Generate User Event(user event=w787, event data cluster="action: read mathematica string" ("event data")) -> ()  [unwired: 2 in, 2 out]
      }
      event "filenames": Value Change {
        n453 = event-data() -> ()  [unwired: 1 in, 6 out]
        n454 = local read "filesnames lookup"() -> (w795:map{i32, i32})
        n455 = local read "filenames"() -> (w793:map{i32, string})
        n456 = local read "filenames"() -> (w794:u16)
        n457 = local read "folder"() -> (w796:path)
        n458 = Look In Map(map=w795, key=w794) -> (value=w792:i32)  [unwired: 1 in, 1 out]
        n459 = Look In Map(map=w793, key=w792) -> (value=w791:string)  [unwired: 1 in, 1 out]
        n460 = Build Path(base path=w796, name or relative path=w791) -> (appended path=w789:path)
        n461 = for {
          N: 1 -> [_]
          tunnel: w797 -> [w799]
          tunnel: w789 -> [w798]
          n462 = local write "Read from file"(w798) -> ()
          n463 = Generate User Event(user event=w799, event data cluster="action: read from file" ("event data")) -> ()  [unwired: 2 in, 2 out]
        }
      }
      event User Event {
        n464 = event-data() -> ("interface"=w802:string)  [unwired: 1 in, 4 out]
        n465 = case shown="\"interface: update color cursors\"" w802 {
          tunnel: [_ _ TRUE] -> w801
          frame "void", Default {
          }
          frame "interface: update color cursors" {
            w806 = T1[] [enum."T (K)", enum."B (T)", enum."θ (deg)"] items=["ζ", "τ1", "τS", "τN", "τC", "κ0", "m1", "m2", "m3", "T (K)", "B (T)", "θ (deg)"]
            w803 = T1[] [enum."ζ", enum."τ1", enum."τS", enum."τN", enum."τC", enum."κ0", enum."m1", enum."m2", enum."m3"] items=["ζ", "τ1", "τS", "τN", "τC", "κ0", "m1", "m2", "m3", "T (K)", "B (T)", "θ (deg)"]
            n466 = local read "T1"() -> (w814:dbl)
            n467 = local read "τS"() -> (w815:dbl)
            n468 = local read "τN"() -> (w816:dbl)
            n469 = local read "τC"() -> (w817:dbl)
            n470 = local read "κ0"() -> (w818:dbl)
            n471 = local read "ζ"() -> (w813:dbl)
            n472 = Build Array(w813, w814, w815, w816, w817, w818) -> (w820:dbl[])
            n473 = for {
              shift-right: [w836] -> w821
              shift-left: map{T1, dbl} {} ("Map IN") -> [w837]
              tunnel: w803 -> [w834] mode=indexing
              tunnel: w820 -> [w835] mode=indexing
              tunnel: [w834] -> w829 mode=indexing
              n474 = Insert Into Map(map in=w837, key=w834, value=w835) -> (map out=w836:map{T1, dbl})  [unwired: 2 out]
            }
            n475 = call "3-lorentzian-heat-response -- V4.vi"("action"=3-lorentzian-heat-response_action."calc m1m2m3", "Map IN"=w821) -> ("Map OUT"=w825:map{T1, dbl})  [unwired: 7 in, 2 out]
            n476 = local read "θ (deg)"() -> (w824:dbl)
            n477 = local read "B (T)"() -> (w823:dbl)
            n478 = local read "T (K)"() -> (w822:dbl)
            n479 = local read "cursor x selector"() -> (w809:map{T1, dbl})
            n480 = Build Array(w822, w823, w824) -> (w826:dbl[])
            n481 = local read "X selector"() -> (w810:T1)
            n482 = local read "cursor index map"() -> (w819:map{T1, i32})
            n483 = local read "T (K)"() -> (w811:dbl)
            n484 = for {
              shift-right: [w832] -> w827
              shift-left: w825 -> [w833]
              tunnel: w806 -> [w831] mode=indexing
              tunnel: w826 -> [w830] mode=indexing
              n485 = Insert Into Map(map in=w833, key=w831, value=w830) -> (map out=w832:map{T1, dbl})  [unwired: 2 out]
            }
            n486 = control-ref of="Plot:  colors"() -> (w808:refnum<vi>)
            n487 = Look In Map(map=w809, key=w810, default value=w811) -> (value=w812:dbl)  [unwired: 1 out]
            n488 = for {
              tunnel: w812 -> [w845]
              tunnel: w808 -> [w844]
              tunnel: w829 -> [w840] mode=indexing
              tunnel: w819 -> [w842]
              shift-right: [w839] -> _
              shift-left: w825 -> [w839]
              n489 = Look In Map(map=w839, key=w840) -> (value=w838:dbl)  [unwired: 1 in, 1 out]
              n490 = Look In Map(map=w842, key=w840) -> (value=w841:i32)  [unwired: 1 in, 1 out]
              n491 = call "replace cursor - plot ref - V2.vi"("Plot ref in"=w844, "new X"=w845, "new  Y"=w838, "cursor index"=w841, "cursor action"=cursor_action."write") -> ()  [unwired: 11 in, 4 out]
            }
            n492 = call "string parse mathematica assosiated array.vi"("derivative"=mathematica_string_map_action."create string", "Map IN"=w827) -> ("String OUT"=w828:string)  [unwired: 8 in, 1 out]
            n493 = local write "String"(w828) -> ()
          }
          frame "interface: exit" {
          }
        }
      }
    }
  }
  "cursor x selector" <- w9
